vi "UHR-Fleezers Control (host) - 9.2.vi"() -> ()   [LabVIEW 2009]
uses:
  <vilib>/Utility/miscctls.llb/LVPoint32TypeDef.ctl
  <vilib>/Utility/miscctls.llb/LVMinMaxIncTypeDef.ctl
  <vilib>/userDefined/High Color/nirio_resource_hc.ctl
  <vilib>/Instr/_visa.llb/VISA Configure Serial Port (Instr).vi
  <vilib>/Platform/TimedLoop/XDataNode/XDataNode.xnode
  <vilib>/Platform/TimedLoop/XDataNode/loadlvalarms.vi
  <vilib>/Platform/TimedLoop/XDataNode/timing_clust.ctl
  <vilib>/Platform/TimedLoop/XDataNode/nitl_modes.ctl
  <vilib>/Platform/TimedLoop/XDataNode/wakeup.ctl
  <vilib>/rvi/interface/nirviOpenFPGA/nirviOpenFPGA.xnode
  FPGA Bitfiles/UHR-Fleezers Instr~3C_FPGA Target_UHR-Fleezers Contr~F0.lvbitx
  UHR-Fleezers Control (fpga) - 9.1.vi
  <vilib>/FPGAPlugInAG/PCIe-7852R/nirviIntfOpen_PCIe-7852R.vi
  <vilib>/rvi/interface/nirviMethod/nirviMethod.xnode
  <vilib>/Utility/error.llb/Merge Errors.vi
  <vilib>/LabVIEW Targets/FPGA/Rio/nirio_HostInterface/nirio_Reset.vi
  <vilib>/LabVIEW Targets/FPGA/Rio/nirio_HostInterface/nirio_DMAStopAll.vi
  <vilib>/rvi/interface/common/niFpgaNodeNameForErrorReporting.ctl
  <vilib>/rvi/errors/niLvFpgaWhatHappensToTopLevelVI.ctl
  <vilib>/LabVIEW Targets/FPGA/Rio/nirio_HostInterface/nirio_DisableInterrupts.vi
  <vilib>/Utility/error.llb/Error Cluster From Error Code.vi
  <vilib>/rvi/errors/niLvFpgaAdjustHostInterfaceError.vi
  <vilib>/rvi/interface/nirviReadWriteControl/nirviReadWriteControl.xnode
  <vilib>/LabVIEW Targets/FPGA/Rio/nirio_HostInterface/nirio_WriteBig.vi
  <vilib>/LabVIEW Targets/FPGA/Rio/nirio_HostInterface/nirio_DMAConfigure.vi
  <vilib>/LabVIEW Targets/FPGA/Rio/nirio_HostInterface/nirio_DMAStop.vi
  <vilib>/RVI Host/nirviSupport.llb/nirviErrorClusterFromErrorCode.vi
  <vilib>/LabVIEW Targets/FPGA/Rio/nirio_HostInterface/nirio_EnableInterrupts.vi
  <vilib>/rvi/errors/niLvFpgaReportInternalErrorWithAdditionalInfo.vi
  <vilib>/express/express analysis/Spectral/XNode/ExpressSpectralMeasurementsBlockNode.xnode
  <vilib>/express/express analysis/Spectral/Block/exnSpectralBlock spectral measurements PSD poly.vi
  <vilib>/express/express analysis/Spectral/Block/exnSpectralBlock spectral measurements PSD WFM.vi
  <vilib>/Waveform/WDTOps.llb/WDT Append Waveforms DBL.vi
  <vilib>/LabVIEW Targets/FPGA/Rio/nirio_HostInterface/nirio_ReadBig.vi
  <vilib>/vision/Avi1.llb/AviRefnum.ctl
  <vilib>/rvi/interface/nirviCloseFPGA/nirviCloseFPGA.xnode
  <vilib>/FPGAPlugInAG/PCIe-7852R/nirviIntfClose_PCIe-7852R.vi
  <vilib>/Analysis/NI_AALBase.lvlib
  <vilib>/Platform/TimedLoop/XDataNode/XDNodeRunTimeDep.lvlib
  openfpgaref.8.6.ctl
  NiRioSrv.dll
  <vilib>/vision/NI_Vision_Development_Module.lvlib
panel:
  out "Waveform Graph":dbl[](graph) caption="APD Line Scan"
  in  "Total Volume\nFlushed (uL)":dbl
  in  "Flush Center Channel":bool
  in  "Inject Bottom Channel":bool
  in  "Inject Top Channel":bool
  out "Messages":string
  in  "APD Ave N":dbl=10.0
  out "Int. Time (s)":dbl
  in  "Stop All":bool
  out "sigma/mean":dbl
  out "Rate sigma (Hz)":dbl format="%0.2f"
  out "Current Stage  Position":cluster{dbl, dbl, dbl}
  in  "Index":dbl=1.0 caption="Save File Index" min=1.0 step=1.0
  in  "Tab Control 6":T1(tab)=enum."Dual Display (APD)"
  out "All Signals":waveform(dbl)[](graph)
  in  "Signals to Plot":i32(listbox)
  out "Trap Disp. Freq. (Hz)":dbl caption="Freq. (Hz)" format="%#_6p"
  out "Display Period (s)":dbl caption="Period (s)" format="%#_6p"
  in  "Trap Disp. Downsample":dbl=20000.0 caption="Downsample"
  in  "APD Disp. Scale":dbl=0.1 caption="Scale (Divide,\nfor above plot only)"
  in  "APD Disp. Downsample":dbl=30.0 caption="Integrate" min=1.0 step=1.0
  out "APD Display Freq. (Hz)":dbl caption="Freq. (Hz)"
  out "APD Display Period (s)":dbl caption="Period (s)"
  out "RMS (Ang)":dbl format="%_2g"
  in  "Bead Sep. Int. Time (s)":dbl=5.0 caption="Int. Time (s)"
  in  "Below (kHz)":dbl=0.5
  in  "Above (kHz)":dbl=2.0
  in  "Adjust Scale\nto Mean":bool
  in  "Rescale on Mean":bool
  in  "Offset (nm)":dbl
  out "Mean":dbl caption="Mean (pN)" format="%#_3g"
  out "Force":waveform(dbl)[](graph)
  out "APD 1 Chart":waveform(dbl)(graph)
  in  "Calibration":u16(ring)=2 items=["None", "Position", "Force"]
  out "T1 X":dbl caption="T1 X (pN)" format="%0.2f"
  out "T2 X":dbl caption="T2 X (pN)" format="%0.2f"
  out "Bead Separation":waveform(dbl)(graph)
  in  "Amplitude (nm)":dbl=1.0
  out "Bead Mean (nm)":dbl caption="Mean (nm)" format="%0.2f"
  out "Difference":dbl caption="Difference (pN)" format="%.2g"
  in  "Set X Only":bool
  in  "Set Y Only":bool
  out "Detection Laser X":T2(plugin-control)
  out "APD 1":T2(plugin-control)
  out "Detection Laser Y":T2(plugin-control)
  out "Pointer Y (V)":dbl format="%_3g"
  out "Pointer X (V)":dbl format="%_3g"
  in  "Set Confocal Spot (X-Y)":bool
  out "FFT 1":cluster{"f0":dbl, "df":dbl, "magnitude":dbl[]}[](graph)
  out "FFT 2":cluster{"f0":dbl, "df":dbl, "magnitude":dbl[]}[](graph)
  in  "FFT 1 Choice 1":u16(ring) items=["T1 Y", "T1 X", "T1 Sum", "T2 Y", "T2 X", "T2 Sum", "T1 FB X", "T1 FB Sum", "T2 FB X", "T2 FB Sum", "PSD Y", "PSD X", "PSD Y Sum", "none"]
  in  "FFT 2 Choice 1":u16(ring)=13 items=["T1 Y", "T1 X", "T1 Sum", "T2 Y", "T2 X", "T2 Sum", "T1 FB X", "T1 FB Sum", "T2 FB X", "T2 FB Sum", "PSD Y", "PSD X", "PSD Y Sum", "none"]
  in  "FFT 1 Choice 2":u16(ring)=1 items=["T1 Y", "T1 X", "T1 Sum", "T2 Y", "T2 X", "T2 Sum", "T1 FB X", "T1 FB Sum", "T2 FB X", "T2 FB Sum", "PSD Y", "PSD X", "PSD Y Sum", "none"]
  in  "FFT 2 Choice 2":u16(ring)=13 items=["T1 Y", "T1 X", "T1 Sum", "T2 Y", "T2 X", "T2 Sum", "T1 FB X", "T1 FB Sum", "T2 FB X", "T2 FB Sum", "PSD Y", "PSD X", "PSD Y Sum", "none"]
  in  "Compute FFT":bool
  in  "Reset FFT":bool
  in  "# Spectra to Ave.":dbl=100.0
  out "Ave. Time (s)":dbl
  out "1 Channel":waveform(dbl)(graph)
  out "Slow mean":dbl format="%0.2f"
  in  "Slow mean N ave.":dbl=1.0 min=1.0 step=1.0
  out "Mean Intensity":dbl
  out "Sigma":dbl
  out "Sigma/Mean":dbl
  in  "Subtract mean":bool
  in  "High Res. Display":u16(ring) items=["T1 Y", "T1 X", "T1 Sum", "T2 Y", "T2 X", "T2 Sum", "T1 FB X", "T1 FB Sum", "T2 FB X", "T2 FB Sum", "PSD Y", "PSD X", "PSD Y Sum"]
  out "APD 1 Graph":dbl[](graph) caption="Most Recent Time Trace"
  out "Trap Delta Graph":dbl[](graph) caption="Most Recent Time Trace"
  out "APD 1 Rate (Hz)":dbl format="%#_3p"
  out "Image":u32[][](graph)
  in  "Tab Control":T3(tab)=enum."APD Counting"
  in  "Read Cal":bool
  out "Tether":bool
  in  "Tether Alarm?":bool=TRUE
  in  "Move to Delta (MHz)":dbl=14.5
  in  "Then...":string(combo)="2"
  in  "Data Acq. Spot":bool
  out "Fl. High":bool
  out "Waiting":bool
  in  "Yank to Freq. (MHz)":dbl
  in  "Fl. Threshold (kHz)":dbl
  in  "Fl. Triggered...":bool
  in  "Confocal Linescan":bool
  in  "Speed (nm/s)":dbl=100.0
  in  "Stop F (pN)":dbl=2.0
  in  "Furthest Withdraw (MHz)":dbl=15.0
  in  "Closest Delta (MHz)":dbl=10.25 step=0.25
  in  "Fish for Tether":bool
  in  "Confocal Image":bool
  in  "Round T1 X":bool caption="Round"
  in  "T1 offset_x (mV)":dbl=-26.302542012392074 format="%#_2g"
  in  "T1 kappa_x (pN/nm)":dbl=0.22546432407642192 min=0.0 step=0.001 format="%#_2g"
  out "Time (s)":dbl
  out "Total Time (s)":dbl
  in  "Start Saving":bool
  in  "Limits Enable":bool=TRUE caption="Enable"
  in  "Limit Max (MHz)":dbl=16.0 caption="Max (MHz)"
  in  "Limit Min (MHz)":dbl=10.0 caption="Min (MHz)"
  in  "Cal sets to save":u32=50 min=1 step=1
  in  "Comment (data description)":string="testing confocal setup"
  out "Calibrating Trap...":bool
  in  "Trap 2 (ON/OFF)":bool
  in  "Trap 1 (ON/OFF)":bool
  in  "Save Calibration":bool
  in  "N sets to save":u32=200 caption="N Sets"
  in  "Save N Sets":bool
  out "Save file name":path
  in  "Save ave N":dbl=500.0 caption="Averaging Factor"
  out "Saving...":bool
  in  "Stop Saving":bool
  out "Progress":u16(slide) scale=0.0..100.0
  out "Manipulating Trap":bool
  out "Buffer Status":dbl(slide) scale=0.0..1.0
  out "Overflow (data lost)":bool
  in  "Reset":bool
  out "Data Rate (Hz)":dbl caption="Trap Data Rate (Hz)" format="%#_3p"
  out "Data Period (s)":dbl caption="Trap Data Period (s)" format="%#_6p"
  out "Save Data Rate (Hz)":dbl caption="Rate (Hz)" format="%#_6p"
  out "Save Data Period (s)":dbl caption="Period (s)" format="%#_6p"
  in  "T1 alpha_x (nm/V)":dbl=630.439304367558 step=10.0 format="%#_3g"
  in  "T2 alpha_x (nm/V)":dbl=704.7738222964198 step=10.0 format="%#_3g"
  in  "T2 kappa_x (pN/nm)":dbl=0.2030110880477556 min=0.0 step=0.001 format="%#_2g"
  in  "T2 offset_x (mV)":dbl=-26.67973517613748 format="%#_2g"
  in  "BD 1 Frequency 1 (MHz)":dbl=70.5 caption="T1 X (MHz)" min=60.0 max=90.0 step=1.0 format="%#_6p"
  in  "BD 1 Frequency 2 (MHz)":dbl=85.0 caption="T2 X (MHz)" min=60.0 max=90.0 step=1.0 format="%#_6p"
  in  "Green Laser ON/Interlacing":bool
  in  "Round T2 X":bool caption="Round"
  in  "AO1":dbl(slide)=5.47 caption="Confocal Y (V)" min=0.0 max=10.0 step=0.01 scale=0.0..10.0 scale format="%_1f"
  in  "AO2":dbl(slide)=4.15 caption="Confocal X (V)" min=0.0 max=10.0 step=0.01 scale=0.0..10.0 scale format="%_1f"
  in  "Upper Cap.":bool
  in  "Lower Cap.":bool
  in  "Trap Raster Scan":bool
  out "Raster Scanning...":bool
  in  "Trap Delta (MHz)":dbl=14.5
  in  "Action":string(combo)="Alarm"
  in  "Dump Beads":bool
  out "Duration (s)":dbl
  out "Stage Moving":bool
  in  "Wait Before Save (s)":u32=1
  out "Attempts":dbl
  in  "Attempt Limit":dbl=20.0 caption="Limit"
  in  "z nudge increment (um)":dbl=0.5
  in  "+z":bool
  in  "Saved Stage Positions":T4={"Position 1"={1.35171, -1.39824, -0.01733}, "Position 2"={0.0, 0.0, 0.0}, "Position 3"={2.99911, -0.2477, 0.0}, "Position 4"={2.1058, 0.57485, 0.0}} {"Position 1"."?" min=-0.1 max=0.1 step=0.1; "Position 2"."?" min=-0.1 max=0.1 step=0.1; "Position 3"."?" min=-0.1 max=0.1 step=0.1; "Position 4"."?" min=-0.1 max=0.1 step=0.1}
  in  "Position 1 Label":string="Upper capillary"
  in  "Set Position 1":bool
  in  "Set Position 2":bool
  in  "Set Position 3":bool
  in  "Set Position 4":bool
  in  "Move to Position 3":bool
  in  "Move to Position 4":bool
  in  "Move to Position 2":bool
  in  "Move to Position 1":bool
  in  "Position 2 Label":string="Lower capillary"
  in  "Position 3 Label":string="Measurement Spot"
  in  "Position 4 Label":string="Dump beads"
  in  "-z":bool
  in  "Top Ch Inject Rate (ul/h)":dbl=10.0
  in  "Pump write delay (ms)":dbl=300.0
  in  "All Pump Parameters":T5={"Pump 1"={"Diameter (mm)"=4.61, "Units"=3.0, "Volume"=0.0, "Rate"=0.0}, "Pump 2"={"Diameter (mm)"=4.61, "Units"=3.0, "Volume"=0.0, "Rate"=0.0}, "Pump 3"={"Diameter (mm)"=4.61, "Units"=3.0, "Volume"=0.0, "Rate"=0.0}}
  in  "Top Ch Inject Volume (uL)":dbl=100.0
  in  "Pump pause delay (ms)":u32
  in  "Bottom Ch Inject Volume (uL)":dbl=100.0
  in  "Bottom Ch Inject Rate (ul/h)":dbl=10.0
  in  "Flush Center Ch Volume (uL)":dbl=15.0
  in  "Flush Center Ch Rate (ul/m)":dbl=100.0
  in  "Tab Control 2":T6(tab)=enum."AOD Raster Scan"
  out "Total Counts (ticks)":u32
  in  "Trap ON/OFF X or Y Amp?":bool=TRUE
  in  "Oscillate Set 1":bool
  in  "Trap 1 ON":bool
  in  "Number Interlace Sets":u8=3 min=1 max=3
  in  "DIO count 3 (ticks)":u32=200
  in  "DIO count 2 (ticks)":u32=200
  in  "DIO count 1 (ticks)":u32=200
  in  "BD 2 Amplitude 3 (%)":dbl min=0.0 max=50.0 step=1.0
  in  "BD 2 Amplitude 2 (%)":dbl min=0.0 max=50.0 step=1.0
  in  "BD 2 Amplitude 1 (%)":dbl min=0.0 max=50.0 step=1.0
  in  "BD 1 Amplitude 3 (%)":dbl min=0.0 max=50.0 step=1.0
  in  "BD 1 Amplitude 2 (%)":dbl=35.0 min=0.0 max=50.0 step=1.0
  in  "BD 1 Amplitude 1 (%)":dbl=10.0 min=0.0 max=50.0 step=1.0
  in  "BD 2 Frequency 3 (MHz)":dbl=26.0 min=0.0 max=40.0 step=1.0 format="%#_6p"
  in  "BD 1 Frequency 3 (MHz)":dbl=70.0 min=60.0 max=90.0 step=1.0 format="%#_6p"
  in  "BD 2 Frequency 2 (MHz)":dbl=26.0 min=0.0 max=40.0 step=1.0 format="%#_6p"
  in  "BD 2 Frequency 1 (MHz)":dbl=26.0 min=0.0 max=40.0 step=1.0 format="%#_6p"
  in  "Not-Interlacing Set":enum32{"Set 1", "Set 2", "Set 3"}(radio)
  in  "Interlace":bool=TRUE
  in  "Trap 2 ON":bool
  in  "Trap 3 ON":bool
  in  "Scan axis 2":bool=TRUE
  in  "Osc. freq. (Hz)":dbl=0.25
  in  "Osc. amp. (MHz)":dbl=2.0
  out "Coords":T7
  in  "Manipulation Scaling":cluster{"Horizontal":dbl, "Vertical":dbl}={"Horizontal"=0.075, "Vertical"=0.01}
  in  "Freq or Amp switch first":bool=TRUE
  in  "Swap F1 and F2":bool
  in  "Freq switch delay":u16
  in  "Amp switch delay":u16=5
  in  "MCL Step Increment (V_int)":dbl=3.0
  out "Time to Finish All (min)":dbl format="%#_2p"
  in  "Scan Speed (nm/s)":dbl=100.0
  in  "Scan Range (nm)":dbl=600.0
  in  "Step Size (nm)":dbl=1.0
  in  "MCL/AOM Scale Tweak":dbl=1.0
  in  "MCL Step Position Ratio":dbl=0.5
  in  "Move MCL Also?":bool=TRUE
  out "Final sep (nm)":dbl
  out "Initial sep (nm)":dbl
  out "Save index":dbl
  out "Final delta (MHz)":dbl
  out "Initial delta (MHz)":dbl
  out "Final freq. (MHz)":dbl
  out "Initial freq. (MHz)":dbl
  in  "Saved AOD Raster Scan Parameter Sets":T8(array[cluster])=[{"Scan Range AOD (nm) 2"=500.0, "Step Size AOD (nm) 2"=1.0, "Scan Speed AOD (nm/s) 2"=200.0, "Number of scans (AOD) 2"=1, "Label"=""}, {"Scan Range AOD (nm) 2"=1000.0, "Step Size AOD (nm) 2"=1.0, "Scan Speed AOD (nm/s) 2"=200.0, "Number of scans (AOD) 2"=5, "Label"="wide offset scan"}, {"Scan Range AOD (nm) 2"=20.0, "Step Size AOD (nm) 2"=0.68, "Scan Speed AOD (nm/s) 2"=0.68, "Number of scans (AOD) 2"=1, "Label"="2 bp steps"}]
  in  "Load parameters":bool
  out "Scan Range (MHz)":dbl=10.0
  in  "Restart DMA? (AOD)":bool=TRUE caption="Restart DMA?"
  out "Incr. int (AOD)":i64
  out "Time/Scan (s) (AOD)":dbl format="%#_2p"
  out "Data points/scans":dbl
  out "Data points/scan (f/b)":dbl
  in  "Save scans":bool=TRUE
  out "AOD Scan I":u64 caption="Scan I"
  in  "Continuous AOD Scanning":bool caption="Continuous Scanning"
  in  "Abort AOD Scan":bool caption="Abort Scan"
  in  "Scan BD":bool=TRUE
  out "Cycles/step (AOD)":u64=400 format="%.0p"
  in  "Number of F/B Scans (AOD)":u16=3 min=1
  out "Scan steps (AOD)":u64=1000
  out "Scan Increment (MHz)":dbl=0.2
  out "AOD Scanning":bool caption="Scanning"
  in  "Start AOD Scan":bool caption="Start Scan"
  out "N sets should be saved":dbl
  out "Progress 2":u16(slide) caption="Progress" scale=0.0..100.0
  in  "Abort save 2":bool caption="Abort save"
  in  "Trap 1 Bead Size (nm)":dbl=860.0
  in  "Trap 2 Bead Size (nm)":dbl=790.0
  out "MCL Count":dbl
  in  "All FB On/Off":bool=TRUE
  in  "AI2 to Setpoint":cluster{"Set 1":bool, "Set 2":bool}
  out "AI2 (V)":cluster{"Set 1":dbl, "Set 2":dbl}
  in  "Reset Feedback":cluster{"Set 1":bool, "Set 2":bool}
  in  "PID Gains":T9={"Set 1"={"proportional gain (Kc)"=0, "integral gain (Kc*Ts/Ti)"=5, "derivative gain (Kc*Td/Ts)"=0}, "Set 2"={"proportional gain (Kc)"=0, "integral gain (Kc*Ts/Ti)"=5, "derivative gain (Kc*Td/Ts)"=0}}
  in  "Setpoints (V)":cluster{"Set 1":dbl, "Set 2":dbl}={"Set 1"=7.0, "Set 2"=7.0}
  in  "Feedback On/Off":cluster{"Set 1":bool, "Set 2":bool}={"Set 1"=TRUE, "Set 2"=TRUE}
  in  "Tab Control 3":enum32{"Timing", "MCL Scan", "Analog Out"}(tab)
  out "APD Gate Late Counter":u32
  in  "- phase (APD Gate)":bool
  in  "+ phase (APD Gate)":bool
  out "APD Gate Relative Phase":i16
  in  "Phase Adj. (APD Gate)":i16=20
  in  "Initial Phase Adjustment (APD Gate)":i16=50
  in  "Save APD Data\nwith Trap Data":bool=TRUE
  out "APD FIFO Elements Remaining":u32
  in  "- phase (APD Acq)":bool
  in  "+ phase (APD Acq)":bool
  out "APD Acq Late Counter":u32
  out "APD Acq Relative Phase":i16
  in  "Phase Adj. (APD Acq)":i16=20
  in  "Initial Phase Adjustment (APD Acq)":i16
  in  "Invert APD Gate":bool caption="Invert Gate"
  in  "APD Gate OFF Count":u32=450 caption="Gate OFF Count"
  in  "APD Gate ON Count":u32=150 caption="Gate ON Count"
  in  "APD Gate":enum32{"ON", "OFF", "Interlace"}(radio)=enum."Interlace"
  in  "APD Integration Time (s)":dbl=0.01 caption="Integration Time (s)"
  out "APD Acq Rate (Hz)":dbl=20000000.0 caption="Rate (Hz)"
  out "APD Samples/FIFO Acq.":dbl
  out "APD Elements/DMA read":u32
  out "APD Int. Count":u32 format="%.0p"
  in  "Tab Control 5":enum32{"PSD X", "PSD Y", "Other Data Channel"}(tab)
  out "Data map":dbl[][](graph)
  in  "Channel":i32=4
  in  "Abort MCL Scan":bool
  out "MCL Scan I":u64
  out "MCL Scanning":bool
  in  "Start MCL Scan":bool
  out "wait to reset values":bool
  in  "Tab Control 4":enum32{"Scan Settings", "MCL FPGA Loop Timing"}(tab)=enum."MCL FPGA Loop Timing"
  out "Total Time (s)":dbl
  in  "Scan lines (y)":u64=10
  in  "Fast Scan Dir":bool=TRUE
  in  "2D or 1D Scan":bool=TRUE
  out "Initial X":dbl
  out "Initial Y":dbl
  out "Time/f+b scan (s) (MCL)":dbl caption="Time/scan (s)"
  in  "Number of scans (MCL)":u64=1 caption="Scans"
  in  "Scan steps (MCL)":u64=20 caption="Scan steps (x)"
  in  "N APD Samp/step":dbl=6.0
  in  "Scan Range (V)\n(of steps)":dbl=3.5
  in  "Restart DMA? (MCL)":bool=TRUE caption="Restart DMA?"
  in  "Continuous MCL Scanning":bool caption="Cont. Scanning"
  in  "Center Scan":bool=TRUE
  in  "Save Data (MCL)":bool=TRUE caption="Save Data"
  out "Actual Incr. int (MCL)":i16 caption="Incr. int"
  out "Desired incr (int)":dbl
  out "Desired Scan Incr (V)":dbl
  out "N sets should be saved (MCL)":dbl caption="N sets should be saved"
  out "Data points/scans (MCL)":dbl caption="Data points/scans"
  out "Data points/scan (f+b)":dbl caption="points/scan (f+b)"
  out "Cycles/step (MCL)":u64 caption="Cycles/step" format="%.0p"
  out "Actual MCL Inc (V)":dbl
  in  "Phase adjust (MCL)":i16 caption="Phase adjust"
  out "Relative Phase (MCL)":i16 caption="Relative Phase"
  in  "Initial Phase Adj. (MCL)":i16 caption="Initial Phase Adj."
  in  "Update Count (MCL)":u32=600
  in  "+ phase (MCL)":bool
  in  "- phase (MCL)":bool
  out "MCL Late Counter":u32
  in  "APD 1 AO Mult.":i16=1 min=1
  in  "APD 2 AO Mult.":i16=1 min=1
  in  "APD 1 AO offset":i16
  in  "APD 2 AO offset":i16
  in  "Tab Control 7":enum32{"Green FB Signals", "Slow MCL Scan"}(tab)
  out "Green FB Plot":dbl(graph)
  out "MCL Scan 2":cluster{"Begin (V)":dbl, dbl, dbl[]}(graph)
  out "MCL Scan":cluster{"Begin (V)":dbl, dbl, dbl[]}(graph)
  in  "Green laser mode":enum32{"Laser ON", "Laser OFF", "Interlace"}(radio)=enum."Interlace"
  in  "GI Frequency, ON count":u32=150 min=1 step=1
  in  "Invert GI":bool
  out "GI Late Counter":u32
  in  "Phase adj. (GI)":i16=5
  out "GI relative phase":i16
  in  "+ phase (GI)":bool
  in  "Initial Phase Adjustment (GI)":i16=15
  in  "GI Frequency, OFF count":u32=450 min=1 step=1
  in  "- phase (GI)":bool
  out "Green FB Signals (V)":cluster{"Y":dbl, "X":dbl, "Sum":dbl}
  out "Relative phase (Green FB)":i16
  in  "+ phase (Green FB)":bool
  in  "- phase (Green FB)":bool
  in  "Green FB Count":u32=600
  in  "Phase adj. (Green FB)":i16=10
  in  "Initial Phase Adjustment (Green FB)":i16=50
  in  "Green FB On/Off":bool=TRUE
  in  "Current When FB OFF (%)":dbl=65.0 min=0.0 max=100.0 step=1.0
  in  "Green int current ON count adj":u32=150
  in  "Green FB Gains":T10={"proportional gain (Kc)"=10, "integral gain (Kc*Ts/Ti)"=5, "derivative gain (Kc*Td/Ts)"=0}
  in  "Green FB Setpoint (mV)":dbl=100.0
  in  "- phase (GI) 2":bool
  in  "Initial Phase Adjustment (GI) 2":i16=-100
  in  "+ phase (GI) 2":bool
  out "GI relative phase 2":i16
  in  "Phase adj. (GI) 2":i16=20
  out "GI Late Counter 2":u32
  in  "# Samples/trap":dbl=20000.0 format="%#_6p"
  out "Elements/DMA read":u32 format="%.0p"
  out "Ave. Rate (Hz)":dbl format="%#_6p"
  out "FIFO El. Rem.":u32 format="%.0p"
  in  "Phase adj. (AI1)":i16=15
  out "Relative phase (AI1)":i16
  in  "+ phase (AI1)":bool
  in  "- phase (AI1)":bool
  out "Late Counter (AI1)":u32
  in  "Initial Phase Adjustment (AI1)":i16=220
  out "AI rate (Hz)":dbl=50000.0 format="%#_6p"
  in  "AI Count (ticks)":u32=200
  out "# Samples/channel":u32=20000 format="%.0p"
  in  "FIFO Depth":u32=600000 format="%.0p"
  in  "Detector Type":string(combo)="IR-QPD + PSD + FB-QPD X position"
  in  "N Acq Sets (Traps + Fl.)":i16=3
  in  "Sets to FIFO (Traps)":T11={"Set 1"=TRUE, "Set 2"=TRUE, "Set 3"=FALSE}
  in  "FPGA Ave.":dbl=1.0 min=1.0 step=1.0
  out "Ave. Period (s)":dbl format="%#_6p"
  out "DMA Update Period (s)":dbl
  out "FPGA Averaging":bool
  out "Trap Sets":i16
  out "Counts/DMA":dbl format="%#_6p"
  in  "Video Capture Rate (Hz)":dbl=30.0
  in  "Video Index":dbl=1.0 min=1.0 step=1.0
  in  "New Video File":bool
  in  "Capture Video":bool
  in  "Reset Averaging":bool
  in  "Averaging":bool
  in  "Capture and Save Image":bool
  in  "Image Index":dbl=1.0 min=1.0
  out "Path Out":path
  in  "Center Point":cluster{"X":i32, "Y":i32}={"X"=341, "Y"=253}
  in  "Zoom Factor":sgl=4.0
  out "Window Size":cluster{"Width":i32, "Height":i32}
  out "Window Position":cluster{"X Position":i32, "Y Position":i32}={"X Position"=40, "Y Position"=40}
  in  "Initial Window Size":cluster{"Width":i32, "Height":i32}={"Width"=884, "Height"=619}
  in  "Initial Window Position":cluster{"X Position":i32, "Y Position":i32}={"X Position"=796, "Y Position"=4}
  in  "Intensity Upper":u8=88
  in  "Intensity Lower":u8=66
  out "error out":errorcluster
  out "error out 2":errorcluster
  in  "Lost Tether Alarm Threshold (pN)":dbl=0.5
  in  "AOM X Cal (nm/MHz)":dbl=123.0
  in  "MCL X Cal (nm/V)":dbl=1070.0
  out "X RF Amplitude Limits (%)":T12={"Minimum"=0.0, "Maximum"=50.0, "Increment"=1.0}
  out "X RF Frequency Limits (MHz)":T12={"Minimum"=60.0, "Maximum"=90.0, "Increment"=1.0}
  out "Y RF Frequency Limits (MHz)":T12={"Minimum"=60.0, "Maximum"=90.0, "Increment"=1.0}
  out "Y RF Amplitude Limits (%)":T12={"Minimum"=0.0, "Maximum"=50.0, "Increment"=1.0}
  in  "Manip. X?":bool=TRUE
  in  "Manip. Y?":bool
  in  "Force Manip Abort":bool
  out "Read cal error":errorcluster
  in  "DAQ Delay (ms)":u32=1000
  in  "Start Scan":bool
  in  "Scan axis":bool=TRUE
  in  "Osc. amp. (V)":dbl=5.0
  in  "Osc. center (V)":dbl=5.0
  in  "Osc. freq. (Hz) 2":dbl=1.0
  in  "MCL Mode":u16(ring) items=["Manual Positioning", "Sinusoidal Wave", "Linear Scan"]
  in  "Begin (V)":dbl
  in  "End (V)":dbl=10.0
  in  "N Points":dbl=20.0
  in  "Delay to Interlace (s)":dbl
  in  "Delayed Interlace Start":bool
  in  "Read Lateness and Rel Phase":bool
  out "Vec Mean of T1 T2":dbl[](array[numeric])
  in  "Cal read wait (s)":u32=5
  out "Time tether formed":timestamp
  in  "Sample Chamber Stage Serial Port":refnum<visa-resource-name>="COM5"
  in  "Syringe Pump Serial Port":refnum<visa-resource-name>="COM4"
  # "Trap Display:"
  # "APD Display:"
  # "DAQ"
  # "Move Stage and Take Action"
  # "Trap Manipulation"
  # "Data Saving"
  # "Bead Calibration"
  # "Trap Position Difference Limits"
  # "Center channel"
  # "Units: \n1 = ml/m\n2 = ml/h\n3 = ul/m\n4 = ul/h"
  # "Rate param is ul/h\nVolume param is ul"
  # "X"
  # "Y"
  # "Oscillate Set 1 freq. (debugging)"
  # "BD 1"
  # "BD 2"
  # "AOD Raster Scan"
  # "Approx. trap separations"
  # "X"
  # "Y"
  # "Gate"
  # "X"
  # "2D"
  # "Y"
  # "1D"
  # "Green Laser Interlacing"
  # "Green FB Measurement"
  # "Digital Gate"
  # "Current Analog Control"
  # "Total AI Rates (NOT rates/trap)"
  # "(Samples/trap x Trap Sets)"
  # "(Samples/channel x\n8 if averaging (8 channels)\n4 if no averaging)"
  # "Trap 1"
  # "Trap 2"
  # "Flour./Trap 3"
  # "External Video Window"
  # "MCL Position Debugging"
  # "Temporary Control Storage\n(these used to be somewhere else, still want to keep them)"
  # "Y"
  # "X"
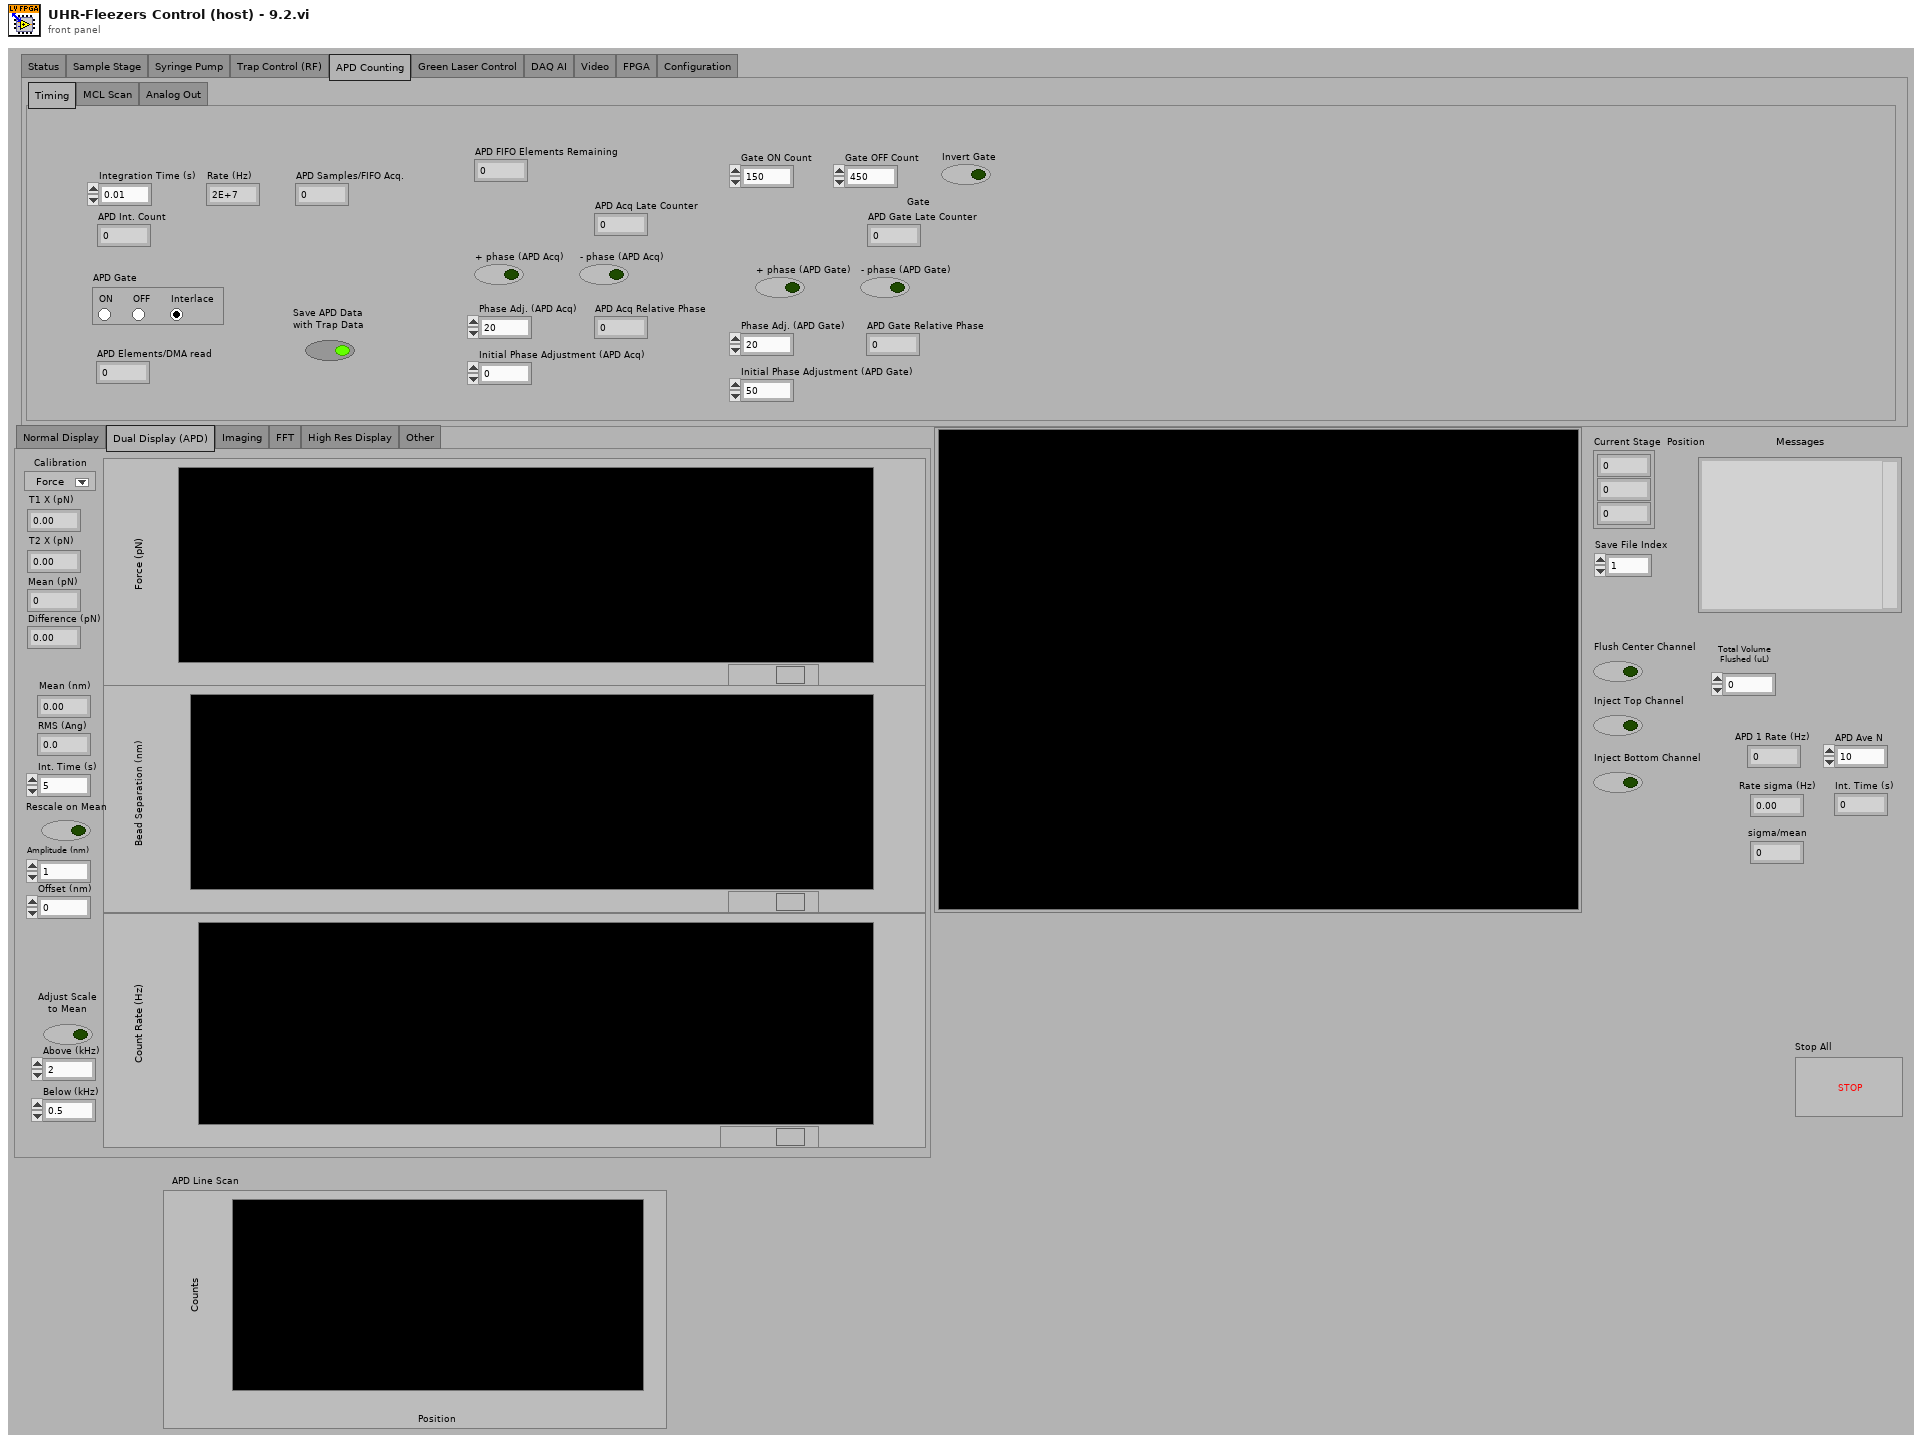
[diagram p1: front panel]
types:
  T1 = enum32{"Normal Display", "Dual Display (APD)", "Imaging", "FFT", "High Res Display", "Other"}
  T2 = typedef "IMAQ Image.ctl" = refnum<image>
  T3 = enum32{"Status", "Sample Stage", "Syringe Pump", "Trap Control (RF)", "APD Counting", "Green Laser Control", "DAQ AI", "Video", "FPGA", "Configuration"}
  T4 = cluster{"Position 1":cluster{dbl, dbl, dbl}, "Position 2":cluster{dbl, dbl, dbl}, "Position 3":cluster{dbl, dbl, dbl}, "Position 4":cluster{dbl, dbl, dbl}}
  T5 = cluster{"Pump 1":cluster{"Diameter (mm)":dbl, "Units":dbl, "Volume":dbl, "Rate":dbl}, "Pump 2":cluster{"Diameter (mm)":dbl, "Units":dbl, "Volume":dbl, "Rate":dbl}, "Pump 3":cluster{"Diameter (mm)":dbl, "Units":dbl, "Volume":dbl, "Rate":dbl}}
  T6 = enum32{"IR Laser Interlacing (Direct RF Board Control Method)", "AOD Raster Scan", "Feedback on BD 1 Amp to Control AI2"}
  T7 = typedef "LVPoint32TypeDef.ctl" = cluster{"Horizontal":i32, "Vertical":i32}
  T8 = cluster{"Scan Range AOD (nm) 2":dbl, "Step Size AOD (nm) 2":dbl, "Scan Speed AOD (nm/s) 2":dbl, "Number of scans (AOD) 2":u16, "Label":string}[]
  T9 = cluster{"Set 1":cluster{"proportional gain (Kc)":i16, "integral gain (Kc*Ts/Ti)":i16, "derivative gain (Kc*Td/Ts)":i16}, "Set 2":cluster{"proportional gain (Kc)":i16, "integral gain (Kc*Ts/Ti)":i16, "derivative gain (Kc*Td/Ts)":i16}}
  T10 = cluster{"proportional gain (Kc)":i16, "integral gain (Kc*Ts/Ti)":i16, "derivative gain (Kc*Td/Ts)":i16}
  T11 = cluster{"Set 1":bool, "Set 2":bool, "Set 3":bool}
  T12 = typedef "LVMinMaxIncTypeDef.ctl" = cluster{"Minimum":dbl, "Maximum":dbl, "Increment":dbl}
  T13 = typedef "Image Type" = u32
  T14 = typedef "nirio_resource_hc.ctl" = tag
  T15 = typedef "openfpgaref.8.6.ctl" = refnum<k20>
  T16 = typedef "niFpgaNodeNameForErrorReporting.ctl" = enum16{"Open FPGA VI Reference", "Read/Write Control", "Invoke Method: Abort", "Invoke Method: Acknowledge IRQ", "Invoke Method: Download", "Invoke Method: FIFO.Configure", "Invoke Method: FIFO.Read", "Invoke Method: FIFO.Start", "Invoke Method: FIFO.Stop", "Invoke Method: FIFO.Write", "Invoke Method: Reset", "Invoke Method: Run", "Invoke Method: Wait on IRQ", "Close FPGA VI Reference"}
  T17 = typedef "niLvFpgaWhatHappensToTopLevelVI.ctl" = enum16{"top level VI scripted behind XNode", "top level VI inlined behind XNode"}
  T18 = typedef "XDNodeRunTimeDep.lvlib/timing_clust.ctl" = cluster{"Expected End [f-1]":u64, "Actual End [f-1]":u64, "Finished Late? [f-1]":bool, "Expected End [i-1]":u64, "Actual End [i-1]":u64, "Finished Late? [i-1]":bool, "Expected Start [i]":u64, "Actual Start [i]":u64, "Expected Start [f]":u64, "Actual Start [f]":u64, "Source Name":string, "Structure Name":string, "Period":i64, "Deadline":i64, "Offset":i64, "Start":i64, "Priority":i32, "Timeout":i32, "Mode":T19, "Wakeup Reason":T20, "Error":errorcluster, "Source Type":string, "Secondary Source Type":string, "Global End Time":u64, "Global Start Time":u64, "Frame Duration":u64, "Iteration Duration":u64, "Assigned CPU":i32, "I/O Scan Engine Mode":u32}
  T19 = typedef "XDNodeRunTimeDep.lvlib/nitl_modes.ctl" = enum32{"No Change", "Process missed periods, maintain original phase", "Discard missed periods, maintain original phase", "Process missed periods, ignore original phase", "Discard missed periods, ignore original phase"}
  T20 = typedef "XDNodeRunTimeDep.lvlib/wakeup.ctl" = enum32{"Normal", "Aborted", "Asynchronous wakeup", "Timing source error", "Timed loop error", "Timeout"}
  T21 = enum32{"setting", "request", "request control", "info", "statistics", "system settings", "I/O sub system", "HRT control", "camera descriptions", "device specific data", "event sub system settings", "event sub system results", "image memory manager"}
  T22 = typedef "AviRefnum.ctl" = refnum<k1>
  T23 = typedef "imagedata.ctl" = cluster{"image type":i32, "image depth":i32, "image":u8[], "mask":u8[], "colors":u32[], "Rectangle":cluster{"left":i16, "top":i16, "right":i16, "bottom":i16}}
  T24 = enum16{"big-endian, network order", "native, host order", "little-endian"}
  T25 = enum16{"open", "replace", "create", "open or create", "replace or create", "replace or create with confirmation"}
  T26 = cluster{"Scan Range AOD (nm) 2":dbl, "Step Size AOD (nm) 2":dbl, "Scan Speed AOD (nm/s) 2":dbl, "Number of scans (AOD) 2":u16, "Label":string}
  T27 = cluster{"[0]":dbl, "[1]":dbl, "[2]":dbl, "[3]":dbl, "[4]":dbl, "[5]":dbl}
  T28 = cluster{"Diameter (mm)":dbl, "Units":dbl, "Volume":dbl, "Rate":dbl}
  T29 = enum32{"Normal Display", "Dual Display (APD)", "FFT", "High Res Display"}
  T30 = cluster{"Origin Pixel":cluster{"X":sgl, "Y":sgl}, "Angle Relative to Horizontal (deg)":sgl, "Axis Reference":u32}
  T31 = typedef "Simple Grid Descriptor" = cluster{"X Step":sgl, "Y Step":sgl, "Unit":T32}
  T32 = typedef "Image Unit" = enum32{"Undefined", "Angström", "Micrometer", "Millimeter", "Centimeter", "Meter", "Kilometer", "Microinch", "Inch", "Feet", "Nautical miles", "Standard miles", "Steps"}
  T33 = cluster{"averaging mode":u16, "weighting mode":u16, "number of averages":u32}
  T34 = cluster{"dB On (F)":bool, "unwrap phase (F)":bool, "convert to degree (F)":bool}
  T35 = cluster{"Green FB Ch 0":i16, "Green FB Ch 1":i16, "Green FB Ch 2":i16}
  T36 = cluster{string, string, string, string, string, string, string, string}
  T37 = cluster{string, string, string, string, string, string, string, string, string, string, string, string}
  T38 = cluster{string, string, string, string, string, string, string, string, string, string, string, string, string}
  T39 = cluster{string, string, string, string, string, string, string, string, string, string, string, string, string, string}
  T40 = cluster{"f0":dbl, "df":dbl, "magnitude":dbl[]}[][]
  T41 = cluster{"Green FB Ch 0":dbl, "Green FB Ch 1":dbl, "Green FB Ch 2":dbl}
  T42 = cluster{"Left":i32, "Top":i32, "Width":u32, "Height":u32}
  T43 = cluster{cluster{"Left":i32, "Top":i32, "Width":u32, "Height":u32}}[]
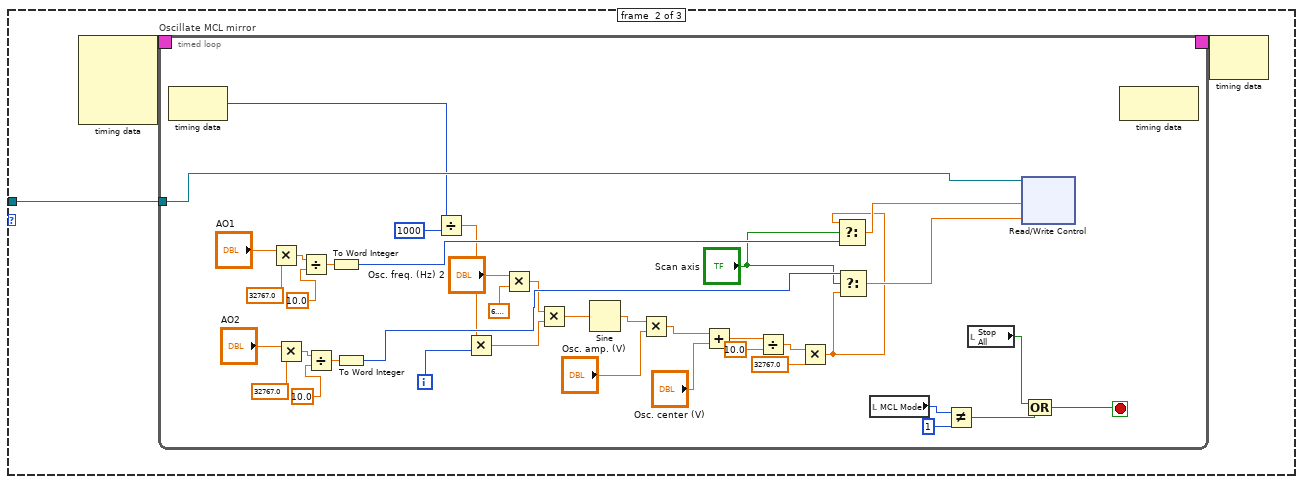
[diagram p2: hidden frame]
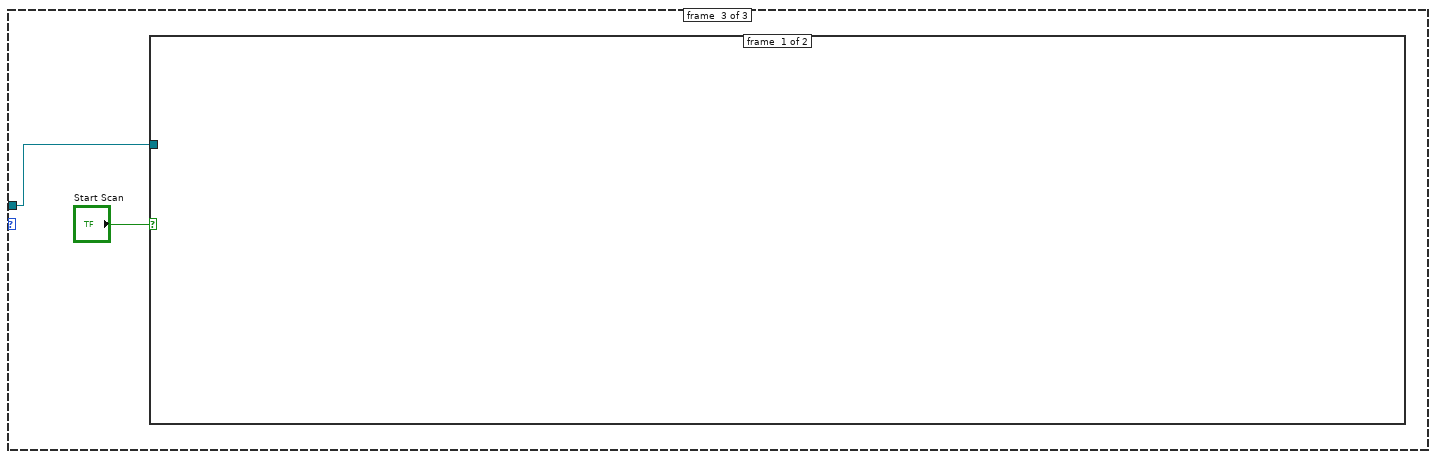
[diagram p3: hidden frame]
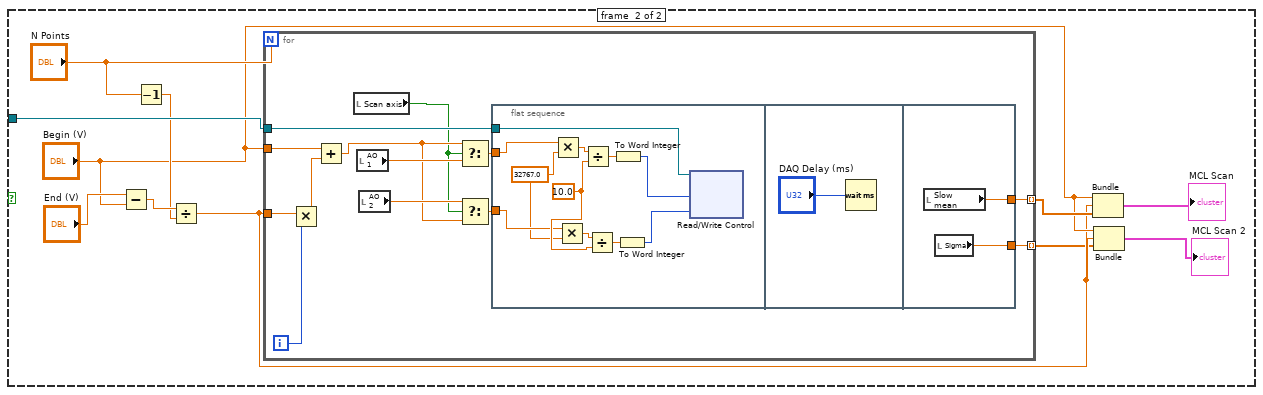
[diagram p4: hidden frame]
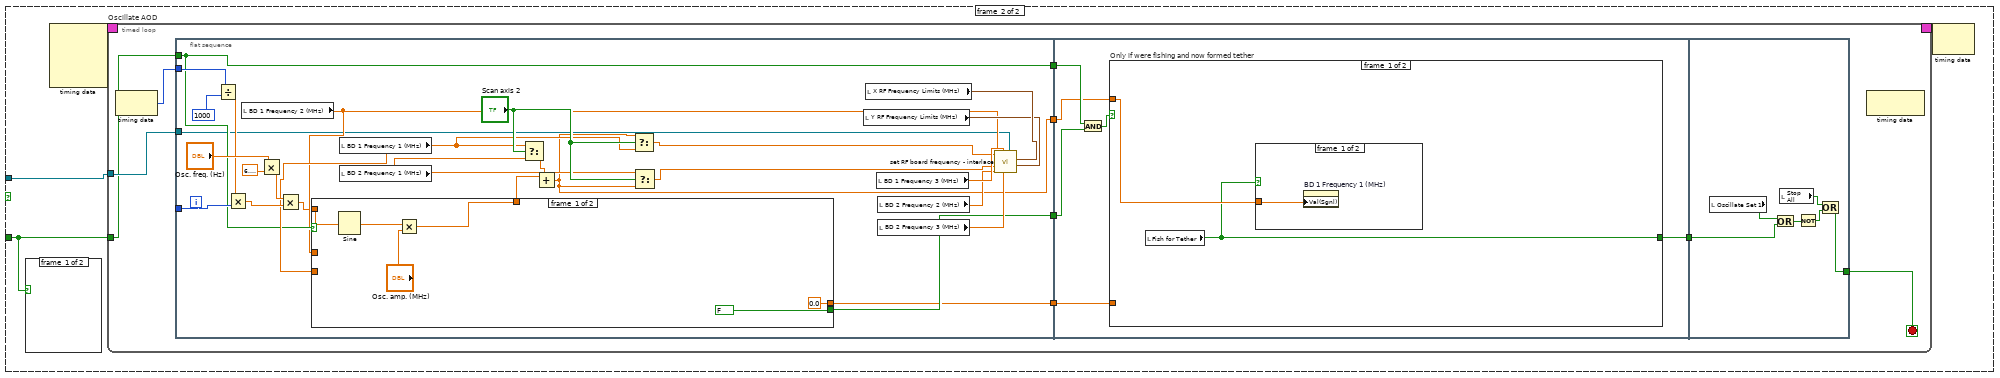
[diagram p5: hidden frame]
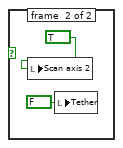
[diagram p6: hidden frame]
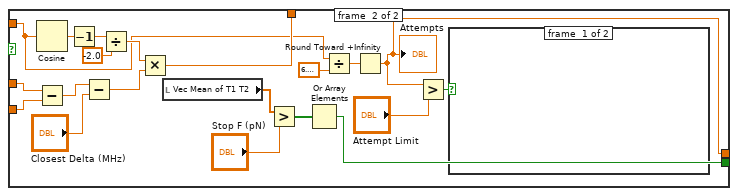
[diagram p7: hidden frame]
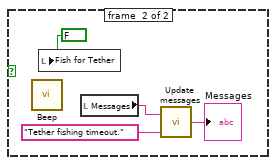
[diagram p8: hidden frame]
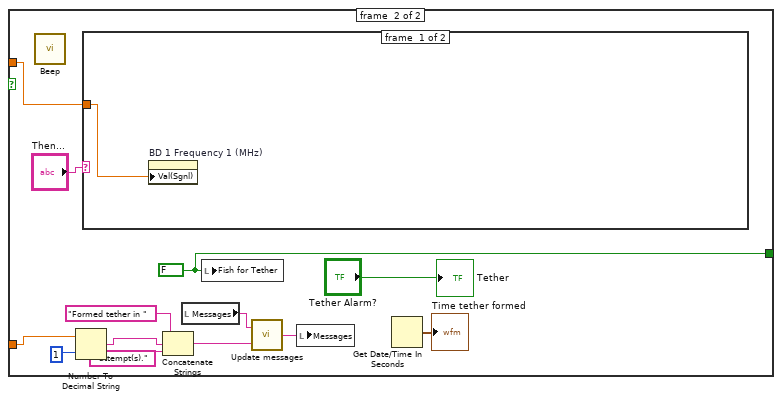
[diagram p10: hidden frame]
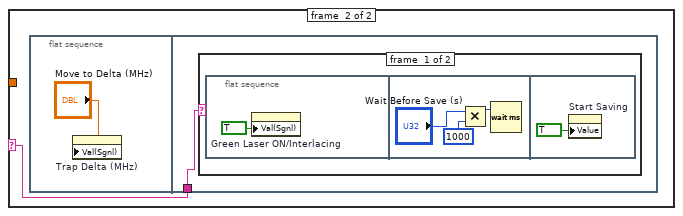
[diagram p11: hidden frame]
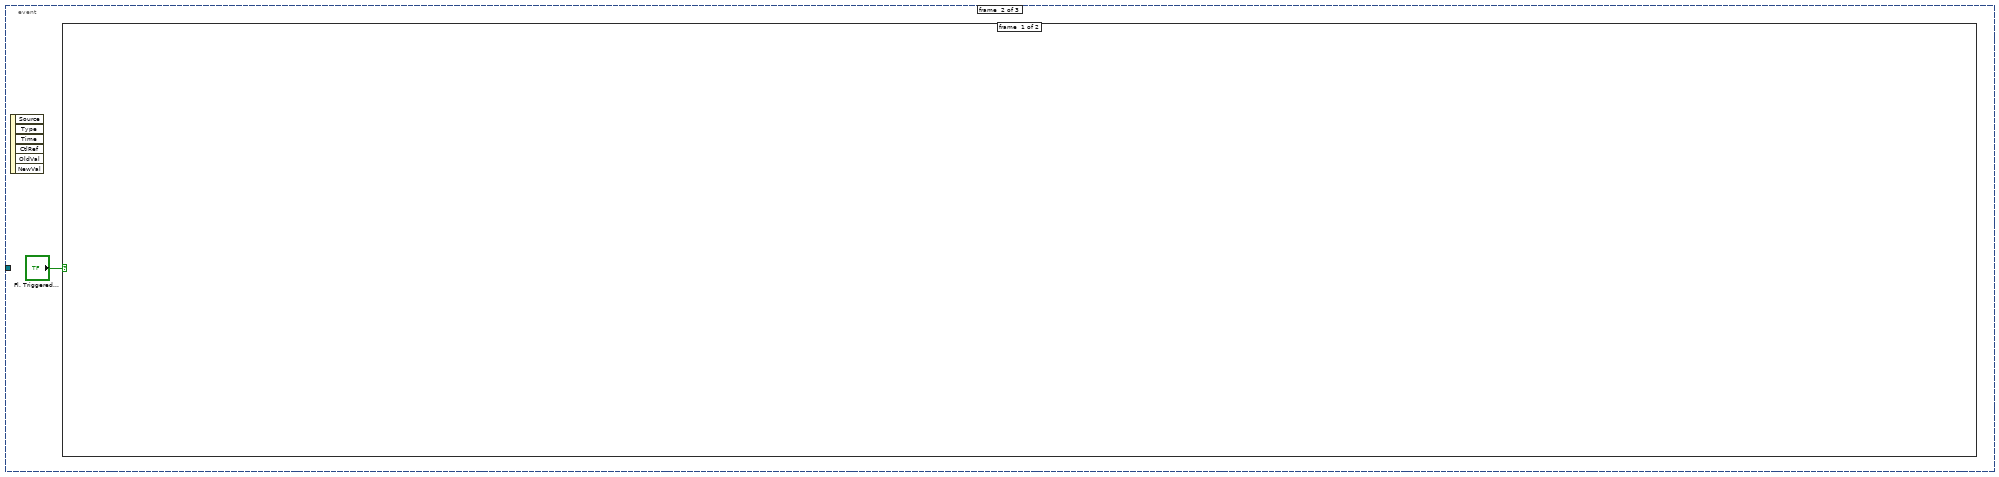
[diagram p13: hidden frame]
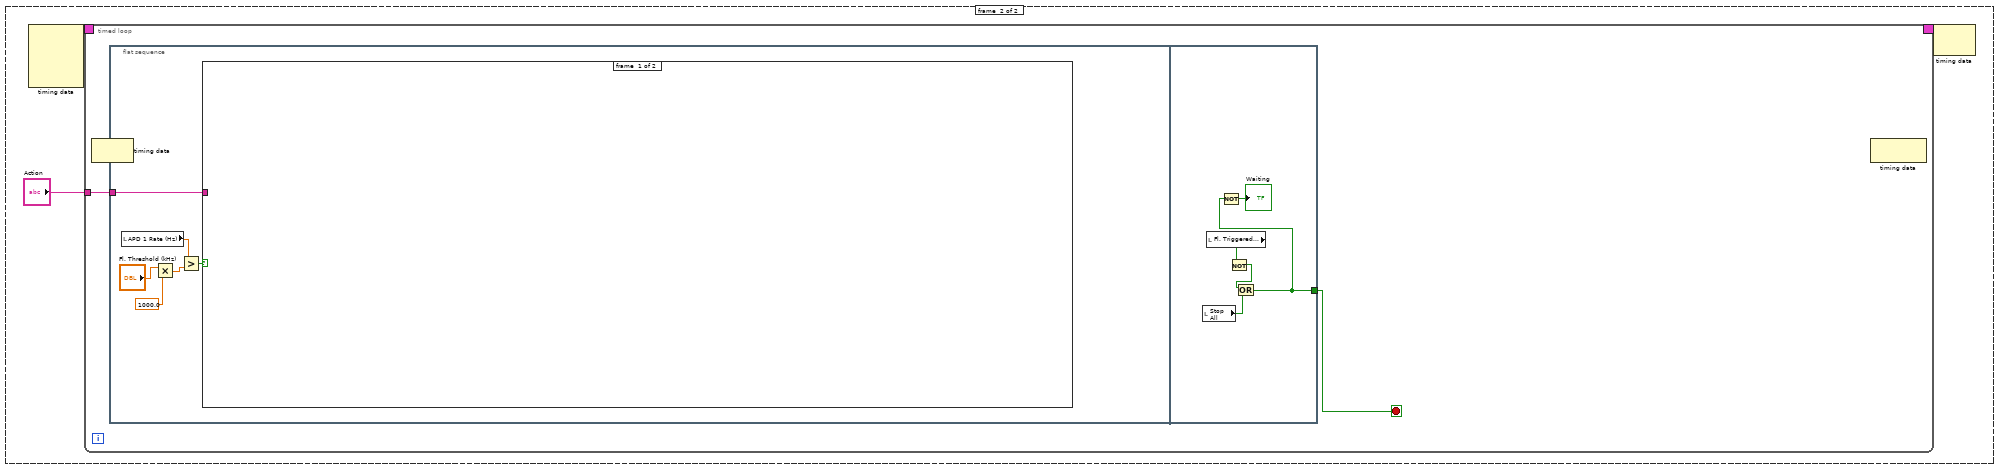
[diagram p14: hidden frame]
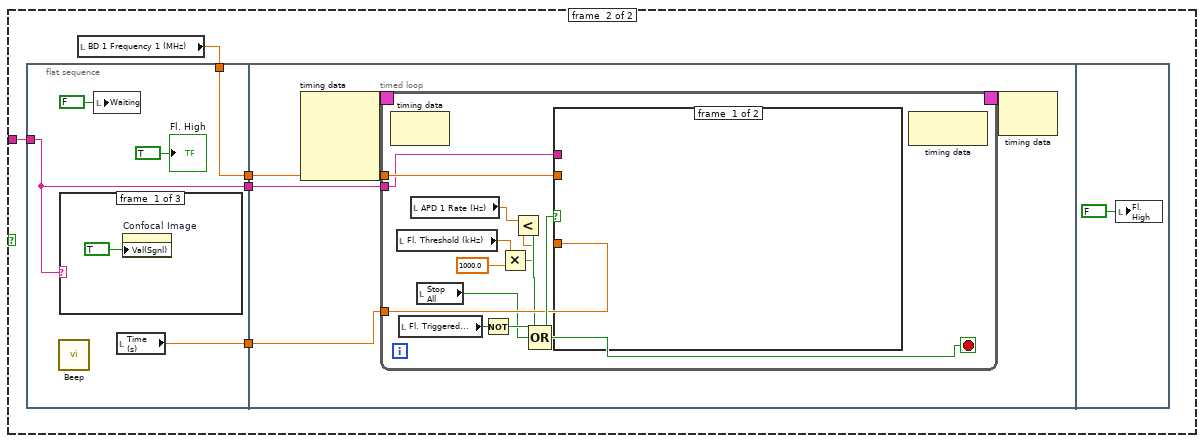
[diagram p15: hidden frame]
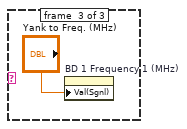
[diagram p17: hidden frame]
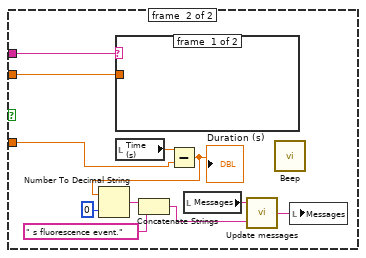
[diagram p18: hidden frame]
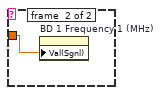
[diagram p19: hidden frame]
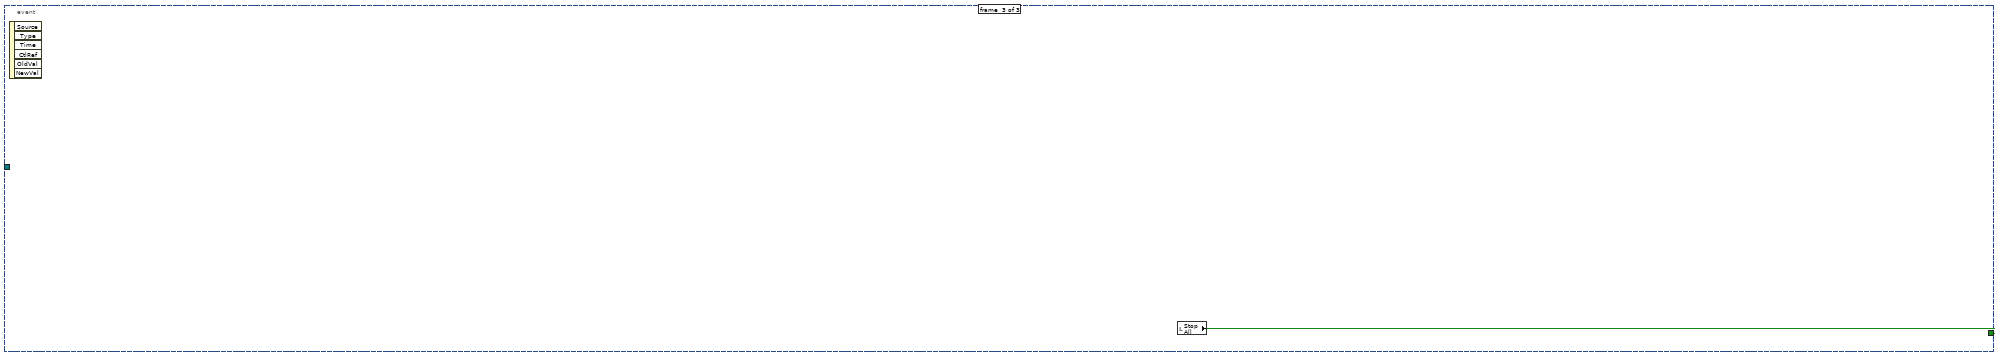
[diagram p20: hidden frame]
diagram:
  w3 = T13 2 items=["Grayscale (U8)", "Grayscale (I16)", "Grayscale (SGL)", "Complex (CSG)", "RGB (U32)", "HSL (U32)", "RGB (U64)", "Grayscale (U16)"] ("Image Type")
  w59 = T12 {"Minimum"=-0.1, "Maximum"=0.1, "Increment"=0.1}  # Z Limits
  w72 = cluster{"output high":i16, "output low":i16} {"output high"=3000, "output low"=0} ("FB output range 1")
  w78 = TRUE ("AI to FIFO")
  w163 = 10.0 ("y")
  w162 = 32767.0 ("y")
  w178 = 6.0  # clock mult.
  w179 = 49152000.0  # TCXO frequ.
  n1 = Build Array("DIO count 1 (ticks)", "DIO count 2 (ticks)", "DIO count 3 (ticks)") -> (w54:u32[])
  n2 = Multiply(x="APD Integration Time (s)", y=40000000.0) -> (x*y=w86:dbl)
  n3 = Reciprocal(x="APD Integration Time (s)") -> (1/x=w83:dbl)
  n4 = local write "APD Acq Rate (Hz)"(w83) -> ()
  n5 = local read "AO1"() -> (w157:dbl)
  n6 = local read "AO2"() -> (w156:dbl)
  n7 = To Unsigned Long Integer(number=w86) -> (unsigned 32bit integer=w85:u32)
  "APD Int. Count" <- w85
  n8 = local read "Scan Increment (MHz)"() -> (w174:dbl)
  n9 = local read "Fast Scan Dir"() -> (w143:bool)
  n10 = local read "Continuous MCL Scanning"() -> (w144:bool)
  n11 = Multiply(x=w157, y=w162) -> (x*y=w159:dbl)
  n12 = Multiply(x=w156, y=w162) -> (x*y=w161:dbl)
  n13 = local read "Number of scans (MCL)"() -> (w145:u64)
  n14 = Divide(x=w159, y=w163) -> (x/y=w158:dbl)
  n15 = Divide(x=w161, y=w163) -> (x/y=w160:dbl)
  n16 = To Word Integer(number=w158) -> (16bit integer=w155:i16)
  n17 = To Word Integer(number=w160) -> (16bit integer=w154:i16)
  n18 = Not(x=w143) -> (.not. x?=w138:bool)
  n19 = local read "Cycles/step (MCL)"() -> (w146:u64)
  n20 = Multiply(x=w174, y=1000.0) -> (x*y=w181:dbl)
  n21 = local read "Scan steps (MCL)"() -> (w147:u64)
  n22 = local read "Desired Scan Incr (V)"() -> (w149:dbl)
  n23 = Scale By Power Of 2(n=48, x=w181) -> (x*2^n=w182:dbl)
  n24 = Multiply(x=w179, y=w178) -> (x*y=w177:dbl)
  n25 = Divide(x=w182, y=w177) -> (x/y=w176:dbl)
  n26 = local read "Setpoints (V)"() -> (w202:cluster{"Set 1":dbl, "Set 2":dbl})
  n27 = property on="AI Count (ticks)" class="DigNum (strict)"("Val(Sgnl)"="AI Count (ticks)") -> ()  [unwired: 2 in, 2 out]
  n28 = local read "Number Interlace Sets"() -> (w47:u8)
  n29 = Split 1D Array(array=w54, index=w47) -> (first subarray=w56:u32[])  [unwired: 1 out]
  n30 = Add Array Elements(numeric array=w56) -> (sum=w55:u32)
  n31 = To Quad Integer(1:w176) -> (0:w173:i64)
  n32 = local read "Sets to FIFO (Traps)"() -> (w209:T11)
  n33 = local read "# Samples/channel"() -> (w166:u32)
  n34 = local read "Number of F/B Scans (AOD)"() -> (w167:u16)
  n35 = local read "Not-Interlacing Set"() -> (w46:enum32{"Set 1", "Set 2", "Set 3"})
  n36 = To Unsigned Byte Integer(number=w46) -> (unsigned 8bit integer=w52:u8)
  n37 = Index Array(array=w54, index=w52) -> (element=w53:u32)
  n38 = Divide(x=40000000.0, y="AI Count (ticks)") -> (x/y=w134:dbl)
  n39 = Multiply(x=w149, y=32767.0) -> (x*y=w151:dbl)
  n40 = local read "Feedback On/Off"() -> (w205:cluster{"Set 1":bool, "Set 2":bool})
  n41 = local read "PID Gains"() -> (w197:T9)
  n42 = local read "Scan steps (AOD)"() -> (w172:u64)
  n43 = local read "All FB On/Off"() -> (w206:bool)
  n44 = local write "AI rate (Hz)"(w134) -> ()
  n45 = local read "Cycles/step (AOD)"() -> (w171:u64)
  n46 = Divide(x=w151, y=10.0) -> (x/y=w150:dbl)
  n47 = Multiply(x=w172, y=w171) -> (x*y=w170:u64)
  n48 = Multiply(x=3276.7, y=w202) -> (x*y=w201:cluster{"Set 1":dbl, "Set 2":dbl})
  n49 = To Word Integer(number=w150) -> (16bit integer=w148:i16)
  n50 = Multiply(x=w170, y=u64 2) -> (x*y=w168:u64)
  n51 = Divide(x=w134, y="FPGA Ave.") -> (x/y=w135:dbl)
  n52 = To Word Integer(number=w201) -> (16bit integer=w200:cluster{"Set 1":i16, "Set 2":i16})
  n53 = xnode "Open FPGA VI Reference"("resource name"=T14 "750kHzDAQ") -> ("FPGA VI Reference Out"=w189:T15, "error out"=w188:errorcluster)  [unwired: 1 in]
  n54 = Unbundle By Name(w197) -> ("Set 1"=w196:T10, "Set 2"=w195:T10)
  n55 = Multiply(x=w168, y=w167) -> (x*y=w165:u64)
  n56 = Divide(x=w165, y=w166) -> (x/y=w164:dbl)
  n57 = Unbundle By Name(w200) -> ("Set 1"=w199:i16, "Set 2"=w198:i16)
  n58 = local write "Ave. Rate (Hz)"(w135) -> ()
  n59 = And(x=w205, y=w206) -> (x .and. y?=w204:cluster{"Set 1":bool, "Set 2":bool})
  n60 = local read "2D or 1D Scan"() -> (w75:bool)
  n61 = local write "Data points/scans"(w165) -> ()
  n62 = local read "Scan BD"() -> (w183:bool)
  n63 = Reciprocal(x=w135) -> (1/x=w136:dbl)
  n64 = local write "Data points/scan (f/b)"(w168) -> ()
  n65 = local read "N Acq Sets (Traps + Fl.)"() -> (w127:i16)
  n66 = local write "N sets should be saved"(w164) -> ()
  n67 = Unbundle By Name(w204) -> ("Set 1"=w208:bool, "Set 2"=w207:bool)
  n68 = xnode "Invoke Method"("FPGA VI Reference In"=w189, "error in"=w188) -> ("FPGA VI Reference Out"=w71:T15, "error out"=w101:errorcluster)
  n69 = local read "Interlace"() -> (w48:bool)
  n70 = Select(t=w55, s=w48, f=w53) -> (s? t:f=w45:u32)
  n71 = local write "Update Count (MCL)"(w45) -> ()
  n72 = local write "Total Counts (ticks)"(w45) -> ()
  n73 = local write "Ave. Period (s)"(w136) -> ()
  n74 = property on="2D or 1D Scan" class="Bool (strict)"("Val(Sgnl)"=w75) -> ()  [unwired: 2 in, 2 out]
  n75 = xnode "Read/Write Control"("FPGA VI Reference In"=w70, "error in"=w101, "ai count"="AI Count (ticks)", "AI Averages"="FPGA Ave.", "DMA buffer timeout"=0, "AI to FIFO"=FALSE, "Interlace ON/OFF"=w48, "Number Interlace Cycles"=w47, "AI1 Sets to FIFO"=w209, "FB On/Off Set 1"=w208, "FB On/Off Set 2"=w207, "Interlace Off Parameters"=w46, "FB Setpoint Set 1"=w199, "FB Setpoint Set 2"=w198, "FB Gains Set 1"=w196, "FB Gains Set 2"=w195, "FB output range 1"=w72, "FB output range 2"=w72, "Cycles per step"=w171, "Scan BD"=w183, "Number of scans"=w167, "Scan steps"=w172, "Scan freq.  increment"=w173, "AO1"=w155, "AO2"=w154, "Scan freq.  increment (MCL)"=w148, "Scan steps (MCL)"=w147, "Cycles per step (MCL)"=w146, "Number of scans (MCL)"=w145, "MCL count"=w45, "Cont. Scan (MCL)"=w144, "MCL Scan Axis"=w138, "1D or 2D Scan?"=w75, "N of AI1 Int Acq Sets"=w127, "Freq or Amp switch first"="Freq or Amp switch first", "Freq switch delay"="Freq switch delay", "Amp switch delay"="Amp switch delay", "Swap F1 and F2"="Swap F1 and F2", "APD Acq Rate Count"=w85, "APD to FIFO"=FALSE, "APD Gate Operating Mode"="APD Gate", "APD Gate ON Count"="APD Gate ON Count", "APD Gate OFF Count"="APD Gate OFF Count", "Invert APD Gate"="Invert APD Gate", "DIO count 1 (ticks)"="DIO count 1 (ticks)", "DIO count 2 (ticks)"="DIO count 2 (ticks)", "DIO count 3 (ticks)"="DIO count 3 (ticks)", "APD 1 AO scale factor"="APD 1 AO Mult.", "APD 2 AO scale factor"="APD 2 AO Mult.", "APD 1 AO offset"="APD 1 AO offset", "APD 2 AO offset"="APD 2 AO offset") -> ("FPGA VI Reference Out"=w40:T15, "error out"=w42:errorcluster)
  n76 = local read "Green Laser ON/Interlacing"() -> (w43:bool)
  n77 = local read "GI Frequency, OFF count"() -> (w36:u32)
  n78 = Multiply(x="Current When FB OFF (%)", y=655.35) -> (x*y=w26:dbl)
  n79 = local read "GI Frequency, ON count"() -> (w35:u32)
  n80 = local read "Green laser mode"() -> (w44:enum32{"Laser ON", "Laser OFF", "Interlace"})
  n81 = local read "Green FB Count"() -> (w34:u32)
  n82 = To Unsigned Word Integer(number=w26) -> (unsigned 16bit integer=w24:u16)
  n83 = local read "Invert GI"() -> (w38:bool)
  n84 = Multiply(x="Green FB Setpoint (mV)", y=3.2767) -> (x*y=w23:dbl)
  n85 = case shown="False" w43 {
    tunnel: w44 -> [_ w236]
    tunnel: [enum32{"Laser ON", "Laser OFF", "Interlace"}."Laser OFF" ("Green laser mode") w236] -> w37
    frame #0 {
    }
    frame #1 {
    }
  }
  n86 = To Word Integer(number=w23) -> (16bit integer=w21:i16)
  n87 = xnode "Read/Write Control"("FPGA VI Reference In"=w40, "error in"=w42, "Green interlace ON count 2"=w35, "Green interlace OFF count 2"=w36, "Invert GI 2"=w38, "Operating Mode 2"=w37, "Green FB Gains"="Green FB Gains", "Green FB Setpoint"=w21, "Green FB On/Off"="Green FB On/Off", "Current Out"=w24, "Green int current ON count adj"="Green int current ON count adj", "Green FB Count"=w34, "Operating Mode"=w37, "Green interlace OFF count"=w36, "Green interlace ON count"=w35, "Invert GI"=w38) -> ("FPGA VI Reference Out"=w39:T15, "error out"=w41:errorcluster)
  n88 = flat-sequence {
    tunnel: w71 -> [w241]
    tunnel: [w241] -> w70
    tunnel: [w240] -> w69
    tunnel: [w239] -> w68
    tunnel: [w237] -> w66
    tunnel: [w238] -> w67
    frame #0 {
      w238 = T12 {"Minimum"=0.0, "Maximum"=40.0, "Increment"=1.0} ("Min Max Inc")
      w237 = T12 {"Minimum"=0.0, "Maximum"=50.0, "Increment"=1.0} ("Data Entry Limits")
      w240 = T12 {"Minimum"=60.0, "Maximum"=90.0, "Increment"=1.0} ("Min Max Inc")
      w239 = T12 {"Minimum"=0.0, "Maximum"=50.0, "Increment"=1.0} ("Data Entry Limits")
      n89 = property on="BD 2 Frequency 1 (MHz)" class="DigNum (strict)"("Data Range"=w238) -> ()  [unwired: 2 in, 2 out]
      n90 = property on="BD 2 Frequency 3 (MHz)" class="DigNum (strict)"("Data Range"=w238) -> ()  [unwired: 2 in, 2 out]
      n91 = property on="BD 2 Frequency 2 (MHz)" class="DigNum (strict)"("Data Range"=w238) -> ()  [unwired: 2 in, 2 out]
      n92 = property on="BD 1 Frequency 1 (MHz)" class="DigNum (strict)"("Data Range"=w240) -> ()  [unwired: 2 in, 2 out]
      n93 = property on="BD 1 Frequency 2 (MHz)" class="DigNum (strict)"("Data Range"=w240) -> ()  [unwired: 2 in, 2 out]
      n94 = property on="BD 1 Frequency 3 (MHz)" class="DigNum (strict)"("Data Range"=w240) -> ()  [unwired: 2 in, 2 out]
      n95 = property on="BD 2 Amplitude 1 (%)" class="DigNum (strict)"("Data Range"=w237) -> ()  [unwired: 2 in, 2 out]
      n96 = property on="BD 2 Amplitude 2 (%)" class="DigNum (strict)"("Data Range"=w237) -> ()  [unwired: 2 in, 2 out]
      n97 = property on="BD 2 Amplitude 3 (%)" class="DigNum (strict)"("Data Range"=w237) -> ()  [unwired: 2 in, 2 out]
      n98 = property on="BD 1 Amplitude 3 (%)" class="DigNum (strict)"("Data Range"=w239) -> ()  [unwired: 2 in, 2 out]
      n99 = property on="BD 1 Amplitude 2 (%)" class="DigNum (strict)"("Data Range"=w239) -> ()  [unwired: 2 in, 2 out]
      n100 = property on="BD 1 Amplitude 1 (%)" class="DigNum (strict)"("Data Range"=w239) -> ()  [unwired: 2 in, 2 out]
      "X RF Frequency Limits (MHz)" <- w240
      "X RF Amplitude Limits (%)" <- w239
      "Y RF Amplitude Limits (%)" <- w237
      "Y RF Frequency Limits (MHz)" <- w238
    }
  }
  n101 = xnode "Invoke Method"("FPGA VI Reference In"=w39, "error in"=w41, "Depth"="FIFO Depth") -> ("FPGA VI Reference Out"=w194:T15, "error out"=w193:errorcluster)
  n102 = xnode "Invoke Method"("FPGA VI Reference In"=w194, "error in"=w193) -> ("FPGA VI Reference Out"=w100:T15, "error out"=w99:errorcluster)
  n103 = xnode "Invoke Method"("FPGA VI Reference In"=w100, "error in"=w99) -> ("FPGA VI Reference Out"=w98:T15, "error out"=w97:errorcluster)  [unwired: 1 out]
  n104 = flat-sequence "Initial FPGA Loop Relative Phase Adjustment" {
    tunnel: "Initial Phase Adjustment (AI1)" -> [w251]
    tunnel: "Initial Phase Adjustment (GI)" -> [w250]
    tunnel: w98 -> [w249]
    tunnel: w97 -> [w248]
    tunnel: "Initial Phase Adj. (MCL)" -> [w247]
    tunnel: [w252] -> w109
    tunnel: [w246] -> w105
    tunnel: "Initial Phase Adjustment (APD Acq)" -> [w245]
    tunnel: "Initial Phase Adjustment (APD Gate)" -> [w244]
    tunnel: "Initial Phase Adjustment (Green FB)" -> [w243]
    tunnel: "Initial Phase Adjustment (GI) 2" -> [w242]
    tunnel: w109 -> [w404]
    tunnel: [w405] -> w106
    tunnel: w105 -> [w405]
    tunnel: [w404] -> w104
    tunnel: w106 -> [w408]
    tunnel: w104 -> [w407]
    tunnel: [w410] -> w103
    tunnel: [w409] -> w102
    tunnel: [w569] -> w107
    tunnel: [w570] -> w108
    tunnel: w103 -> [w570]
    tunnel: w102 -> [w569]
    frame #0 {
      n105 = xnode "Read/Write Control"("FPGA VI Reference In"=w249, "error in"=w248, "Phase count adjustment"=w251, "Phase count adjustment (GI)"=w250, "Phase count adjustment (MCL)"=w247, "Phase Count Adjustment (APD Acq)"=w245, "Phase count adjustment (APD Gate)"=w244, "Phase count adjustment (Green FB)"=w243, "Phase count adjustment (GI) 2"=w242) -> ("FPGA VI Reference Out"=w246:T15, "error out"=w252:errorcluster)
    }
    frame #1 {
      n106 = Wait (ms)(milliseconds to wait=u32 1000) -> ()  [unwired: 1 out]
    }
    frame #2 {
      w406 = TRUE
      n107 = xnode "Read/Write Control"("FPGA VI Reference In"=w408, "error in"=w407, "+ phase"=w406, "+ phase (GI)"=w406, "+ phase (MCL)"=w406, "+ phase (APD Acq)"=w406, "+ phase (APD Gate)"=w406, "+ phase (Green FB)"=w406, "+ phase (GI) 2"=w406) -> ("FPGA VI Reference Out"=w409:T15, "error out"=w410:errorcluster)
    }
    frame #3 {
      n108 = Wait (ms)(milliseconds to wait=u32 1000) -> ()  [unwired: 1 out]
    }
  }
  n109 = local read "Phase adj. (Green FB)"() -> (w57:i16)
  n110 = local read "Phase adj. (GI) 2"() -> (w27:i16)
  n111 = local read "Phase adj. (AI1)"() -> (w141:i16)
  n112 = local read "Phase adj. (GI)"() -> (w140:i16)
  n113 = local read "Phase adjust (MCL)"() -> (w139:i16)
  n114 = xnode "Read/Write Control"("FPGA VI Reference In"=w107, "error in"=w108, "Phase count adjustment"=w141, "Phase count adjustment (GI)"=w140, "Phase count adjustment (MCL)"=w139, "Phase Count Adjustment (APD Acq)"="Phase Adj. (APD Acq)", "Phase count adjustment (APD Gate)"="Phase Adj. (APD Gate)", "Phase count adjustment (Green FB)"=w57, "Phase count adjustment (GI) 2"=w27) -> ("FPGA VI Reference Out"=w8:T15, "error out"=w116:errorcluster)
  n115 = call "Initialize RF boards - interlace 3.vi"("error in"=w116, "FPGA VI Reference In"=w8) -> ("error out"=w114:errorcluster, "FPGA VI Reference Out"=w115:T15)
  n116 = call "set RF board frequency - interlace.vi"("Board 2 Frequency Limits"=w67, "Board 1 Frequency Limits"=w69, "error in"=w114, "FPGA VI Reference In"=w115, "Board 2 Frequency 3 (MHz)"="BD 2 Frequency 3 (MHz)", "Board 1 Frequency 3 (MHz)"="BD 1 Frequency 3 (MHz)", "Board 2 Frequency 2 (MHz)"="BD 2 Frequency 2 (MHz)", "Board 2 Frequency 1 (MHz)"="BD 2 Frequency 1 (MHz)", "Board 1 Frequency 2 (MHz)"="BD 1 Frequency 2 (MHz)", "Board 1 Frequency 1  (MHz)"="BD 1 Frequency 1 (MHz)") -> ("error out"=w225:errorcluster, "FPGA VI Reference Out"=w226:T15)
  n117 = call "set RF board amplitude - interlace.vi"("Board 2 Amplitude Limits"=w66, "Board 1 Amplitude Limits"=w68, "error in"=w225, "FPGA VI Reference In"=w226, "Board 2 Amplitude 3 (%)"="BD 2 Amplitude 3 (%)", "Board 1 Amplitude 3 (%)"="BD 1 Amplitude 3 (%)", "Board 2 Amplitude 2 (%)"="BD 2 Amplitude 2 (%)", "Board 2 Amplitude 1 (%)"="BD 2 Amplitude 1 (%)", "Board 1 Amplitude 2 (%)"="BD 1 Amplitude 2 (%)", "Board 1 Amplitude 1 (%)"="BD 1 Amplitude 1 (%)") -> ("error out"=w213:errorcluster, "FPGA VI Reference Out"=w214:T15)
  n118 = flat-sequence {
    tunnel: w214 -> [w579]
    tunnel: w213 -> [w578]
    tunnel: [w577] -> w218
    tunnel: [w576] -> w217
    tunnel: [w620] -> w216
    tunnel: w218 -> [w620]
    tunnel: [w619] -> w215
    tunnel: w217 -> [w619]
    tunnel: w216 -> [w628]
    tunnel: w215 -> [w627]
    tunnel: [w626] -> w80
    tunnel: [w625] -> w79
    frame #0 {
      n119 = local read "Trap 1 (ON/OFF)"() -> (w571:bool)
      n120 = xnode "Read/Write Control"("FPGA VI Reference In"=w579, "error in"=w578, "Direct RF Box  Communication"=FALSE) -> ("FPGA VI Reference Out"=w577:T15, "error out"=w576:errorcluster)
      n121 = local write "Saving..."(FALSE ("Saving Data")) -> ()
      n122 = local write "Stop All"(FALSE ("Stop All")) -> ()
      n123 = local write "Index"(1.0 ("Index")) -> ()
      n124 = property on="Trap 1 ON" class="Bool (strict)"("Value"=w571) -> ()  [unwired: 2 in, 2 out]
      "Manipulating Trap" <- FALSE ("Manipulating Trap")
    }
    frame #1 {
      n125 = local read "Trap 2 (ON/OFF)"() -> (w618:bool)
      n126 = Wait (ms)(milliseconds to wait=u32 10) -> ()  [unwired: 1 out]
      n127 = property on="Trap 2 ON" class="Bool (strict)"("Val(Sgnl)"=w618) -> ()  [unwired: 2 in, 2 out]
    }
    frame #2 {
      n128 = xnode "Read/Write Control"("FPGA VI Reference In"=w628, "error in"=w627, "FPGA Controls  RF Box"=TRUE ("Direct RF Box  Communication")) -> ("FPGA VI Reference Out"=w626:T15, "error out"=w625:errorcluster)
      n129 = call "Update messages.vi"("Message to add"="UHR-Fleezers ready.", "Old message string"="") -> ("New message string"=w624:string)
      n130 = local write "Messages"(w624) -> ()
    }
  }
  n131 = Subtract(x="BD 1 Frequency 1 (MHz)", y="BD 1 Frequency 2 (MHz)") -> (x-y=w126:dbl)
  n132 = Subtract(x="BD 2 Frequency 1 (MHz)", y="BD 2 Frequency 2 (MHz)") -> (x-y=w125:dbl)
  n133 = Square(x=w125) -> (x^2=w123:dbl)
  n134 = Square(x=w126) -> (x^2=w124:dbl)
  n135 = Add(x=w124, y=w123) -> (x+y=w122:dbl)
  n136 = Square Root(x=w122) -> (sqrt(x)=w121:dbl)
  n137 = local write "Trap Delta (MHz)"(w121) -> ()
  n138 = xnode "Read/Write Control"("FPGA VI Reference In"=w80, "error in"=w79, "AI to FIFO"=w78, "APD to FIFO"=w78) -> ("FPGA VI Reference Out"=w77:T15, "error out"=w76:errorcluster)
  n139 = property on="pos 1 z" class="DigNum (strict)"("Data Range"=w59) -> ()  [unwired: 2 in, 2 out]
  n140 = property on="pos 2 z" class="DigNum (strict)"("Data Range"=w59) -> ()  [unwired: 2 in, 2 out]
  n141 = property on="pos 3 z" class="DigNum (strict)"("Data Range"=w59) -> ()  [unwired: 2 in, 2 out]
  n142 = property on="pos 4 z" class="DigNum (strict)"("Data Range"=w59) -> ()  [unwired: 2 in, 2 out]
  n143 = node-c288() -> (w13:T18)  [unwired: 4 out]
  n144 = node-c288() -> (w15:T18)  [unwired: 4 out]
  n145 = node-c288(i64 1 ("Period")) -> (w130:T18)  [unwired: 3 out]
  n146 = node-c288() -> (w11:T18)  [unwired: 4 out]
  n147 = node-c288() -> (w19:T18)  [unwired: 4 out]
  n148 = node-c288() -> (w17:T18)  [unwired: 4 out]
  n149 = call "IMAQ Create"("Image Name"="Det. Y Image", "Image Type"=w3) -> ("New Image"=w1:T2)  [unwired: 3 in, 1 out]
  n150 = call-poly "VISA Configure Serial Port"("VISA resource name"="Sample Chamber Stage Serial Port") -> ("VISA resource name out"=w63:refnum<visa-resource-name>, "error out"=w62:errorcluster)  [unwired: 5 in, 8 out]
  n151 = call "IMAQ Create"("Image Name"="Det. X Image", "Image Type"=w3) -> ("New Image"=w2:T2)  [unwired: 3 in, 1 out]
  n152 = call "IMAQ Create"("Image Name"="APD1 Image", "Image Type"=w3) -> ("New Image"=w6:T2)  [unwired: 3 in, 1 out]
  n153 = flat-sequence "Video" {
    tunnel: [w675] -> w192
    tunnel: w192 -> [w711]
    tunnel: w190 -> [w709]
    frame #0 {
      n154 = while {
        stop <- w668 continue-if-true
        n155 = call "Close Video Capture.vi"() -> ("error code OUT"=w670:i32)
        n156 = Equal?(x=w670, y=0) -> (x = y?=w668:bool)
      }
      n157 = local write "Stop All"(FALSE ("Stop All")) -> ()
    }
    frame #1 {
      n158 = call "DMR_Init.vi"() -> ()  [unwired: 3 out]
    }
    frame #2 {
      # "Setting the destination format to Mono8 makes sure that the image can be displayed in the intensity plot."
      n159 = call "DMR_GetDevice.vi"("search string IN"="DE019116701") -> ("device handle OUT"=w693:i32)  [unwired: 4 in, 2 out]
      n160 = call "DMR_OpenDevice.vi"("device handle IN"=w693) -> ("driver handle OUT"=w676:i32)  [unwired: 4 out]
      n161 = call "DMR_FindList.vi"("flags IN"=u32 0 ("flags"), "list name IN"="" ("String"), "list type IN"=T21."camera descriptions", "driver handle IN"=w676) -> ("list handle OUT"=w679:i32)  [unwired: 2 out]
      n162 = call "DMR_FindList.vi"("flags IN"=u32 0 ("flags"), "list name IN"="Base", "list type IN"=T21."setting", "driver handle IN"=w676) -> ("list handle OUT"=w677:i32)  [unwired: 2 out]
      n163 = call "OBJ_GetHandle.vi"("object name IN"="VideoStandard", "list handle IN"=w679) -> ("object handle OUT"=w673:i32)  [unwired: 3 out]
      n164 = call "OBJ_GetHandle.vi"("object name IN"="PixelFormat", "list handle IN"=w677) -> ("object handle OUT"=w687:i32)  [unwired: 3 out]
      n165 = call "OBJ_SetS.vi"("value index IN"=0, "value IN"="NTSC M", "object handle IN"=w673) -> ()  [unwired: 2 out]
      n166 = call "OBJ_SetS.vi"("value index IN"=0, "value IN"="Mono8" ("value"), "object handle IN"=w687) -> ()  [unwired: 2 out]
      n167 = call "OBJ_GetHandle.vi"("object name IN"="VideoChannel", "list handle IN"=w677) -> ("object handle OUT"=w683:i32)  [unwired: 3 out]
      n168 = while {
        tunnel: [w698] -> w675
        tunnel: w676 -> [w695]
        stop <- w696 continue-if-true
        n169 = call "DMR_ImageRequestSingle.vi"("request control IN"=0, "driver handle IN"=w695) -> ("error code OUT"=w697:i32, "driver handle OUT"=w698:i32)  [unwired: 2 out]
        n170 = Equal To 0?(x=w697) -> (x = 0?=w696:bool)
      }
      n171 = call "OBJ_SetI.vi"("value index IN"=0, "value IN"=3 ("Video channel"), "object handle IN"=w683) -> ()  [unwired: 2 out]
    }
    frame #3 {
      w706 = T13 0 items=["Grayscale (U8)", "Grayscale (I16)", "Grayscale (SGL)", "Complex (CSG)", "RGB (U32)", "HSL (U32)", "RGB (U64)"] ("Image Type")
      n172 = call "IMAQ Create"("Image Name"="untitled", "Image Type"=w706) -> ("New Image"=w707:T2)  [unwired: 2 in, 2 out]
      n173 = node-c288() -> (w705:T18)  [unwired: 4 out]
      n174 = Initialize Array(u32 0 ("Window Number (0...15)"), 480 ("dimension size"), 640 ("dimension size")) -> (w700:u32[][])
      n175 = timed-loop {
        tunnel: w711 -> [w729]
        tunnel: [w728] -> w710
        tunnel: w709 -> [w727]
        tunnel: w707 -> [w726]
        timing: w705 -> [_]
        timing-out: [_] -> w704
        tunnel: w700 -> [w712]
        stop <- w715 stop-if-true
        # "This block performs the \nactual image capture."
        n176 = node-c288() -> ()  [unwired: 2 out]
        n177 = local read "Stop All"() -> (w716:bool)
        n178 = Reciprocal(x="Video Capture Rate (Hz)") -> (1/x=w718:dbl)
        n179 = Or(x=FALSE, y=w716) -> (x .or. y?=w715:bool)
        n180 = Multiply(x=w718, y=1000.0) -> (x*y=w713:dbl)
        n181 = call "DMR_ImageRequestWaitFor.vi"("queue number IN"=0, "timeout(ms) IN"=500, "driver handle IN"=w729) -> ("error code OUT"=w733:i32, "request number OUT"=w730:i32, "driver handle OUT"=w731:i32)
        n182 = feedback #1(T22 refnum ("Avi Refnum")) -> (w720:T22)
        n183 = case shown="True" "New Video File" {
          tunnel: [T22 refnum ("Avi Refnum") w750] -> w722
          tunnel: [FALSE TRUE] -> w723
          tunnel: w720 -> [_ w746]
          frame #0 {
          }
          frame #1 {
            n184 = call "Create new save file.vi"("Ext"=".avi" ("string"), "Index In"="Video Index") -> ("Path Out"=w742:path, "Index Out"=w743:dbl)  [unwired: 1 in]
            "Path Out" <- w742
            n185 = Not Equal?(x=w746, y=T22 refnum ("Avi Refnum")) -> (x != y?=w747:bool)
            n186 = Increment(x=w743) -> (x+1=w752:dbl)
            n187 = case shown="True" w747 {
              tunnel: w746 -> [_ w753]
              frame #0 {
              }
              frame #1 {
                n188 = call "IMAQ AVI Close"("Avi Refnum"=w753) -> ()  [unwired: 1 in, 10 out]
              }
            }
            n189 = call "IMAQ AVI Create"("Frames Per Second"=u32 30, "AVI Path"=w742) -> ("Avi Refnum"=w750:T22)  [unwired: 5 in, 4 out]
            n190 = local write "Video Index"(w752) -> ()
          }
        }
        n191 = Equal To 0?(x=w733) -> (x = 0?=w732:bool)
        n192 = Select(t=w722, s=w723, f=w720) -> (s? t:f=w721:T22)
        n193 = case shown="True" w732 {
          tunnel: w731 -> [w754 w794]
          tunnel: w730 -> [_ w793]
          tunnel: [w754 w790] -> w728
          tunnel: w727 -> [_ w780]
          tunnel: w726 -> [_ w773]
          tunnel: w712 -> [_ w777]
          tunnel: w721 -> [_ w775]
          frame #0 {
          }
          frame #1 {
            w784 = u32 0 ("X-offset IN")
            n194 = call "DMR_GetImageRequestBufferData.vi"("driver handle IN"=w794, "request number IN"=w793) -> ("width OUT"=w783:i32, "height OUT"=w782:i32, "driver handle OUT"=w789:i32, "request number OUT"=w788:i32, "bytes per pixel OUT"=w785:i32)  [unwired: 13 out]
            n195 = call "DMR_GetImageRequestBufferImageData.vi"("driver handle IN"=w789, "request number IN"=w788, "bytes per pixel IN"=w785, "X-offset IN"=w784, "Y-offset IN"=w784, "height IN"=w782, "width IN"=w783) -> ("driver handle OUT"=w787:u32, "request number OUT"=w786:u32, "image OUT"=w778:u32[][])  [unwired: 10 out]
            n196 = call "DMR_ImageRequestUnlock.vi"("request number IN"=w786, "driver handle IN"=w787) -> ("driver handle OUT"=w792:i32)  [unwired: 1 in, 2 out]
            n197 = case shown="True" "Averaging" {
              tunnel: w778 -> [w820 w825]
              tunnel: [w820 w824] -> w774
              tunnel: w777 -> [_ w822]
              frame #0 {
              }
              frame #1 {
                (unwired) 1
                w830 = 1
                n198 = feedback #2(w822) -> (w821:u32[][])
                n199 = Add(x=w825, y=w821) -> (x+y=w826:u32[][])
                n200 = Select(t=w822, s="Reset Averaging", f=w826) -> (s? t:f=w828:u32[][])
                n201 = feedback #3(w830) -> (w823:i32)
                n202 = Divide(x=w826, y=w823) -> (x/y=w827:dbl[][])
                n203 = Increment(x=w823) -> (x+1=w831:i32)
                n204 = To Unsigned Long Integer(number=w827) -> (unsigned 32bit integer=w824:u32[][])
                n205 = Select(t=w830, s="Reset Averaging", f=w831) -> (s? t:f=w829:i32)
              }
            }
            "Image" <- w774
            n206 = case shown="True" "Capture and Save Image" {
              tunnel: w774 -> [_ w842]
              tunnel: w780 -> [_ w841]
              frame #0 {
              }
              frame #1 {
                n207 = To Unsigned Byte Integer(number=w842) -> (unsigned 8bit integer=w838:u8[][])
                n208 = call <vilib>:"Flatten Pixmap.vi"("colors"=w841, "8-bit pixmap"=w838) -> ("image data"=w839:T23)  [unwired: 4 in, 5 out]
                n209 = call "Create new save file.vi"("Insert"="video_frame_" ("string"), "Ext"=".bmp" ("string"), "Index In"="Image Index") -> ("Path Out"=w834:path, "Index Out"=w840:dbl)
                n210 = call <vilib>:"Write BMP File.vi"("image data"=w839, "path to BMP file"=w834) -> ()  [unwired: 1 in, 9 out]
                n211 = Increment(x=w840) -> (x+1=w833:dbl)
                n212 = local write "Image Index"(w833) -> ()
              }
            }
            n213 = case shown="True" "Capture Video" {
              tunnel: w775 -> [_ w819]
              tunnel: w774 -> [_ w817]
              tunnel: w773 -> [_ w816]
              frame #0 {
              }
              frame #1 {
                n214 = To Unsigned Byte Integer(number=w817) -> (unsigned 8bit integer=w818:u8[][])
                n215 = call "IMAQ ArrayToImage"("Image Pixels (U8)"=w818, "Image"=w816) -> ("Image Out"=w815:T2)  [unwired: 4 in, 5 out]
                n216 = call "IMAQ AVI Write Frame"("Image"=w815, "Avi Refnum"=w819) -> ()  [unwired: 2 in, 8 out]
              }
            }
            n217 = call "DMR_ImageRequestSingle.vi"("request control IN"=0, "driver handle IN"=w792) -> ("driver handle OUT"=w790:i32)  [unwired: 3 out]
            n218 = To Double Precision Float(number=w774) -> (double precision float=w767:dbl[][])
            n219 = Initialize Array(u8 1, 480 ("dimension size"), 640 ("dimension size")) -> (w766:u8[][])
            n220 = Multiply(x=w766, y="Intensity Upper") -> (x*y=w765:u8[][])
            n221 = Multiply(x=w766, y="Intensity Lower") -> (x*y=w764:u8[][])
            n222 = In Range and Coerce(upper limit=w765, x=w767, lower limit=w764) -> (coerced(x)=w763:dbl[][])  [unwired: 1 out]
            n223 = Subtract(x=w763, y="Intensity Lower") -> (x-y=w759:dbl[][])
            n224 = Subtract(x="Intensity Upper", y="Intensity Lower") -> (x-y=w758:u8)
            n225 = Divide(x=w759, y=w758) -> (x/y=w760:dbl[][])
            n226 = Multiply(x=u8 255, y=w760) -> (x*y=w756:dbl[][])
            n227 = To Unsigned Byte Integer(number=w756) -> (unsigned 8bit integer=w755:u8[][])
            n228 = call "IMAQ ArrayToImage"("Image Pixels (U8)"=w755, "Image"=w773) -> ("Image Out"=w771:T2)  [unwired: 4 in, 5 out]
            n229 = First Call?() -> (First Call?: T/F=w772:bool)
            n230 = case shown="True" w772 {
              tunnel: w771 -> [w795 w806]
              frame #0 {
                n231 = flat-sequence {
                  tunnel: w795 -> [w801]
                  frame #0 {
                    w798 = FALSE ("Get/Set Status? (Set)")
                    w797 = 0 ("Window Number (0...15)")
                    n232 = call "IMAQ WindSize"("Get/Set Status? (Set)"=w798, "Window Number"=w797) -> ("Width & Height out"=→"Window Size":cluster{"Width":i32, "Height":i32})  [unwired: 4 in, 2 out]
                    n233 = call "IMAQ WindMove"("Window Number (0...15)"=w797, "Get/Set Status? (Set)"=w798) -> ("Coordinates (screen)"=→"Window Position":cluster{"X Position":i32, "Y Position":i32})  [unwired: 3 in, 1 out]
                    n234 = call "IMAQ WindDraw"("Resize to Image Size? (Y)"=FALSE, "Window Number (0...15)"=w797, "Image"=w801) -> ()  [unwired: 7 in, 2 out]
                  }
                  frame #1 {
                    n235 = call "IMAQ WindZoom 2"("Center Point"="Center Point", "Zoom to Fit? (False)"=FALSE, "Zoom Factor"="Zoom Factor") -> ()  [unwired: 5 in, 4 out]
                  }
                }
              }
              frame #1 {
                n236 = flat-sequence {
                  tunnel: w806 -> [w809]
                  tunnel: [w807] -> w805
                  tunnel: w805 -> [w811]
                  frame #0 {
                    w808 = TRUE ("Resize to Image Size? (Y)")
                    w807 = 0 ("Window Number (0...15)")
                    n237 = call "IMAQ WindNonTearing"("Window Number"=w807, "NonTearing? (True)"=w808) -> ()  [unwired: 8 in, 2 out]
                    n238 = call "IMAQ WindDraw"("Resize to Image Size? (Y)"=w808, "Window Number (0...15)"=w807, "Image"=w809) -> ()  [unwired: 7 in, 2 out]
                  }
                  frame #1 {
                    n239 = disable-structure shown="Disabled" {
                      frame #0 {
                        n240 = call "IMAQ WindToolsSetup"() -> ("error out"=w814:errorcluster)  [unwired: 6 in]
                        n241 = call "IMAQ WindToolsShow"("error in (no error)"=w814) -> ()  [unwired: 4 in, 2 out]
                      }
                      frame #1 {
                      }
                    }
                    n242 = call "IMAQ WindSize"("Scrollbars? (N)"=FALSE, "Width & Height"="Initial Window Size", "Window Number"=w811) -> ()  [unwired: 3 in, 3 out]
                    n243 = call "IMAQ WindMove"("Window Number (0...15)"=w811, "Coordinates (screen)"="Initial Window Position") -> ()  [unwired: 3 in, 2 out]
                  }
                }
              }
            }
          }
        }
        n244 = node-c288(w713) -> ()  [unwired: 1 out]
      }
      n245 = node-c288(w704) -> ()  [unwired: 1 out]
      n246 = call "DMR_CloseDevice.vi"("driver handle IN"=w710) -> ()  [unwired: 1 in, 4 out]
    }
    frame #4 {
      n247 = call "DMR_Close.vi"() -> ()  [unwired: 1 out]
    }
  }
  n248 = timed-loop "Oscillate AOD (debugging)" {
    tunnel: w80 -> [w846]
    tunnel: [w845] -> w20
    timing: w13 -> [_]
    timing-out: [_] -> w12
    stop <- w845 stop-if-true
    n249 = node-c288() -> ()  [unwired: 2 out]
    n250 = event shown="[0] \"Oscillate Set 1\", \"Fish for Tether\": Value Change" {
      selector: _ -> [_ _ _]
      dyn-events: _ -> [_ _ _]
      timeout: _ -> [_ _ _]
      tunnel: w846 -> [w853 _ _]
      tunnel: [FALSE ("Stop All") _ w1036] -> w845
      event #0 {
        n251 = event-data() -> ()  [unwired: 6 out]
        n252 = local read "Oscillate Set 1"() -> (w852:bool)
        n253 = Or(x=w852, y="Fish for Tether") -> (x .or. y?=w850:bool)
        n254 = case shown="True" w850 {
          tunnel: w853 -> [_ w855]
          tunnel: "Fish for Tether" -> [_ w854]
          frame #0 {
          }
          frame #1 {
            n255 = case shown="True" w854 {
              frame #0 {
              }
              frame #1 {
                n256 = local write "Scan axis 2"(TRUE) -> ()
                n257 = local write "Tether"(FALSE ("Tether")) -> ()
              }
            }
            n258 = node-c288() -> (w857:T18)  [unwired: 4 out]
            n259 = timed-loop "Oscillate AOD" {
              timing: w857 -> [_]
              timing-out: [_] -> w856
              tunnel: w855 -> [w867]
              tunnel: w854 -> [w866]
              i -> [w869]
              stop <- w865 stop-if-true
              n260 = node-c288() -> (w868:i64)  [unwired: 1 out]
              n261 = flat-sequence {
                tunnel: w869 -> [w896]
                tunnel: w868 -> [w895]
                tunnel: w867 -> [w874]
                tunnel: w866 -> [w877]
                tunnel: [w877] -> w864
                tunnel: [w876] -> w863
                tunnel: [w873] -> w862
                tunnel: [w870] -> w860
                tunnel: w864 -> [w932]
                tunnel: w863 -> [w930]
                tunnel: w862 -> [w929]
                tunnel: [w928] -> w861
                tunnel: w860 -> [w927]
                tunnel: [w959] -> w865
                tunnel: w861 -> [w958]
                frame #0 {
                  n262 = Divide(x=w895, y=i64 1000) -> (x/y=w890:dbl)
                  n263 = Multiply(x=w890, y=w896) -> (x*y=w892:dbl)
                  n264 = local read "BD 1 Frequency 2 (MHz)"() -> (w875:dbl)
                  n265 = Multiply(x="Osc. freq. (Hz)", y=6.283185307179586) -> (x*y=w893:dbl)
                  n266 = Multiply(x=w893, y=w892) -> (x*y=w872:dbl)
                  n267 = local read "BD 1 Frequency 1 (MHz)"() -> (w880:dbl)
                  n268 = case shown="True" w877 {
                    tunnel: w872 -> [w902 w907]
                    tunnel: w880 -> [_ w918]
                    tunnel: w875 -> [_ w919]
                    tunnel: [w899 w913] -> w878
                    tunnel: [FALSE w910] -> w873
                    tunnel: [0.0 w903] -> w870
                    frame #0 {
                      n269 = Sine(x=w902) -> (sin(x)=w900:dbl)
                      n270 = Multiply(x=w900, y="Osc. amp. (MHz)") -> (x*y=w899:dbl)
                    }
                    frame #1 {
                      n271 = Cosine(x=w907) -> (cos(x)=w922:dbl)
                      n272 = Subtract(x=w919, y=w918) -> (x-y=w917:dbl)
                      n273 = Decrement(x=w922) -> (x-1=w921:dbl)
                      n274 = Subtract(x=w917, y="Closest Delta (MHz)") -> (x-y=w914:dbl)
                      n275 = Divide(x=w921, y=-2.0) -> (x/y=w915:dbl)
                      n276 = Multiply(x=w915, y=w914) -> (x*y=w913:dbl)
                      n277 = local read "Vec Mean of T1 T2"() -> (w909:dbl[])
                      n278 = Greater?(x=w909, y="Stop F (pN)") -> (0:w911:bool[])
                      n279 = Or Array Elements(Boolean array=w911) -> (logical OR=w910:bool)
                      n280 = Divide(x=w907, y=6.283185307179586) -> (x/y=w906:dbl)
                      n281 = Round Toward +Infinity(x=w906) -> (ceil(x): smallest int >= x=w903:dbl)
                      "Attempts" <- w903
                      n282 = Greater?(x=w903, y="Attempt Limit") -> (0:w905:bool)
                      n283 = case shown="True" w905 {
                        frame #0 {
                        }
                        frame #1 {
                          n284 = call <vilib>:"Beep.vi"() -> ()  [unwired: 3 in, 9 out]
                          n285 = local write "Fish for Tether"(FALSE ("Fish for Tether")) -> ()
                          n286 = local read "Messages"() -> (w924:string)
                          n287 = call "Update messages.vi"("Message to add"="Tether fishing timeout." ("Messages"), "Old message string"=w924) -> ("New message string"=→"Messages":string)
                        }
                      }
                    }
                  }
                  n288 = local read "BD 2 Frequency 1 (MHz)"() -> (w879:dbl)
                  n289 = Select(t=w880, s="Scan axis 2", f=w879) -> (s? t:f=w883:dbl)
                  n290 = Add(x=w878, y=w883) -> (x+y=w876:dbl)
                  n291 = Select(t=w876, s="Scan axis 2", f=w880) -> (s? t:f=w886:dbl)
                  n292 = Select(t=w879, s="Scan axis 2", f=w876) -> (s? t:f=w885:dbl)
                  n293 = local read "Y RF Frequency Limits (MHz)"() -> (w881:T12)
                  n294 = local read "X RF Frequency Limits (MHz)"() -> (w882:T12)
                  n295 = local read "BD 1 Frequency 3 (MHz)"() -> (w889:dbl)
                  n296 = local read "BD 2 Frequency 2 (MHz)"() -> (w888:dbl)
                  n297 = local read "BD 2 Frequency 3 (MHz)"() -> (w887:dbl)
                  n298 = call "set RF board frequency - interlace.vi"("Board 2 Frequency Limits"=w881, "Board 1 Frequency Limits"=w882, "FPGA VI Reference In"=w874, "Board 2 Frequency 3 (MHz)"=w887, "Board 1 Frequency 3 (MHz)"=w889, "Board 2 Frequency 2 (MHz)"=w888, "Board 2 Frequency 1 (MHz)"=w885, "Board 1 Frequency 2 (MHz)"=w875, "Board 1 Frequency 1  (MHz)"=w886) -> ()  [unwired: 1 in, 2 out]
                }
                frame #1 {
                  n299 = And(x=w932, y=w929) -> (x .and. y?=w931:bool)
                  n300 = case "Only if were fishing and now formed tether" shown="True" w931 {
                    tunnel: w930 -> [w934 w947]
                    tunnel: [w933 w946] -> w928
                    tunnel: w927 -> [_ w942]
                    frame #0 {
                      n301 = local read "Fish for Tether"() -> (w933:bool)
                      n302 = case shown="False" w933 {
                        tunnel: w934 -> [w935 _]
                        frame #0 {
                          n303 = property on="BD 1 Frequency 1 (MHz)" class="DigNum (strict)"("Val(Sgnl)"=w935) -> ()  [unwired: 2 in, 2 out]
                        }
                        frame #1 {
                        }
                      }
                    }
                    frame #1 {
                      w946 = FALSE ("Fish for Tether")
                      n304 = call <vilib>:"Beep.vi"() -> ()  [unwired: 3 in, 9 out]
                      n305 = Number To Decimal String(number=w942, width (-)=i16 1) -> (decimal integer string=w940:string)
                      n306 = case shown="\"2\", \"3\"" "Then..." {
                        selector: "Then..." -> [_ w950]
                        tunnel: w947 -> [w949 _]
                        frame #0 {
                          n307 = property on="BD 1 Frequency 1 (MHz)" class="DigNum (strict)"("Val(Sgnl)"=w949) -> ()  [unwired: 2 in, 2 out]
                        }
                        frame #1 {
                          n308 = flat-sequence {
                            tunnel: w950 -> [w952]
                            frame #0 {
                              n309 = property on="Trap Delta (MHz)" class="DigNum (strict)"("Val(Sgnl)"="Move to Delta (MHz)") -> ()  [unwired: 2 in, 2 out]
                            }
                            frame #1 {
                              n310 = case shown="\"3\"" w952 {
                                frame #0 {
                                n311 = flat-sequence {
                                frame #0 {
                                n312 = property on="Green Laser ON/Interlacing" class="Bool (strict)"("Val(Sgnl)"=TRUE ("Value (Signaling)")) -> ()  [unwired: 2 in, 2 out]
                                }
                                frame #1 {
                                n313 = Multiply(x="Wait Before Save (s)", y=u32 1000 ("x")) -> (x*y=w955:u32)
                                n314 = Wait (ms)(milliseconds to wait=w955) -> ()  [unwired: 1 out]
                                }
                                frame #2 {
                                n315 = property on="Start Saving" class="Bool (strict)"("Value"=TRUE ("Start Saving")) -> ()  [unwired: 2 in, 2 out]
                                }
                                }
                                }
                                frame #1 {
                                }
                              }
                            }
                          }
                        }
                      }
                      n316 = Concatenate Strings("Formed tether in ", w940, " attempt(s)." ("string")) -> (w937:string)
                      n317 = local read "Messages"() -> (w944:string)
                      n318 = local write "Fish for Tether"(w946) -> ()
                      n319 = call "Update messages.vi"("Message to add"=w937, "Old message string"=w944) -> ("New message string"=w943:string)
                      n320 = local write "Messages"(w943) -> ()
                      n321 = Get Date/Time In Seconds() -> (seconds since 1Jan1904=→"Time tether formed":timestamp)
                      "Tether" <- "Tether Alarm?"
                    }
                  }
                }
                frame #2 {
                  n322 = local read "Oscillate Set 1"() -> (w963:bool)
                  n323 = Or(x=w963, y=w958) -> (x .or. y?=w960:bool)
                  n324 = local read "Stop All"() -> (w961:bool)
                  n325 = Not(x=w960) -> (.not. x?=w962:bool)
                  n326 = Compound Arithmetic op=OR(w961, w962) -> (w959:bool)
                }
              }
              n327 = node-c288() -> ()  [unwired: 2 out]
            }
            n328 = node-c288(w856) -> ()  [unwired: 1 out]
          }
        }
      }
      event #1 {
        n329 = event-data() -> ()  [unwired: 7 out]
        n330 = case shown="True" "Fl. Triggered..." {
          frame #0 {
          }
          frame #1 {
            n331 = node-c288() -> (w972:T18)  [unwired: 4 out]
            n332 = timed-loop {
              timing: w972 -> [_]
              timing-out: [_] -> w971
              tunnel: "Action" -> [w973]
              stop <- w974 stop-if-true
              n333 = node-c288() -> ()  [unwired: 2 out]
              n334 = flat-sequence {
                tunnel: w973 -> [w977]
                tunnel: [w1027] -> w974
                frame #0 {
                  n335 = local read "APD 1 Rate (Hz)"() -> (w980:dbl)
                  n336 = Multiply(x="Fl. Threshold (kHz)", y=1000.0) -> (x*y=w976:dbl)
                  n337 = Greater?(x=w980, y=w976) -> (0:w978:bool)
                  n338 = case shown="True" w978 {
                    tunnel: w977 -> [_ w983]
                    frame #0 {
                    }
                    frame #1 {
                      n339 = flat-sequence {
                        tunnel: w985 -> [w988]
                        tunnel: [w988] -> w984
                        tunnel: w983 -> [w987]
                        tunnel: [w987] -> w982
                        tunnel: [w986] -> w981
                        tunnel: w984 -> [w995]
                        tunnel: w982 -> [w994]
                        tunnel: w981 -> [w993]
                        frame #0 {
                          n340 = call <vilib>:"Beep.vi"() -> ()  [unwired: 3 in, 9 out]
                          n341 = case shown="\"Alarm\", Default" w987 {
                            frame #0 {
                              n342 = property on="Confocal Image" class="Bool (strict)"("Val(Sgnl)"=TRUE ("Value (Signaling)")) -> ()  [unwired: 2 in, 2 out]
                            }
                            frame #1 {
                            }
                            frame #2 {
                              n343 = property on="BD 1 Frequency 1 (MHz)" class="DigNum (strict)"("Val(Sgnl)"="Yank to Freq. (MHz)") -> ()  [unwired: 2 in, 2 out]
                            }
                          }
                          n344 = local write "Waiting"(FALSE ("Waiting")) -> ()
                          n345 = local read "Time (s)"() -> (w986:dbl)
                          "Fl. High" <- TRUE ("Yanking")
                        }
                        frame #1 {
                          n346 = node-c288() -> (w997:T18)  [unwired: 4 out]
                          n347 = timed-loop {
                            timing: w997 -> [_]
                            timing-out: [_] -> w996
                            tunnel: w995 -> [w1007]
                            tunnel: w994 -> [w1005]
                            tunnel: w993 -> [w1004]
                            stop <- w1006 stop-if-true
                            n348 = node-c288() -> ()  [unwired: 2 out]
                            n349 = local read "Fl. Threshold (kHz)"() -> (w999:dbl)
                            n350 = local read "Fl. Triggered..."() -> (w1008:bool)
                            n351 = local read "APD 1 Rate (Hz)"() -> (w1009:dbl)
                            n352 = local read "Stop All"() -> (w1002:bool)
                            n353 = Not(x=w1008) -> (.not. x?=w1003:bool)
                            n354 = Multiply(x=w999, y=1000.0) -> (x*y=w1000:dbl)
                            n355 = Less?(x=w1009, y=w1000) -> (x < y?=w1001:bool)
                            n356 = Compound Arithmetic op=OR(w1001, w1002, w1003) -> (w1006:bool)
                            n357 = case shown="True" w1006 {
                              tunnel: w1007 -> [_ w1020]
                              tunnel: w1005 -> [_ w1019]
                              tunnel: w1004 -> [_ w1017]
                              frame #0 {
                              }
                              frame #1 {
                                n358 = case shown="\"Yank\"" w1019 {
                                tunnel: w1020 -> [_ w1021]
                                frame #0 {
                                }
                                frame #1 {
                                n359 = property on="BD 1 Frequency 1 (MHz)" class="DigNum (strict)"("Val(Sgnl)"=w1021) -> ()  [unwired: 2 in, 2 out]
                                }
                                }
                                n360 = local read "Time (s)"() -> (w1018:dbl)
                                n361 = Subtract(x=w1018, y=w1017) -> (x-y=w1014:dbl)
                                "Duration (s)" <- w1014
                                n362 = Number To Decimal String(number=w1014, width (-)=i16 0) -> (decimal integer string=w1012:string)
                                n363 = Concatenate Strings(w1012, " s fluorescence event." ("string")) -> (w1010:string)
                                n364 = local read "Messages"() -> (w1016:string)
                                n365 = call "Update messages.vi"("Message to add"=w1010, "Old message string"=w1016) -> ("New message string"=w1015:string)
                                n366 = call <vilib>:"Beep.vi"() -> ()  [unwired: 3 in, 9 out]
                                n367 = local write "Messages"(w1015) -> ()
                              }
                            }
                            n368 = node-c288() -> ()  [unwired: 2 out]
                          }
                          n369 = node-c288(w996) -> ()  [unwired: 1 out]
                        }
                        frame #2 {
                          n370 = local write "Fl. High"(FALSE ("Yanking")) -> ()
                        }
                      }
                      n371 = local read "BD 1 Frequency 1 (MHz)"() -> (w985:dbl)
                    }
                  }
                }
                frame #1 {
                  n372 = local read "Stop All"() -> (w1030:bool)
                  n373 = local read "Fl. Triggered..."() -> (w1028:bool)
                  n374 = Not(x=w1028) -> (.not. x?=w1029:bool)
                  n375 = Or(x=w1029, y=w1030) -> (x .or. y?=w1027:bool)
                  n376 = Not(x=w1027) -> (.not. x?=→"Waiting":bool)
                }
              }
              n377 = node-c288() -> ()  [unwired: 2 out]
            }
            n378 = node-c288(w971) -> ()  [unwired: 1 out]
          }
        }
      }
      event #2 {
        n379 = event-data() -> ()  [unwired: 7 out]
        n380 = local read "Stop All"() -> (w1036:bool)
      }
    }
    n381 = node-c288() -> ()  [unwired: 2 out]
  }
  n382 = timed-loop "Control parameters (event loop)" {
    tunnel: w80 -> [w1040]
    shift-right: [w1039] -> _
    shift-left: errorcluster {"status"=FALSE, "code"=0, "source"=""} ("error out") -> [w1038]
    tunnel: [w1037] -> w184
    timing: w15 -> [_]
    timing-out: [_] -> w14
    stop <- w1037 stop-if-true
    n383 = node-c288() -> ()  [unwired: 2 out]
    n384 = event shown="[33] \"Scan steps (MCL)\", \"Number of scans (MCL)\", \"Scan Range (V)\n(of steps)\", \"2D or 1D Scan\", \"N APD Samp/step\", \"Fast Scan Dir\", \"Continuous MCL Scanning\", \"Scan lines (y)\": Value Change" {
      selector: _ -> [_ _ _ _ _ _ _ _ _ _ _ _ _ _ _ _ _ _ _ _ _ _ _ _ _ _ _ _ _ _ _ _ _ _ _ _ _ _ _ _ _ _ _ _ _]
      dyn-events: _ -> [_ _ _ _ _ _ _ _ _ _ _ _ _ _ _ _ _ _ _ _ _ _ _ _ _ _ _ _ _ _ _ _ _ _ _ _ _ _ _ _ _ _ _ _ _]
      timeout: _ -> [_ _ _ _ _ _ _ _ _ _ _ _ _ _ _ _ _ _ _ _ _ _ _ _ _ _ _ _ _ _ _ _ _ _ _ _ _ _ _ _ _ _ _ _ _]
      tunnel: w1040 -> [w1081 _ _ w1208 _ w1303 _ _ _ _ w1369 _ _ _ _ _ _ w1485 w1623 w1685 w1728 w1878 w1953 w2064 w2157 w2241 w2325 w2409 w2493 w2586 w2781 w2981 w3074 w3207 _ w3377 w3418 w3465 w3542 w3583 _ w3628 _ _ _]
      tunnel: [w1080 _ _ w1198 _ w1302 _ _ w1334 _ w1348 _ _ _ _ _ _ w1484 w1619 w1682 w1725 w1877 w1951 w2063 w2151 w2235 w2319 w2403 w2487 w2584 w2780 w2979 w3072 w3205 _ w3375 w3416 w3455 w3540 w3581 _ w3626 _ _ _] -> w1039
      tunnel: w1038 -> [w1079 _ _ w1207 _ w1301 _ _ w1334 _ w1368 _ _ _ _ _ _ w1483 w1618 w1681 w1724 w1876 w1952 w2062 w2156 w2240 w2324 w2408 w2492 w2585 w2779 w2980 w3073 w3206 _ w3376 w3417 w3464 w3541 w3582 _ w3627 _ _ _]
      tunnel: [_ _ _ _ _ _ _ _ w1333 _ _ _ _ _ _ _ _ _ _ _ _ _ _ _ _ _ _ _ _ _ _ _ _ _ _ _ _ _ _ _ _ _ _ _ _] -> w1037
      tunnel: [_ _ _ _ _ _ "Round T1 X" _ _ _ _ _ _ _ _ "Load parameters" _ _ _ _ _ _ _ _ _ _ _ _ _ _ _ _ _ _ _ _ _ _ _ _ _ _ _ _ _] -> _
      tunnel: [_ _ "Adjust Scale\nto Mean" _ _ _ _ _ _ _ _ "Set Position 1" "Set Position 2" "Set Position 3" "Set Position 4" _ _ _ _ _ _ _ _ _ _ _ _ _ _ _ _ _ _ _ _ _ _ _ _ _ _ _ _ _ _] -> _
      tunnel: [_ _ _ _ _ _ _ "Round T2 X" _ "Delayed Interlace Start" _ _ _ _ _ _ _ _ _ _ _ _ _ _ _ _ _ _ _ _ _ _ _ _ _ _ _ _ _ _ _ _ _ _ _] -> _
      tunnel: [_ "Rescale on Mean" _ _ _ _ _ _ _ _ _ _ _ _ _ _ _ _ _ _ _ _ _ _ _ _ _ _ _ _ _ _ _ _ _ _ _ _ _ _ _ _ _ _ _] -> _
      event #0 {
        # "So that if 'Save ave N' is updated, the AOD scanning code updates too."
        n385 = event-data() -> ()  [unwired: 6 out]
        n386 = local read "AI Count (ticks)"() -> (w1051:u32)
        n387 = local read "FPGA Ave."() -> (w1055:dbl)
        n388 = Boolean To (0,1)(Boolean="Sets to FIFO (Traps)") -> (0, 1=w1069:cluster{"Set 1":i16, "Set 2":i16, "Set 3":i16})
        n389 = xnode "Read/Write Control"("FPGA VI Reference In"=w1081, "error in"=w1079, "ai count"=w1051, "AI1 Sets to FIFO"="Sets to FIFO (Traps)", "AI Averages"=w1055, "N of AI1 Int Acq Sets"="N Acq Sets (Traps + Fl.)") -> ("error out"=w1080:errorcluster)  [unwired: 1 out]
        n390 = Cluster To Array(cluster=w1069) -> (array=w1068:i16[])
        n391 = local read "Scan steps (AOD)"() -> (w1070:u64)
        n392 = Multiply(x=w1051, y="N Acq Sets (Traps + Fl.)") -> (x*y=w1049:u32)
        n393 = Divide(x=40000000.0, y=w1051) -> (x/y=w1077:dbl)
        "AI rate (Hz)" <- w1077
        n394 = Add Array Elements(numeric array=w1068) -> (sum=w1053:i16)
        "Trap Sets" <- w1053
        n395 = Divide(x=w1077, y=w1055) -> (x/y=w1078:dbl)
        "Ave. Rate (Hz)" <- w1078
        n396 = Reciprocal(x=w1078) -> (1/x=→"Ave. Period (s)":dbl)
        n397 = property on="Scan steps (AOD)" class="DigNum (strict)"("Val(Sgnl)"=w1070) -> ()  [unwired: 2 in, 2 out]
        n398 = Divide(x=w1078, y="N Acq Sets (Traps + Fl.)") -> (x/y=w1074:dbl)
        "Data Rate (Hz)" <- w1074
        n399 = Reciprocal(x=w1074) -> (1/x=→"Data Period (s)":dbl)
        n400 = local read "Save ave N"() -> (w1073:dbl)
        n401 = Divide(x=w1074, y=w1073) -> (x/y=w1072:dbl)
        "Save Data Rate (Hz)" <- w1072
        n402 = Reciprocal(x=w1072) -> (1/x=→"Save Data Period (s)":dbl)
        n403 = Multiply(x=w1049, y="# Samples/trap") -> (x*y=w1045:dbl)
        "Counts/DMA" <- w1045
        n404 = Multiply(x=w1053, y="# Samples/trap") -> (x*y=w1052:dbl)
        "# Samples/channel" <- w1052
        n405 = Greater?(x=w1055, y=1.0) -> (0:w1058:bool)
        "FPGA Averaging" <- w1058
        n406 = local read "APD Int. Count"() -> (w1047:u32)
        n407 = Divide(x=w1052, y=u32 2) -> (x/y=w1061:dbl)
        n408 = Select(t=w1052, s=w1058, f=w1061) -> (s? t:f=w1066:dbl)
        n409 = Divide(x=w1045, y=w1047) -> (x/y=w1046:dbl)
        "APD Samples/FIFO Acq." <- w1046
        n410 = Divide(x=w1045, y=40000000.0) -> (x/y=w1043:dbl)
        "DMA Update Period (s)" <- w1043
        n411 = Multiply(x=w1066, y=u32 8) -> (x*y=→"Elements/DMA read":dbl)
        n412 = Multiply(x=2.0, y=w1046) -> (x*y=→"APD Elements/DMA read":dbl)
        n413 = local read "N sets to save"() -> (w1063:u32)
        n414 = Multiply(x=w1043, y=w1063) -> (x*y=→"Total Time (s)":dbl)
      }
      event #1 {
        n415 = event-data() -> ()  [unwired: 7 out]
        n416 = local read "Bead Mean (nm)"() -> (w1186:dbl)
        n417 = Add(x="Amplitude (nm)", y=w1186) -> (x+y=w1184:dbl)
        n418 = Subtract(x=w1186, y="Amplitude (nm)") -> (x-y=w1183:dbl)
        n419 = property on="Bead Separation" class="WFChart (strict)"("YScale.Maximum"=w1184) -> ()  [unwired: 2 in, 2 out]
        n420 = property on="Bead Separation" class="WFChart (strict)"("YScale.Minimum"=w1183) -> ()  [unwired: 2 in, 2 out]
      }
      event #2 {
        n421 = event-data() -> ()  [unwired: 7 out]
        n422 = local read "APD 1 Rate (Hz)"() -> (w1195:dbl)
        n423 = Multiply(x=1000.0, y="Above (kHz)") -> (x*y=w1193:dbl)
        n424 = Multiply(x=1000.0, y="Below (kHz)") -> (x*y=w1191:dbl)
        n425 = Add(x=w1193, y=w1195) -> (x+y=w1188:dbl)
        n426 = Subtract(x=w1195, y=w1191) -> (x-y=w1189:dbl)
        n427 = property on="APD 1 Chart" class="WFChart (strict)"("YScale.Maximum"=w1188) -> ()  [unwired: 2 in, 2 out]
        n428 = property on="APD 1 Chart" class="WFChart (strict)"("YScale.Minimum"=w1189) -> ()  [unwired: 2 in, 2 out]
      }
      event #3 {
        n429 = event-data() -> ()  [unwired: 7 out]
        n430 = Negate(x="Phase adj. (AI1)") -> (-x=w1205:i16)
        n431 = Select(t=w1205, s="- phase (AI1)", f="Phase adj. (AI1)") -> (s? t:f=w1204:i16)
        n432 = xnode "Read/Write Control"("FPGA VI Reference In"=w1208, "error in"=w1207, "Phase count adjustment"=w1204) -> ("FPGA VI Reference Out"=w1203:T15, "error out"=w1202:errorcluster)
        n433 = Or(x="- phase (AI1)", y="+ phase (AI1)") -> (x .or. y?=w1199:bool)
        n434 = xnode "Read/Write Control"("FPGA VI Reference In"=w1203, "error in"=w1202, "+ phase"=w1199) -> ("error out"=w1198:errorcluster)  [unwired: 1 out]
      }
      event #4 {
        w1284 = u32 9868950 ("Color Box")
        n435 = event-data() -> ("Row"=w1286:i32)  [unwired: 9 out]
        n436 = property on="All Signals" class="WFChart (strict)"("Active Plot"=w1286) -> (error out=w1297:errorcluster)  [unwired: 2 in, 1 out]
        n437 = property on="All Signals" class="WFChart (strict)" props=["Plot", "Visible?", "Plot", "Plot Color"](error in=w1297) -> (error out=w1296:errorcluster, "Plot.Visible?"=w1295:bool)  [unwired: 1 in, 2 out]
        n438 = Select(t=FALSE ("Plot.Visible"), s=w1295, f=TRUE ("Plot.Visible")) -> (s? t:f=w1290:bool)
        n439 = property on="All Signals" class="WFChart (strict)"(error in=w1296, "Plot.Visible?"=w1290) -> (error out=w1292:errorcluster)  [unwired: 1 in, 1 out]
        n440 = property on="All Signals" class="WFChart (strict)"(error in=w1292) -> (error out=w1287:errorcluster, "Plot.Plot Color"=w1291:u32)  [unwired: 1 in, 1 out]
        n441 = property on="Signals to Plot" class="LstBox (strict)"(error in=w1287, "Active Row"=w1286) -> (error out=w1285:errorcluster)  [unwired: 1 in, 1 out]
        n442 = Select(t=w1291, s=w1290, f=u32 0) -> (s? t:f=w1288:u32)
        n443 = property on="Signals to Plot" class="LstBox (strict)"(error in=w1285, "CellFontColor"=w1288, "SelColor"=w1284, "CellBG"=w1284, "CellFontSize"=u32 20 ("Active Row:Cell Font:Size"), "CellFontBold"=TRUE ("Active Row:Cell Font:Bold")) -> ()  [unwired: 1 in, 2 out]
      }
      event #5 {
        n444 = event-data() -> ("CtlRef"=w1300:refnum<vi>)  [unwired: 6 out]
        n445 = control-ref of="Trap Delta (MHz)"() -> (w1299:refnum<vi>)
        n446 = Equal?(x=w1299, y=w1300) -> (x = y?=w1298:bool)
        n447 = case shown="False" "Oscillate Set 1" {
          tunnel: w1303 -> [w1323 _]
          tunnel: [w1322 w1326] -> w1302
          tunnel: w1301 -> [w1321 w1326]
          tunnel: w1298 -> [w1306 _]
          frame #0 {
            n448 = local read "BD 1 Frequency 2 (MHz)"() -> (w1310:dbl)
            n449 = local read "BD 1 Frequency 1 (MHz)"() -> (w1308:dbl)
            n450 = Subtract(x=w1310, y="Trap Delta (MHz)") -> (x-y=w1307:dbl)
            n451 = Select(t=w1307, s=w1306, f=w1308) -> (s? t:f=w1305:dbl)
            n452 = local read "Y RF Frequency Limits (MHz)"() -> (w1311:T12)
            n453 = local read "X RF Frequency Limits (MHz)"() -> (w1312:T12)
            n454 = local read "BD 1 Frequency 3 (MHz)"() -> (w1324:dbl)
            n455 = local write "BD 1 Frequency 1 (MHz)"(w1305) -> ()
            n456 = local read "BD 2 Frequency 1 (MHz)"() -> (w1315:dbl)
            n457 = local read "BD 2 Frequency 2 (MHz)"() -> (w1314:dbl)
            n458 = local read "BD 2 Frequency 3 (MHz)"() -> (w1325:dbl)
            n459 = call "set RF board frequency - interlace.vi"("Board 2 Frequency Limits"=w1311, "Board 1 Frequency Limits"=w1312, "error in"=w1321, "FPGA VI Reference In"=w1323, "Board 2 Frequency 3 (MHz)"=w1325, "Board 1 Frequency 3 (MHz)"=w1324, "Board 2 Frequency 2 (MHz)"=w1314, "Board 2 Frequency 1 (MHz)"=w1315, "Board 1 Frequency 2 (MHz)"=w1310, "Board 1 Frequency 1  (MHz)"=w1305) -> ("error out"=w1322:errorcluster)  [unwired: 1 out]
            n460 = Subtract(x=w1315, y=w1314) -> (x-y=w1319:dbl)
            n461 = Subtract(x=w1305, y=w1310) -> (x-y=w1320:dbl)
            n462 = Square(x=w1319) -> (x^2=w1317:dbl)
            n463 = Square(x=w1320) -> (x^2=w1318:dbl)
            n464 = Add(x=w1318, y=w1317) -> (x+y=w1316:dbl)
            n465 = Square Root(x=w1316) -> (sqrt(x)=w1313:dbl)
            n466 = local write "Trap Delta (MHz)"(w1313) -> ()
            n467 = property on="Initial delta (MHz)" class="DigNum (strict)"("Val(Sgnl)"=w1313) -> ()  [unwired: 2 in, 2 out]
          }
          frame #1 {
          }
        }
      }
      event #6 {
        n468 = event-data() -> ()  [unwired: 7 out]
        n469 = local read "BD 1 Frequency 1 (MHz)"() -> (w1329:dbl)
        n470 = Round To Nearest(number=w1329) -> (nearest integer value=w1328:dbl)
        n471 = property on="BD 1 Frequency 1 (MHz)" class="DigNum (strict)"("Val(Sgnl)"=w1328) -> ()  [unwired: 2 in, 2 out]
      }
      event #7 {
        n472 = event-data() -> ()  [unwired: 7 out]
        n473 = local read "BD 1 Frequency 2 (MHz)"() -> (w1331:dbl)
        n474 = Round To Nearest(number=w1331) -> (nearest integer value=w1330:dbl)
        n475 = property on="BD 1 Frequency 2 (MHz)" class="DigNum (strict)"("Val(Sgnl)"=w1330) -> ()  [unwired: 2 in, 2 out]
      }
      event #8 {
        n476 = event-data() -> ()  [unwired: 7 out]
        n477 = local read "Stop All"() -> (w1333:bool)
      }
      event #9 {
        n478 = event-data() -> ()  [unwired: 7 out]
        n479 = flat-sequence {
          frame #0 {
            n480 = Multiply(x="Delay to Interlace (s)", y=1000.0) -> (x*y=w1336:dbl)
            n481 = Wait (ms)(milliseconds to wait=w1336) -> ()  [unwired: 1 out]
          }
          frame #1 {
            n482 = property on="Green laser mode" class="RadioBtnsControl (strict)"("Val(Sgnl)"=enum32{"Laser ON", "Laser OFF", "Interlace"}."Interlace" ("Value (Signaling)")) -> ()  [unwired: 2 in, 2 out]
          }
        }
      }
      event #10 {
        w1360 = i16 1 ("f")
        n483 = event-data() -> ()  [unwired: 7 out]
        n484 = local write "Trap 1 (ON/OFF)"("Trap 1 ON") -> ()
        n485 = local write "Trap 2 (ON/OFF)"("Trap 2 ON") -> ()
        n486 = Boolean To (0,1)(Boolean="Trap 3 ON") -> (0, 1=w1361:i16)
        n487 = Boolean To (0,1)(Boolean="Trap 1 ON") -> (0, 1=w1362:i16)
        n488 = Boolean To (0,1)(Boolean="Trap 2 ON") -> (0, 1=w1363:i16)
        n489 = Select(t=w1363, s="Trap ON/OFF X or Y Amp?", f=w1360) -> (s? t:f=w1358:i16)
        n490 = Select(t=w1362, s="Trap ON/OFF X or Y Amp?", f=w1360) -> (s? t:f=w1359:i16)
        n491 = Select(t=w1361, s="Trap ON/OFF X or Y Amp?", f=w1360) -> (s? t:f=w1357:i16)
        n492 = Select(t=w1360, s="Trap ON/OFF X or Y Amp?", f=w1363) -> (s? t:f=w1355:i16)
        n493 = Select(t=w1360, s="Trap ON/OFF X or Y Amp?", f=w1362) -> (s? t:f=w1356:i16)
        n494 = Select(t=w1360, s="Trap ON/OFF X or Y Amp?", f=w1361) -> (s? t:f=w1354:i16)
        n495 = And(x="All FB On/Off", y="Feedback On/Off") -> (x .and. y?=w1352:cluster{"Set 1":bool, "Set 2":bool})
        n496 = local read "BD 1 Amplitude 1 (%)"() -> (w1372:dbl)
        n497 = local read "BD 1 Amplitude 2 (%)"() -> (w1371:dbl)
        n498 = local read "BD 1 Amplitude 3 (%)"() -> (w1370:dbl)
        n499 = Unbundle By Name(w1352) -> ("Set 1"=w1347:bool, "Set 2"=w1344:bool)
        n500 = local read "Y RF Amplitude Limits (%)"() -> (w1340:T12)
        n501 = local read "X RF Amplitude Limits (%)"() -> (w1341:T12)
        n502 = local read "BD 2 Amplitude 1 (%)"() -> (w1373:dbl)
        n503 = local read "BD 2 Amplitude 2 (%)"() -> (w1374:dbl)
        n504 = local read "BD 2 Amplitude 3 (%)"() -> (w1375:dbl)
        n505 = And(x="Trap 2 ON", y=w1344) -> (x .and. y?=w1342:bool)
        n506 = And(x="Trap 1 ON", y=w1347) -> (x .and. y?=w1345:bool)
        n507 = Multiply(x=w1359, y=w1372) -> (x*y=w1367:dbl)
        n508 = Multiply(x=w1371, y=w1358) -> (x*y=w1365:dbl)
        n509 = Multiply(x=w1370, y=w1357) -> (x*y=w1366:dbl)
        n510 = Multiply(x=w1373, y=w1356) -> (x*y=w1376:dbl)
        n511 = Multiply(x=w1374, y=w1355) -> (x*y=w1377:dbl)
        n512 = Multiply(x=w1375, y=w1354) -> (x*y=w1378:dbl)
        n513 = call "set RF board amplitude - interlace.vi"("Board 2 Amplitude Limits"=w1340, "Board 1 Amplitude Limits"=w1341, "error in"=w1368, "FPGA VI Reference In"=w1369, "Board 2 Amplitude 3 (%)"=w1378, "Board 1 Amplitude 3 (%)"=w1366, "Board 2 Amplitude 2 (%)"=w1377, "Board 2 Amplitude 1 (%)"=w1376, "Board 1 Amplitude 2 (%)"=w1365, "Board 1 Amplitude 1 (%)"=w1367) -> ("error out"=w1349:errorcluster, "FPGA VI Reference Out"=w1350:T15)
        n514 = xnode "Read/Write Control"("FPGA VI Reference In"=w1350, "error in"=w1349, "FB On/Off Set 1"=w1345, "FB On/Off Set 2"=w1342) -> ("error out"=w1348:errorcluster)  [unwired: 1 out]
      }
      event #11 {
        n515 = event-data() -> ()  [unwired: 7 out]
        n516 = local read "Current Stage  Position"() -> (w1439:cluster{dbl, dbl, dbl})
        n517 = local read "Saved Stage Positions"() -> (w1438:T4)
        n518 = Bundle By Name(cluster=w1438, "Position 1"=w1439) -> (w1437:T4)
        n519 = local write "Saved Stage Positions"(w1437) -> ()
      }
      event #12 {
        n520 = event-data() -> ()  [unwired: 7 out]
        n521 = local read "Current Stage  Position"() -> (w1443:cluster{dbl, dbl, dbl})
        n522 = local read "Saved Stage Positions"() -> (w1442:T4)
        n523 = Bundle By Name(cluster=w1442, "Position 2"=w1443) -> (w1441:T4)
        n524 = local write "Saved Stage Positions"(w1441) -> ()
      }
      event #13 {
        n525 = event-data() -> ()  [unwired: 7 out]
        n526 = local read "Saved Stage Positions"() -> (w1447:T4)
        n527 = local read "Current Stage  Position"() -> (w1446:cluster{dbl, dbl, dbl})
        n528 = Bundle By Name(cluster=w1447, "Position 3"=w1446) -> (w1445:T4)
        n529 = local write "Saved Stage Positions"(w1445) -> ()
      }
      event #14 {
        n530 = event-data() -> ()  [unwired: 7 out]
        n531 = local read "Current Stage  Position"() -> (w1450:cluster{dbl, dbl, dbl})
        n532 = local read "Saved Stage Positions"() -> (w1451:T4)
        n533 = Bundle By Name(cluster=w1451, "Position 4"=w1450) -> (w1449:T4)
        n534 = local write "Saved Stage Positions"(w1449) -> ()
      }
      event #15 {
        n535 = event-data() -> ()  [unwired: 7 out]
        n536 = property on="Saved AOD Raster Scan Parameter Sets" class="Arr (strict)"() -> ("Index Values"=w1461:u32[])  [unwired: 2 in, 2 out]
        n537 = Index Array(array=w1461, index=0) -> (element=w1458:u32)
        n538 = Index Array(array="Saved AOD Raster Scan Parameter Sets", index=w1458) -> (element=w1457:T26)
        n539 = Unbundle By Name(w1457) -> ("Scan Range AOD (nm) 2"=w1456:dbl, "Step Size AOD (nm) 2"=w1455:dbl, "Scan Speed AOD (nm/s) 2"=w1454:dbl, "Number of scans (AOD) 2"=w1453:u16)
        n540 = flat-sequence {
          tunnel: w1456 -> [w1465]
          tunnel: w1455 -> [w1464]
          tunnel: w1454 -> [w1463]
          tunnel: w1453 -> [w1466]
          frame #0 {
            n541 = local write "Scan Speed (nm/s)"(w1463) -> ()
            n542 = local write "Scan Range (nm)"(w1465) -> ()
            n543 = local write "Step Size (nm)"(w1464) -> ()
          }
          frame #1 {
            n544 = property on="Number of F/B Scans (AOD)" class="DigNum (strict)"("Val(Sgnl)"=w1466) -> ()  [unwired: 2 in, 2 out]
          }
        }
      }
      event #16 {
        n545 = event-data() -> ()  [unwired: 7 out]
        n546 = property on="Trap 2 ON" class="Bool (strict)"("Val(Sgnl)"="Trap 2 (ON/OFF)") -> ()  [unwired: 2 in, 2 out]
        n547 = property on="Trap 1 ON" class="Bool (strict)"("Val(Sgnl)"="Trap 1 (ON/OFF)") -> ()  [unwired: 2 in, 2 out]
      }
      event #17 {
        n548 = event-data() -> ()  [unwired: 7 out]
        n549 = local read "DIO count 3 (ticks)"() -> (w1479:u32)
        n550 = local read "DIO count 1 (ticks)"() -> (w1481:u32)
        n551 = local read "DIO count 2 (ticks)"() -> (w1480:u32)
        n552 = To Unsigned Byte Integer(number="Not-Interlacing Set") -> (unsigned 8bit integer=w1470:u8)
        n553 = Add(x=w1470, y=u8 1) -> (x+y=w1474:u8)
        n554 = xnode "Read/Write Control"("FPGA VI Reference In"=w1485, "error in"=w1483, "DIO count 1 (ticks)"=w1481, "DIO count 2 (ticks)"=w1480, "DIO count 3 (ticks)"=w1479, "Interlace ON/OFF"="Interlace", "Number Interlace Cycles"="Number Interlace Sets", "Interlace Off Parameters"=w1474) -> ("error out"=w1484:errorcluster)  [unwired: 1 out]
        n555 = Build Array(w1481, w1480, w1479) -> (w1472:u32[])
        n556 = Split 1D Array(array=w1472, index="Number Interlace Sets") -> (first subarray=w1482:u32[])  [unwired: 1 out]
        n557 = Index Array(array=w1472, index=w1470) -> (element=w1471:u32)
        n558 = Add Array Elements(numeric array=w1482) -> (sum=w1476:u32)
        n559 = Select(t=w1476, s="Interlace", f=w1471) -> (s? t:f=→"Total Counts (ticks)":u32)
      }
      event #18 {
        n560 = event-data() -> ()  [unwired: 7 out]
        n561 = Unbundle By Name("Reset Feedback") -> ("Set 1"=w1621:bool, "Set 2"=w1620:bool)
        n562 = xnode "Read/Write Control"("FPGA VI Reference In"=w1623, "error in"=w1618, "FB Reset Set 1"=w1621, "FB Reset Set 2"=w1620) -> ("error out"=w1619:errorcluster)  [unwired: 1 out]
      }
      event #19 {
        n563 = event-data() -> ()  [unwired: 7 out]
        n564 = Unbundle By Name("PID Gains") -> ("Set 1"=w1684:T10, "Set 2"=w1683:T10)
        n565 = xnode "Read/Write Control"("FPGA VI Reference In"=w1685, "error in"=w1681, "FB Gains Set 1"=w1684, "FB Gains Set 2"=w1683) -> ("error out"=w1682:errorcluster)  [unwired: 1 out]
      }
      event #20 {
        n566 = event-data() -> ()  [unwired: 7 out]
        n567 = xnode "Read/Write Control"("FPGA VI Reference In"=w1728, "error in"=w1724) -> ("FPGA VI Reference Out"=w1727:T15, "error out"=w1726:errorcluster, "AI2 Y Sum Set 1"=w1735:i16, "AI2 Y Sum Set 2"=w1734:i16)
        n568 = Cluster To Array(cluster="AI2 to Setpoint") -> (array=w1738:bool[])
        n569 = local read "AI2 (V)"() -> (w1736:cluster{"Set 1":dbl, "Set 2":dbl})
        n570 = Or Array Elements(Boolean array=w1738) -> (logical OR=w1739:bool)
        n571 = Bundle By Name(cluster=w1736, "Set 1"=w1735, "Set 2"=w1734) -> (w1733:cluster{"Set 1":dbl, "Set 2":dbl})
        n572 = Divide(x=w1733, y=3276.7) -> (x/y=w1732:cluster{"Set 1":dbl, "Set 2":dbl})
        "AI2 (V)" <- w1732
        n573 = case shown="True" w1739 {
          tunnel: [w1801 w1818] -> w1731
          tunnel: "AI2 to Setpoint" -> [_ w1814]
          tunnel: "Setpoints (V)" -> [w1802 w1817]
          tunnel: w1732 -> [_ w1811]
          frame #0 {
            n574 = Multiply(x=3276.7, y=w1802) -> (x*y=w1803:cluster{"Set 1":dbl, "Set 2":dbl})
            n575 = To Word Integer(number=w1803) -> (16bit integer=w1801:cluster{"Set 1":i16, "Set 2":i16})
          }
          frame #1 {
            n576 = Unbundle By Name(w1811) -> ("Set 1"=w1810:dbl, "Set 2"=w1809:dbl)
            n577 = Unbundle By Name(w1817) -> ("Set 1"=w1816:dbl, "Set 2"=w1815:dbl)
            n578 = Unbundle By Name(w1814) -> ("Set 1"=w1813:bool, "Set 2"=w1812:bool)
            n579 = Select(t=w1810, s=w1813, f=w1816) -> (s? t:f=w1808:dbl)
            n580 = Select(t=w1809, s=w1812, f=w1815) -> (s? t:f=w1807:dbl)
            n581 = Bundle By Name(cluster=w1817, "Set 1"=w1808, "Set 2"=w1807) -> (w1805:cluster{"Set 1":dbl, "Set 2":dbl})
            n582 = Multiply(x=3276.7, y=w1805) -> (x*y=w1806:cluster{"Set 1":dbl, "Set 2":dbl})
            n583 = local write "Setpoints (V)"(w1805) -> ()
            n584 = To Word Integer(number=w1806) -> (16bit integer=w1818:cluster{"Set 1":i16, "Set 2":i16})
          }
        }
        n585 = Unbundle By Name(w1731) -> ("Set 1"=w1730:i16, "Set 2"=w1729:i16)
        n586 = xnode "Read/Write Control"("FPGA VI Reference In"=w1727, "error in"=w1726, "FB Setpoint Set 1"=w1730, "FB Setpoint Set 2"=w1729) -> ("error out"=w1725:errorcluster)  [unwired: 1 out]
      }
      event #21 {
        n587 = event-data() -> ()  [unwired: 7 out]
        n588 = xnode "Read/Write Control"("FPGA VI Reference In"=w1878, "error in"=w1876, "Invert GI"="Invert GI", "Invert GI 2"="Invert GI") -> ("error out"=w1877:errorcluster)  [unwired: 1 out]
      }
      event #22 {
        n589 = event-data() -> ()  [unwired: 7 out]
        n590 = local read "Green FB Setpoint (mV)"() -> (w1942:dbl)
        n591 = local read "Current When FB OFF (%)"() -> (w1945:dbl)
        n592 = Multiply(x=w1942, y=3.2767) -> (x*y=w1941:dbl)
        n593 = Multiply(x=w1945, y=655.35) -> (x*y=w1946:dbl)
        n594 = To Unsigned Word Integer(number=w1946) -> (unsigned 16bit integer=w1944:u16)
        n595 = local read "Green int current ON count adj"() -> (w1949:u32)
        n596 = local read "Green FB Gains"() -> (w1948:T10)
        n597 = local read "Green Laser ON/Interlacing"() -> (w1939:bool)
        n598 = local read "Green laser mode"() -> (w1938:enum32{"Laser ON", "Laser OFF", "Interlace"})
        n599 = local read "Green FB On/Off"() -> (w1950:bool)
        n600 = Equal?(x=w1938, y=enum32{"Laser ON", "Laser OFF", "Interlace"}."Interlace") -> (x = y?=w1936:bool)
        n601 = Compound Arithmetic op=AND(w1936, w1950, w1939) -> (w1940:bool)
        n602 = xnode "Read/Write Control"("FPGA VI Reference In"=w1953, "error in"=w1952, "Green FB Setpoint"=w1941, "Green FB On/Off"=w1940, "Current Out"=w1944, "Green int current ON count adj"=w1949, "Green FB Gains"=w1948) -> ("error out"=w1951:errorcluster)  [unwired: 1 out]
      }
      event #23 {
        n603 = event-data() -> ()  [unwired: 7 out]
        n604 = case shown="True" "Green Laser ON/Interlacing" {
          tunnel: "Green laser mode" -> [_ w2071]
          tunnel: [enum32{"Laser ON", "Laser OFF", "Interlace"}."Laser OFF" ("Green laser mode") w2071] -> w2059
          tunnel: [FALSE w2067] -> w2058
          frame #0 {
          }
          frame #1 {
            n605 = local read "Green FB On/Off"() -> (w2068:bool)
            n606 = Equal?(x=w2071, y=enum32{"Laser ON", "Laser OFF", "Interlace"}."Interlace") -> (x = y?=w2069:bool)
            n607 = And(x=w2069, y=w2068) -> (x .and. y?=w2067:bool)
          }
        }
        n608 = xnode "Read/Write Control"("FPGA VI Reference In"=w2064, "error in"=w2062, "Operating Mode"=w2059, "Operating Mode 2"=w2059, "Green FB On/Off"=w2058) -> ("error out"=w2063:errorcluster)  [unwired: 1 out]
      }
      event #24 {
        n609 = event-data() -> ()  [unwired: 7 out]
        n610 = local read "Phase Adj. (APD Gate)"() -> (w2147:i16)
        n611 = Negate(x=w2147) -> (-x=w2155:i16)
        n612 = Select(t=w2155, s="- phase (APD Gate)", f=w2147) -> (s? t:f=w2154:i16)
        n613 = Or(x="- phase (APD Gate)", y="+ phase (APD Gate)") -> (x .or. y?=w2150:bool)
        n614 = xnode "Read/Write Control"("FPGA VI Reference In"=w2157, "error in"=w2156, "Phase count adjustment (APD Gate)"=w2154) -> ("FPGA VI Reference Out"=w2152:T15, "error out"=w2153:errorcluster)
        n615 = xnode "Read/Write Control"("FPGA VI Reference In"=w2152, "error in"=w2153, "+ phase (APD Gate)"=w2150) -> ("error out"=w2151:errorcluster)  [unwired: 1 out]
      }
      event #25 {
        n616 = event-data() -> ()  [unwired: 7 out]
        n617 = local read "Phase Adj. (APD Acq)"() -> (w2233:i16)
        n618 = Negate(x=w2233) -> (-x=w2239:i16)
        n619 = Select(t=w2239, s="+ phase (APD Acq)", f=w2233) -> (s? t:f=w2238:i16)
        n620 = Or(x="+ phase (APD Acq)", y="- phase (APD Acq)") -> (x .or. y?=w2234:bool)
        n621 = xnode "Read/Write Control"("FPGA VI Reference In"=w2241, "error in"=w2240, "Phase Count Adjustment (APD Acq)"=w2238) -> ("FPGA VI Reference Out"=w2236:T15, "error out"=w2237:errorcluster)
        n622 = xnode "Read/Write Control"("FPGA VI Reference In"=w2236, "error in"=w2237, "+ phase (APD Acq)"=w2234) -> ("error out"=w2235:errorcluster)  [unwired: 1 out]
      }
      event #26 {
        n623 = event-data() -> ()  [unwired: 7 out]
        n624 = Negate(x="Phase adj. (GI)") -> (-x=w2323:i16)
        n625 = Select(t=w2323, s="+ phase (GI)", f="Phase adj. (GI)") -> (s? t:f=w2322:i16)
        n626 = Or(x="+ phase (GI)", y="- phase (GI)") -> (x .or. y?=w2318:bool)
        n627 = xnode "Read/Write Control"("FPGA VI Reference In"=w2325, "error in"=w2324, "Phase count adjustment (GI)"=w2322) -> ("FPGA VI Reference Out"=w2320:T15, "error out"=w2321:errorcluster)
        n628 = xnode "Read/Write Control"("FPGA VI Reference In"=w2320, "error in"=w2321, "+ phase (GI)"=w2318) -> ("error out"=w2319:errorcluster)  [unwired: 1 out]
      }
      event #27 {
        n629 = event-data() -> ()  [unwired: 7 out]
        n630 = Negate(x="Phase adj. (GI) 2") -> (-x=w2407:i16)
        n631 = Select(t=w2407, s="+ phase (GI) 2", f="Phase adj. (GI) 2") -> (s? t:f=w2406:i16)
        n632 = Or(x="+ phase (GI) 2", y="- phase (GI) 2") -> (x .or. y?=w2402:bool)
        n633 = xnode "Read/Write Control"("FPGA VI Reference In"=w2409, "error in"=w2408, "Phase count adjustment (GI) 2"=w2406) -> ("FPGA VI Reference Out"=w2404:T15, "error out"=w2405:errorcluster)
        n634 = xnode "Read/Write Control"("FPGA VI Reference In"=w2404, "error in"=w2405, "+ phase (GI) 2"=w2402) -> ("error out"=w2403:errorcluster)  [unwired: 1 out]
      }
      event #28 {
        n635 = event-data() -> ()  [unwired: 7 out]
        n636 = Negate(x="Phase adj. (Green FB)") -> (-x=w2491:i16)
        n637 = Select(t=w2491, s="+ phase (Green FB)", f="Phase adj. (Green FB)") -> (s? t:f=w2490:i16)
        n638 = Or(x="+ phase (Green FB)", y="- phase (Green FB)") -> (x .or. y?=w2486:bool)
        n639 = xnode "Read/Write Control"("FPGA VI Reference In"=w2493, "error in"=w2492, "Phase count adjustment (Green FB)"=w2490) -> ("FPGA VI Reference Out"=w2488:T15, "error out"=w2489:errorcluster)
        n640 = xnode "Read/Write Control"("FPGA VI Reference In"=w2488, "error in"=w2489, "+ phase (Green FB)"=w2486) -> ("error out"=w2487:errorcluster)  [unwired: 1 out]
      }
      event #29 {
        n641 = event-data() -> ()  [unwired: 7 out]
        n642 = local read "Invert APD Gate"() -> (w2583:bool)
        n643 = local read "APD Gate ON Count"() -> (w2582:u32)
        n644 = local read "APD Gate OFF Count"() -> (w2581:u32)
        n645 = local read "APD Integration Time (s)"() -> (w2567:dbl)
        n646 = local read "APD Gate"() -> (w2580:enum32{"ON", "OFF", "Interlace"})
        n647 = Multiply(x=w2567, y=40000000.0) -> (x*y=w2578:dbl)
        n648 = Reciprocal(x=w2567) -> (1/x=→"APD Acq Rate (Hz)":dbl)
        n649 = To Unsigned Long Integer(number=w2578) -> (unsigned 32bit integer=w2577:u32)
        n650 = local read "DMA Update Period (s)"() -> (w2568:dbl)
        n651 = Divide(x=w2568, y=w2567) -> (x/y=w2571:dbl)
        n652 = local read "APD 1 AO offset"() -> (w2573:i16)
        n653 = local read "APD 2 AO offset"() -> (w2572:i16)
        n654 = local read "APD 1 AO Mult."() -> (w2575:i16)
        n655 = local read "APD 2 AO Mult."() -> (w2574:i16)
        n656 = Multiply(x=2.0, y=w2571) -> (x*y=w2570:dbl)
        n657 = local write "APD Samples/FIFO Acq."(w2571) -> ()
        n658 = local write "APD Elements/DMA read"(w2570) -> ()
        n659 = xnode "Read/Write Control"("FPGA VI Reference In"=w2586, "error in"=w2585, "Invert APD Gate"=w2583, "APD Gate ON Count"=w2582, "APD Gate OFF Count"=w2581, "APD Acq Rate Count"=w2577, "APD Gate Operating Mode"=w2580, "APD 1 AO scale factor"=w2575, "APD 2 AO scale factor"=w2574, "APD 1 AO offset"=w2573, "APD 2 AO offset"=w2572) -> ("error out"=w2584:errorcluster)  [unwired: 1 out]
      }
      event #30 {
        n660 = event-data() -> ()  [unwired: 7 out]
        n661 = xnode "Read/Write Control"("FPGA VI Reference In"=w2781, "error in"=w2779, "Green interlace ON count"="GI Frequency, ON count", "Green interlace OFF count"="GI Frequency, OFF count", "Green interlace ON count 2"="GI Frequency, ON count", "Green interlace OFF count 2"="GI Frequency, OFF count", "Green FB Count"="Green FB Count") -> ("error out"=w2780:errorcluster)  [unwired: 1 out]
      }
      event #31 {
        w2949 = 123.0  # AOM cal (nm/MHz)
        n662 = event-data() -> ()  [unwired: 7 out]
        n663 = local read "BD 1 Frequency 1 (MHz)"() -> (w2932:dbl)
        n664 = local read "BD 2 Frequency 1 (MHz)"() -> (w2938:dbl)
        n665 = local read "X RF Frequency Limits (MHz)"() -> (w2936:T12)
        n666 = local read "Y RF Frequency Limits (MHz)"() -> (w2933:T12)
        n667 = local read "AOM X Cal (nm/MHz)"() -> (w2924:dbl)
        n668 = Negate(x="Scan Range (nm)") -> (-x=w2901:dbl)
        n669 = Divide(x=w2901, y=w2924) -> (x/y=w2905:dbl)
        n670 = Select(t=w2936, s="Scan BD", f=w2933) -> (s? t:f=w2935:T12)
        n671 = Select(t=w2932, s="Scan BD", f=w2938) -> (s? t:f=w2937:dbl)
        n672 = Unbundle By Name(w2935) -> ("Maximum"=w2944:dbl, "Minimum"=w2943:dbl)
        n673 = Add(x=w2905, y=w2937) -> (x+y=w2941:dbl)
        n674 = Divide(x=w2901, y="Step Size (nm)") -> (x/y=w2921:dbl)
        n675 = Divide(x="Step Size (nm)", y=w2924) -> (x/y=w2930:dbl)
        n676 = Absolute Value(x=w2921) -> (abs(x)=w2904:dbl)
        n677 = Sign(1:w2901) -> (0:w2902:dbl)
        n678 = In Range and Coerce(upper limit=w2944, x=w2941, lower limit=w2943) -> (coerced(x)=w2940:dbl, In Range?=w2942:bool)
        n679 = To Unsigned Quad Integer(1:w2904) -> (0:w2920:u64)
        "Scan steps (AOD)" <- w2920
        n680 = call "IR AOM freq to word.vi"("Frequency In (MHz)"=w2930) -> ("Frequency Word Out (double)"=w2927:dbl)
        n681 = Multiply(x=w2902, y=w2927) -> (x*y=w2903:dbl)
        n682 = Subtract(x=w2941, y=w2940) -> (x-y=w2939:dbl)
        n683 = To Quad Integer(1:w2903) -> (0:w2926:i64)
        "Incr. int (AOD)" <- w2926
        n684 = Subtract(x=w2905, y=w2939) -> (x-y=w2925:dbl)
        "Scan Range (MHz)" <- w2925
        n685 = Select(t=w2905, s=w2942, f=w2925) -> (s? t:f=w2945:dbl)
        n686 = Multiply(x=w2925, y=w2924) -> (x*y=w2923:dbl)
        n687 = Decrement(x=w2920) -> (x-1=w2973:u64)
        n688 = Negate(x=w2923) -> (-x=w2919:dbl)
        n689 = local write "Scan Range (nm)"(w2919) -> ()
        n690 = Divide(x=w2945, y=w2973) -> (x/y=w2929:dbl)
        "Scan Increment (MHz)" <- w2929
        n691 = call "IR AOM freq to word.vi"("Frequency In (MHz)"=w2929) -> ("Frequency Word Out (double)"=w2928:dbl)
        n692 = Divide(x="Step Size (nm)", y="Scan Speed (nm/s)") -> (x/y=w2916:dbl)
        n693 = To Quad Integer(1:w2928) -> ()  [unwired: 1 out]
        n694 = local read "Number Interlace Sets"() -> (w2899:u8)
        n695 = local read "AI Count (ticks)"() -> (w2900:u32)
        n696 = local read "Total Counts (ticks)"() -> (w2898:u32)
        n697 = local read "# Samples/trap"() -> (w2931:dbl)
        n698 = Multiply(x=w2900, y=w2899) -> (x*y=w2897:u32)
        n699 = Divide(x=w2898, y=w2897) -> (x/y=w2896:dbl)
        n700 = Select(t=w2932, s="Scan BD", f=w2938) -> (s? t:f=w2970:dbl)
        "Initial freq. (MHz)" <- w2970
        n701 = Add(x=w2945, y=w2970) -> (x+y=→"Final freq. (MHz)":dbl)
        n702 = Divide(x=w2898, y=40000000.0) -> (x/y=w2915:dbl)
        n703 = Divide(x=w2916, y=w2915) -> (x/y=w2914:dbl)
        n704 = To Unsigned Quad Integer(1:w2914) -> (0:w2913:u64)
        "Cycles/step (AOD)" <- w2913
        n705 = xnode "Read/Write Control"("FPGA VI Reference In"=w2981, "error in"=w2980, "Scan steps"=w2920, "Number of scans"="Number of F/B Scans (AOD)", "Cycles per step"=w2913, "Scan freq.  increment"=w2926, "Scan BD"="Scan BD") -> ("error out"=w2979:errorcluster)  [unwired: 1 out]
        n706 = Multiply(x=w2920, y=w2913) -> (x*y=w2974:u64)
        n707 = Multiply(x=w2974, y=u64 2) -> (x*y=w2895:u64)
        n708 = Multiply(x=w2896, y=w2895) -> (x*y=w2894:dbl)
        "Data points/scan (f/b)" <- w2894
        n709 = Multiply(x=w2894, y="Number of F/B Scans (AOD)") -> (x*y=w2977:dbl)
        "Data points/scans" <- w2977
        n710 = Divide(x=w2977, y=w2931) -> (x/y=→"N sets should be saved":dbl)
        n711 = Multiply(x=w2974, y=w2915) -> (x*y=w2912:dbl)
        "Time/Scan (s) (AOD)" <- w2912
        n712 = Select(t=w2945, s="Scan BD", f=0.0) -> (s? t:f=w2971:dbl)
        n713 = Select(t=0.0, s="Scan BD", f=w2945) -> (s? t:f=w2967:dbl)
        n714 = local read "BD 2 Frequency 2 (MHz)"() -> (w2963:dbl)
        n715 = local read "BD 1 Frequency 2 (MHz)"() -> (w2966:dbl)
        n716 = Add(x=w2967, y=w2938) -> (x+y=w2964:dbl)
        n717 = Add(x=w2932, y=w2971) -> (x+y=w2965:dbl)
        n718 = Multiply(x=w2912, y=2.0) -> (x*y=w2911:dbl)
        n719 = Multiply(x=w2911, y="Number of F/B Scans (AOD)") -> (x*y=w2908:dbl)
        n720 = Divide(x=w2908, y=60.0) -> (x/y=→"Time to Finish All (min)":dbl)
        n721 = Add(x="Trap 2 Bead Size (nm)", y="Trap 1 Bead Size (nm)") -> (x+y=w2953:dbl)
        n722 = Divide(x=w2953, y=2.0) -> (x/y=w2947:dbl)
        n723 = Subtract(x=w2964, y=w2963) -> (x-y=w2961:dbl)
        n724 = Subtract(x=w2965, y=w2966) -> (x-y=w2962:dbl)
        n725 = local read "Initial delta (MHz)"() -> (w2950:dbl)
        n726 = Square(x=w2961) -> (x^2=w2960:dbl)
        n727 = Square(x=w2962) -> (x^2=w2959:dbl)
        n728 = Add(x=w2959, y=w2960) -> (x+y=w2958:dbl)
        n729 = Square Root(x=w2958) -> (sqrt(x)=w2957:dbl)
        "Final delta (MHz)" <- w2957
        n730 = Multiply(x=w2949, y=w2957) -> (x*y=w2956:dbl)
        n731 = Multiply(x=w2950, y=w2949) -> (x*y=w2948:dbl)
        n732 = Subtract(x=w2948, y=w2947) -> (x-y=→"Initial sep (nm)":dbl)
        n733 = Subtract(x=w2956, y=w2947) -> (x-y=→"Final sep (nm)":dbl)
      }
      event #32 {
        n734 = event-data() -> ()  [unwired: 7 out]
        n735 = local read "Freq or Amp switch first"() -> (w3068:bool)
        n736 = local read "Freq switch delay"() -> (w3071:u16)
        n737 = local read "Amp switch delay"() -> (w3069:u16)
        n738 = local read "Swap F1 and F2"() -> (w3070:bool)
        n739 = xnode "Read/Write Control"("FPGA VI Reference In"=w3074, "error in"=w3073, "Freq switch delay"=w3071, "Swap F1 and F2"=w3070, "Amp switch delay"=w3069, "Freq or Amp switch first"=w3068) -> ("error out"=w3072:errorcluster)  [unwired: 1 out]
      }
      event #33 {
        w3171 = 32767.0 ("y")
        n740 = event-data() -> ()  [unwired: 7 out]
        n741 = Select(t="Scan lines (y)", s="2D or 1D Scan", f="Number of scans (MCL)") -> (s? t:f=w3176:u64)
        n742 = Decrement(x="Scan steps (MCL)") -> (x-1=w3192:u64)
        n743 = Divide(x="Scan Range (V)\n(of steps)", y=w3192) -> (x/y=w3191:dbl)
        "Desired Scan Incr (V)" <- w3191
        n744 = local read "APD Integration Time (s)"() -> (w3184:dbl)
        n745 = Multiply(x=w3191, y=w3171) -> (x*y=w3200:dbl)
        n746 = Divide(x=w3200, y=10.0) -> (x/y=w3190:dbl)
        "Desired incr (int)" <- w3190
        n747 = local read "Update Count (MCL)"() -> (w3196:u32)
        n748 = Round Toward -Infinity(1:w3190) -> (0:w3199:dbl)
        n749 = To Word Integer(number=w3199) -> (16bit integer=w3174:i16)
        "Actual Incr. int (MCL)" <- w3174
        n750 = Multiply(x=w3184, y=40000000.0) -> (x*y=w3197:dbl)
        n751 = Divide(x=w3197, y=w3196) -> (x/y=w3195:dbl)
        n752 = Multiply(x=i16 10, y=w3174) -> (x*y=w3172:i16)
        n753 = Multiply(x="N APD Samp/step", y=w3195) -> (x*y=w3194:dbl)
        "Cycles/step (MCL)" <- w3194
        n754 = Divide(x=w3172, y=w3171) -> (x/y=→"Actual MCL Inc (V)":dbl)
        n755 = Multiply(x="N APD Samp/step", y="Scan steps (MCL)") -> (x*y=w3186:dbl)
        n756 = local read "APD Samples/FIFO Acq."() -> (w3183:dbl)
        n757 = Multiply(x=w3186, y=u64 2) -> (x*y=w3185:dbl)
        "Data points/scan (f+b)" <- w3185
        n758 = Multiply(x=w3185, y=w3176) -> (x*y=w3203:dbl)
        "Data points/scans (MCL)" <- w3203
        n759 = Multiply(x=w3184, y=w3185) -> (x*y=w3177:dbl)
        "Time/f+b scan (s) (MCL)" <- w3177
        n760 = Divide(x=w3203, y=w3183) -> (x/y=→"N sets should be saved (MCL)":dbl)
        n761 = Multiply(x=w3177, y=w3176) -> (x*y=→"Total Time (s)":dbl)
        n762 = Not(x="Fast Scan Dir") -> (.not. x?=w3181:bool)
        n763 = xnode "Read/Write Control"("FPGA VI Reference In"=w3207, "error in"=w3206, "Scan steps (MCL)"="Scan steps (MCL)", "Number of scans (MCL)"=w3176, "Cycles per step (MCL)"=w3194, "Scan freq.  increment (MCL)"=w3174, "1D or 2D Scan?"="2D or 1D Scan", "MCL Scan Axis"=w3181, "Cont. Scan (MCL)"="Continuous MCL Scanning") -> ("error out"=w3205:errorcluster)  [unwired: 1 out]
      }
      event #34 {
        w3344 = 1000.0 ("y")
        n764 = event-data() -> ()  [unwired: 7 out]
        n765 = local read "Save file name"() -> (w3369:path)
        n766 = local write "Read Cal"(FALSE ("Read Cal")) -> ()
        n767 = Strip Path(path=w3369) -> (stripped path=w3368:path)  [unwired: 1 out]
        n768 = Path To String(path=w3368) -> (string=w3367:string)
        n769 = Concatenate Strings(w3367, "\\current.cal" ("string")) -> (w3365:string)
        n770 = String To Path(string=w3365) -> (path=w3364:path)
        n771 = Open/Create/Replace File(file path (use dialog)=w3364, operation (0:open)=T25."open", access (0:read/write)=enum16{"read/write", "read-only", "write-only"}."read-only") -> (refnum out=w3372:refnum<file>, error out=w3358:errorcluster)  [unwired: 1 in, 3 out]
        n772 = Deny Access(4:w3358, 7:w3372) -> (0:w3357:errorcluster, 3:w3363:refnum<file>)  [unwired: 1 out]
        n773 = Read from Binary File(5:0.0, 8:w3357, 9:T24."big-endian, network order" ("byte order (0:big-endian, network order)"), 10:-1 ("count (1)"), 11:w3363) -> (0:w3356:errorcluster, 2:w3354:dbl[], 3:w3359:refnum<file>)  [unwired: 2 out]
        n774 = Array To Cluster(array=w3354) -> (cluster=w3353:T27)
        n775 = Unbundle(w3353) -> ("[0]"=w3352:dbl, "[1]"=w3351:dbl, "[2]"=w3350:dbl, "[3]"=w3349:dbl, "[4]"=w3348:dbl, "[5]"=w3347:dbl)
        n776 = Close File(refnum=w3359, error in=w3356) -> (error out=→"Read cal error":errorcluster)  [unwired: 1 out]
        n777 = Multiply(x=w3347, y=w3344) -> (x*y=w3345:dbl)
        n778 = local write "T2 kappa_x (pN/nm)"(w3349) -> ()
        n779 = local write "T1 kappa_x (pN/nm)"(w3350) -> ()
        n780 = local write "T1 alpha_x (nm/V)"(w3352) -> ()
        n781 = local write "T2 alpha_x (nm/V)"(w3351) -> ()
        n782 = Multiply(x=w3348, y=w3344) -> (x*y=w3346:dbl)
        n783 = local write "T1 offset_x (mV)"(w3346) -> ()
        n784 = local write "T2 offset_x (mV)"(w3345) -> ()
      }
      event #35 {
        n785 = event-data() -> ()  [unwired: 7 out]
        n786 = local write "MCL Scanning"(FALSE ("MCL Scanning")) -> ()
        n787 = xnode "Read/Write Control"("FPGA VI Reference In"=w3377, "error in"=w3376, "Abort scan (MCL)"="Abort MCL Scan") -> ("error out"=w3375:errorcluster)  [unwired: 1 out]
      }
      event #36 {
        n788 = event-data() -> ()  [unwired: 7 out]
        n789 = xnode "Read/Write Control"("FPGA VI Reference In"=w3418, "error in"=w3417, "MCL count"="Update Count (MCL)") -> ("error out"=w3416:errorcluster)  [unwired: 1 out]
      }
      event #37 {
        n790 = event-data() -> ()  [unwired: 7 out]
        n791 = Negate(x="Phase adjust (MCL)") -> (-x=w3463:i16)
        n792 = Select(t=w3463, s="- phase (MCL)", f="Phase adjust (MCL)") -> (s? t:f=w3461:i16)
        n793 = Or(x="- phase (MCL)", y="+ phase (MCL)") -> (x .or. y?=w3456:bool)
        n794 = xnode "Read/Write Control"("FPGA VI Reference In"=w3465, "error in"=w3464, "Phase count adjustment (MCL)"=w3461) -> ("FPGA VI Reference Out"=w3457:T15, "error out"=w3458:errorcluster)
        n795 = xnode "Read/Write Control"("FPGA VI Reference In"=w3457, "error in"=w3458, "+ phase (MCL)"=w3456) -> ("error out"=w3455:errorcluster)  [unwired: 1 out]
      }
      event #38 {
        n796 = event-data() -> ()  [unwired: 7 out]
        n797 = xnode "Read/Write Control"("FPGA VI Reference In"=w3542, "error in"=w3541, "Abort scan"="Abort AOD Scan") -> ("error out"=w3540:errorcluster)  [unwired: 1 out]
      }
      event #39 {
        n798 = event-data() -> ()  [unwired: 7 out]
        n799 = xnode "Read/Write Control"("FPGA VI Reference In"=w3583, "error in"=w3582, "Cont. Scan"="Continuous AOD Scanning") -> ("error out"=w3581:errorcluster)  [unwired: 1 out]
      }
      event #40 {
        n800 = event-data() -> ()  [unwired: 7 out]
        n801 = call "Create new save file.vi"("Insert"="", "Ext"=".dat" ("string"), "Index In"="Index") -> ("Path Out"=→"Save file name":path, "Index Out"=w3621:dbl)
        "Save index" <- w3621
        n802 = local write "Index"(w3621) -> ()
      }
      event #41 {
        w3636 = 10.0 ("y")
        w3635 = 32767.0 ("y")
        n803 = event-data() -> ()  [unwired: 7 out]
        n804 = local read "AO2"() -> (w3634:dbl)
        n805 = local read "AO1"() -> (w3631:dbl)
        n806 = Multiply(x=w3631, y=w3635) -> (x*y=w3630:dbl)
        n807 = Multiply(x=w3634, y=w3635) -> (x*y=w3633:dbl)
        n808 = Divide(x=w3630, y=w3636) -> (x/y=w3629:dbl)
        n809 = Divide(x=w3633, y=w3636) -> (x/y=w3632:dbl)
        n810 = To Word Integer(number=w3629) -> (16bit integer=w3637:i16)
        n811 = To Word Integer(number=w3632) -> (16bit integer=w3638:i16)
        n812 = xnode "Read/Write Control"("FPGA VI Reference In"=w3628, "error in"=w3627, "AO1"=w3637, "AO2"=w3638) -> ("error out"=w3626:errorcluster)  [unwired: 1 out]
      }
      event #42 {
        n813 = event-data() -> ()  [unwired: 7 out]
        n814 = local read "Syringe Pump Serial Port"() -> (w3694:refnum<visa-resource-name>)
        n815 = local read "Pump write delay (ms)"() -> (w3695:dbl)
        n816 = case shown="True" "Inject Top Channel" {
          tunnel: w3695 -> [w3700 w3708]
          tunnel: w3694 -> [w3697 w3707]
          frame #0 {
            n817 = flat-sequence {
              tunnel: w3697 -> [w3701]
              tunnel: [w3701] -> w3698
              tunnel: w3700 -> [_]
              tunnel: [w3704] -> w3699
              tunnel: w3698 -> [w3704]
              tunnel: w3699 -> [w3705]
              frame #0 {
                n818 = call "Write to pump.vi"("string"="enter pump1", "VISA resource name"=w3701) -> ()  [unwired: 1 out]
              }
              frame #1 {
                n819 = Wait (ms)(milliseconds to wait="Pump pause delay (ms)") -> ()  [unwired: 1 out]
              }
              frame #2 {
                n820 = call "Write to pump.vi"("string"="stop", "VISA resource name"=w3705) -> ()  [unwired: 1 out]
              }
            }
          }
          frame #1 {
            n821 = flat-sequence {
              tunnel: w3707 -> [w3717]
              tunnel: w3708 -> [w3712]
              tunnel: w3708 -> [w3719]
              tunnel: w3707 -> [w3720]
              frame #0 {
                n822 = local read "All Pump Parameters"() -> (w3711:T5)
                n823 = Unbundle By Name(w3711) -> ("Pump 1"=w3718:T28)
                n824 = call "Set pump parameters.vi"("Pump write delay (ms)"=w3712, "Volume (uL)"="Top Ch Inject Volume (uL)", "Rate (uL/h)"="Top Ch Inject Rate (ul/h)", "Units"=4.0, "Pump #"=1.0, "Pump Parameters In"=w3718, "VISA resource name"=w3717) -> ("Pump Parameters Out"=w3710:T28)  [unwired: 3 in]
                n825 = Bundle By Name(cluster=w3711, "Pump 1"=w3710) -> (w3709:T5)
                n826 = local write "All Pump Parameters"(w3709) -> ()
              }
              frame #1 {
                n827 = Wait (ms)(milliseconds to wait=w3719) -> ()  [unwired: 1 out]
              }
              frame #2 {
                n828 = call "Write to pump.vi"("string"="start", "VISA resource name"=w3720) -> ()  [unwired: 1 out]
              }
            }
          }
        }
      }
      event #43 {
        n829 = event-data() -> ()  [unwired: 7 out]
        n830 = local read "Pump write delay (ms)"() -> (w3723:dbl)
        n831 = case shown="False" "Inject Bottom Channel" {
          tunnel: w3723 -> [w3728 w3736]
          tunnel: "Syringe Pump Serial Port" -> [w3725 w3735]
          frame #0 {
            n832 = flat-sequence {
              tunnel: w3725 -> [w3729]
              tunnel: [w3729] -> w3726
              tunnel: w3728 -> [_]
              tunnel: [w3732] -> w3727
              tunnel: w3726 -> [w3732]
              tunnel: w3727 -> [w3733]
              frame #0 {
                n833 = call "Write to pump.vi"("string"="enter pump3", "VISA resource name"=w3729) -> ()  [unwired: 1 out]
              }
              frame #1 {
                n834 = local read "Pump pause delay (ms)"() -> (w3731:u32)
                n835 = Wait (ms)(milliseconds to wait=w3731) -> ()  [unwired: 1 out]
              }
              frame #2 {
                n836 = call "Write to pump.vi"("string"="stop", "VISA resource name"=w3733) -> ()  [unwired: 1 out]
              }
            }
          }
          frame #1 {
            n837 = flat-sequence {
              tunnel: w3735 -> [w3745]
              tunnel: w3736 -> [w3740]
              tunnel: w3736 -> [w3747]
              tunnel: w3735 -> [w3748]
              frame #0 {
                n838 = local read "All Pump Parameters"() -> (w3739:T5)
                n839 = Unbundle By Name(w3739) -> ("Pump 3"=w3746:T28)
                n840 = call "Set pump parameters.vi"("Pump write delay (ms)"=w3740, "Volume (uL)"="Bottom Ch Inject Volume (uL)", "Rate (uL/h)"="Bottom Ch Inject Rate (ul/h)", "Units"=4.0, "Pump #"=3.0, "Pump Parameters In"=w3746, "VISA resource name"=w3745) -> ("Pump Parameters Out"=w3738:T28)  [unwired: 3 in]
                n841 = Bundle By Name(cluster=w3739, "Pump 3"=w3738) -> (w3737:T5)
                n842 = local write "All Pump Parameters"(w3737) -> ()
              }
              frame #1 {
                n843 = Wait (ms)(milliseconds to wait=w3747) -> ()  [unwired: 1 out]
              }
              frame #2 {
                n844 = call "Write to pump.vi"("string"="start", "VISA resource name"=w3748) -> ()  [unwired: 1 out]
              }
            }
          }
        }
      }
      event #44 {
        n845 = event-data() -> ()  [unwired: 7 out]
        n846 = local read "Pump write delay (ms)"() -> (w3752:dbl)
        n847 = flat-sequence {
          tunnel: w3750 -> [w3765]
          tunnel: w3752 -> [w3761]
          tunnel: "Flush Center Channel" -> [_]
          tunnel: w3752 -> [w3767]
          tunnel: w3750 -> [w3768]
          frame #0 {
            n848 = local read "All Pump Parameters"() -> (w3760:T5)
            n849 = Multiply(x=60.0, y="Flush Center Ch Rate (ul/m)") -> (x*y=w3757:dbl)
            n850 = Unbundle By Name(w3760) -> ("Pump 2"=w3766:T28)
            n851 = call "Set pump parameters.vi"("Pump write delay (ms)"=w3761, "Volume (uL)"="Flush Center Ch Volume (uL)", "Rate (uL/h)"=w3757, "Units"=3.0, "Pump #"=2.0, "Pump Parameters In"=w3766, "VISA resource name"=w3765) -> ("Pump Parameters Out"=w3759:T28)  [unwired: 3 in]
            n852 = Bundle By Name(cluster=w3760, "Pump 2"=w3759) -> (w3758:T5)
            n853 = Add(x="Flush Center Ch Volume (uL)", y="Total Volume\nFlushed (uL)") -> (x+y=w3754:dbl)
            n854 = local write "All Pump Parameters"(w3758) -> ()
            n855 = local write "Total Volume\nFlushed (uL)"(w3754) -> ()
          }
          frame #1 {
            n856 = Wait (ms)(milliseconds to wait=w3767) -> ()  [unwired: 1 out]
          }
          frame #2 {
            n857 = call "Write to pump.vi"("string"="start", "VISA resource name"=w3768) -> ()  [unwired: 1 out]
          }
        }
        n858 = local read "Syringe Pump Serial Port"() -> (w3750:refnum<visa-resource-name>)
      }
    }
    "error out 2" <- w1039
    n859 = node-c288() -> ()  [unwired: 2 out]
  }
  n860 = timed-loop "Acquire Data" {
    tunnel: w77 -> [w3945]
    tunnel: w76 -> [w3944]
    tunnel: [w3982] -> w233
    tunnel: [w3976] -> w231
    timing: w130 -> [_]
    timing-out: [_] -> w129
    tunnel: w6 -> [w3777]
    tunnel: w2 -> [w3775]
    tunnel: w1 -> [w3774]
    stop <- "Stop All" stop-if-true
    w3827 = "NI_ChannelName" ("name")
    n861 = node-c288() -> ()  [unwired: 2 out]
    n862 = case "Reset data stream" shown="True" "Reset" {
      tunnel: w3945 -> [w6166 w6173]
      tunnel: w3944 -> [w6165 w6172]
      tunnel: [w6166 w6168] -> w3940
      tunnel: [w6165 w6167] -> w3939
      frame #0 {
      }
      frame #1 {
        w6171 = TRUE ("AI to FIFO")
        w6178 = FALSE ("AI to FIFO")
        n863 = local write "Overflow (data lost)"(FALSE ("Overflow (data lost)")) -> ()
        n864 = xnode "Read/Write Control"("FPGA VI Reference In"=w6173, "error in"=w6172, "AI to FIFO"=w6178, "APD to FIFO"=w6178) -> ("FPGA VI Reference Out"=w6176:T15, "error out"=w6177:errorcluster)
        n865 = xnode "Invoke Method"("FPGA VI Reference In"=w6176, "error in"=w6177) -> ("FPGA VI Reference Out"=w6174:T15, "error out"=w6175:errorcluster)
        n866 = xnode "Invoke Method"("FPGA VI Reference In"=w6174, "error in"=w6175) -> ("FPGA VI Reference Out"=w6170:T15, "error out"=w6169:errorcluster)
        n867 = xnode "Read/Write Control"("FPGA VI Reference In"=w6170, "error in"=w6169, "AI to FIFO"=w6171, "APD to FIFO"=w6171) -> ("FPGA VI Reference Out"=w6168:T15, "error out"=w6167:errorcluster)
      }
    }
    n868 = Or(x="Start AOD Scan", y="Trap Raster Scan") -> (x .or. y?=w3887:bool)
    n869 = And(x="Save scans", y=w3887) -> (x .and. y?=w3936:bool)
    n870 = case "Start AOM raster scan" shown="True" w3887 {
      tunnel: w3940 -> [w5405 w5414]
      tunnel: w3939 -> [w5404 w5413]
      tunnel: [w5405 w5407] -> w3938
      tunnel: [w5404 w5406] -> w3937
      frame #0 {
      }
      frame #1 {
        n871 = case shown="True" "Restart DMA? (AOD)" {
          tunnel: [w5780 w5781] -> w5408
          tunnel: [w5779 w5782] -> w5409
          tunnel: w5414 -> [w5780 w5788]
          tunnel: w5413 -> [w5779 w5787]
          frame #0 {
          }
          frame #1 {
            w5784 = FALSE ("AI to FIFO")
            n872 = xnode "Read/Write Control"("FPGA VI Reference In"=w5788, "error in"=w5787, "AI to FIFO"=w5784, "APD to FIFO"=w5784) -> ("FPGA VI Reference Out"=w5786:T15, "error out"=w5785:errorcluster)
            n873 = xnode "Invoke Method"("FPGA VI Reference In"=w5786, "error in"=w5785) -> ("FPGA VI Reference Out"=w5790:T15, "error out"=w5789:errorcluster)
            n874 = xnode "Invoke Method"("FPGA VI Reference In"=w5790, "error in"=w5789) -> ("FPGA VI Reference Out"=w5781:T15, "error out"=w5782:errorcluster)
            n875 = local write "Overflow (data lost)"(FALSE ("Overflow (data lost)")) -> ()
          }
        }
        n876 = case shown="True" "Move MCL Also?" {
          tunnel: w5409 -> [w5417 w5523]
          tunnel: w5408 -> [w5418 w5524]
          tunnel: [w5416 w5527] -> w5407
          tunnel: [w5415 w5526] -> w5406
          frame #0 {
            w5419 = TRUE ("AI to FIFO")
            n877 = xnode "Read/Write Control"("FPGA VI Reference In"=w5418, "error in"=w5417, "AI to FIFO"=w5419, "APD to FIFO"=w5419, "Start scan"=w5419) -> ("FPGA VI Reference Out"=w5416:T15, "error out"=w5415:errorcluster)
          }
          frame #1 {
            w5520 = FALSE ("1D or 2D Scan?")
            w5525 = TRUE ("AI to FIFO")
            # "Count for MCL loop"
            # "N total cycles"
            # "N steps"
            # "V_int"
            n878 = local read "Scan Range (nm)"() -> (w5502:dbl)
            n879 = local read "Number of F/B Scans (AOD)"() -> (w5519:u16)
            n880 = Sign(1:w5502) -> (0:w5501:dbl)
            n881 = Compound Arithmetic op=MULTIPLY(w5502, "MCL Step Position Ratio", "MCL/AOM Scale Tweak") -> (w5506:dbl)
            n882 = Negate(x=w5501) -> (-x=w5498:dbl)
            n883 = Multiply(x=w5498, y="MCL Step Increment (V_int)") -> (x*y=w5500:dbl)
            n884 = Divide(x=w5506, y="MCL X Cal (nm/V)") -> (x/y=w5512:dbl)
            n885 = Multiply(x=32767.0 ("y"), y=w5512) -> (x*y=w5518:dbl)
            n886 = local read "Total Counts (ticks)"() -> (w5503:u32)
            n887 = local read "Cycles/step (AOD)"() -> (w5514:u64)
            n888 = local read "Scan steps (AOD)"() -> (w5515:u64)
            n889 = Divide(x=w5518, y=10.0) -> (x/y=w5511:dbl)
            n890 = Divide(x=w5511, y="MCL Step Increment (V_int)") -> (x/y=w5509:dbl)
            n891 = Absolute Value(x=w5509) -> (abs(x)=w5497:dbl)
            n892 = Compound Arithmetic op=MULTIPLY(w5515, w5514, w5503) -> (w5510:u64)
            n893 = local write "wait to reset values"(w5525) -> ()
            n894 = local write "MCL Scanning"(w5525) -> ()
            n895 = Divide(x=w5510, y=w5497) -> (x/y=w5507:dbl)
            "MCL Count" <- w5507
            n896 = xnode "Read/Write Control"("FPGA VI Reference In"=w5524, "error in"=w5523, "Scan steps (MCL)"=w5497, "Number of scans (MCL)"=w5519, "Cycles per step (MCL)"=u64 1, "Scan freq.  increment (MCL)"=w5500, "1D or 2D Scan?"=w5520, "MCL Scan Axis"=w5520, "Cont. Scan (MCL)"=w5520, "MCL count"=w5507) -> ("FPGA VI Reference Out"=w5522:T15, "error out"=w5521:errorcluster)
            n897 = xnode "Read/Write Control"("FPGA VI Reference In"=w5522, "error in"=w5521, "AI to FIFO"=w5525, "APD to FIFO"=w5525, "Start scan"=w5525, "Start scan (MCL)"=w5525) -> ("FPGA VI Reference Out"=w5527:T15, "error out"=w5526:errorcluster)
          }
        }
        "Raster Scanning..." <- TRUE ("Scanning...")
      }
    }
    n898 = Compound Arithmetic op=OR("Start MCL Scan", "Confocal Image", "Confocal Linescan") -> (w3885:bool)
    n899 = And(x="Save Data (MCL)", y=w3885) -> (x .and. y?=w3935:bool)
    n900 = case "Start MCL raster scan" shown="True" w3885 {
      tunnel: w3938 -> [w4589 w4604]
      tunnel: w3937 -> [w4588 w4603]
      tunnel: [w4589 w4599] -> w3822
      tunnel: [w4588 w4598] -> w3821
      tunnel: [FALSE w4597] -> w3921
      tunnel: "Start MCL Scan" -> [_ w4592]
      tunnel: "Confocal Image" -> [_ w4591]
      tunnel: "Confocal Linescan" -> [_ _]
      frame #0 {
      }
      frame #1 {
        w4597 = TRUE
        n901 = case shown="True" "Restart DMA? (MCL)" {
          tunnel: [w4841 w4844] -> w4602
          tunnel: [w4840 w4843] -> w4601
          tunnel: w4604 -> [w4841 w4849]
          tunnel: w4603 -> [w4840 w4848]
          frame #0 {
          }
          frame #1 {
            w4845 = FALSE ("AI to FIFO")
            n902 = xnode "Read/Write Control"("FPGA VI Reference In"=w4849, "error in"=w4848, "AI to FIFO"=w4845, "APD to FIFO"=w4845) -> ("FPGA VI Reference Out"=w4847:T15, "error out"=w4846:errorcluster)
            n903 = xnode "Invoke Method"("FPGA VI Reference In"=w4847, "error in"=w4846) -> ("FPGA VI Reference Out"=w4851:T15, "error out"=w4850:errorcluster)
            n904 = xnode "Invoke Method"("FPGA VI Reference In"=w4851, "error in"=w4850) -> ("FPGA VI Reference Out"=w4844:T15, "error out"=w4843:errorcluster)
            n905 = local write "Overflow (data lost)"(FALSE ("Overflow (data lost)")) -> ()
          }
        }
        n906 = case shown="False" w4592 {
          selector: w4592 -> [_ w4608]
          tunnel: w4591 -> [w4607 _]
          tunnel: [w4607 w4608] -> w4590
          frame #0 {
            n907 = property on="2D or 1D Scan" class="Bool (strict)"("Val(Sgnl)"=w4607) -> ()  [unwired: 2 in, 2 out]
            n908 = property on="Confocal Image" class="Bool (strict)"("Value"=FALSE ("Start Confocal Map")) -> ()  [unwired: 2 in, 2 out]
          }
          frame #1 {
          }
        }
        n909 = local write "MCL Scanning"(w4597) -> ()
        n910 = local read "AO1"() -> (w4594:dbl)
        n911 = local read "AO2"() -> (w4593:dbl)
        n912 = case shown="True" "Center Scan" {
          tunnel: w4602 -> [w4615 w4724]
          tunnel: w4601 -> [w4614 w4723]
          tunnel: [w4613 w4722] -> w4599
          tunnel: [w4612 w4721] -> w4598
          tunnel: [w4610 w4708] -> w4596
          tunnel: [w4609 w4707] -> w4595
          tunnel: w4594 -> [w4610 w4713]
          tunnel: w4593 -> [w4609 w4716]
          tunnel: w4590 -> [_ _]
          frame #0 {
            w4611 = TRUE ("AI to FIFO")
            n913 = xnode "Read/Write Control"("FPGA VI Reference In"=w4615, "error in"=w4614, "AI to FIFO"=w4611, "APD to FIFO"=w4611, "Start scan (MCL)"=w4611) -> ("FPGA VI Reference Out"=w4613:T15, "error out"=w4612:errorcluster)
          }
          frame #1 {
            w4720 = TRUE ("AI to FIFO")
            n914 = local read "Scan steps (MCL)"() -> (w4699:u64)
            n915 = local read "Scan lines (y)"() -> (w4695:u64)
            n916 = local read "Fast Scan Dir"() -> (w4706:bool)
            n917 = local read "Actual MCL Inc (V)"() -> (w4696:dbl)
            n918 = Decrement(x=w4695) -> (x-1=w4694:u64)
            n919 = Decrement(x=w4699) -> (x-1=w4698:u64)
            n920 = Multiply(x=w4696, y=w4694) -> (x*y=w4693:dbl)
            n921 = Divide(x=w4693, y=2.0) -> (x/y=w4703:dbl)
            n922 = Multiply(x=w4696, y=w4698) -> (x*y=w4697:dbl)
            n923 = Divide(x=w4697, y=2.0) -> (x/y=w4702:dbl)
            n924 = Select(t=w4702, s=w4706, f=w4703) -> (s? t:f=w4701:dbl)
            n925 = Select(t=w4703, s=w4706, f=w4702) -> (s? t:f=w4705:dbl)
            n926 = Subtract(x=w4713, y=w4705) -> (x-y=w4704:dbl)
            n927 = Subtract(x=w4716, y=w4701) -> (x-y=w4700:dbl)
            n928 = local read "2D or 1D Scan"() -> (w4718:bool)
            n929 = Not(x=w4706) -> (.not. x?=w4712:bool)
            n930 = Not(x=w4718) -> (.not. x?=w4714:bool)
            n931 = And(x=w4706, y=w4714) -> (x .and. y?=w4715:bool)
            n932 = And(x=w4714, y=w4712) -> (x .and. y?=w4717:bool)
            n933 = Select(t=w4716, s=w4717, f=w4700) -> (s? t:f=w4707:dbl)
            n934 = Select(t=w4713, s=w4715, f=w4704) -> (s? t:f=w4708:dbl)
            n935 = call "Volt to I16.vi"("Voltage In"=w4708) -> ("I16 Voltage Out"=w4711:i16)
            n936 = call "Volt to I16.vi"("Voltage In"=w4707) -> ("I16 Voltage Out"=w4710:i16)
            n937 = xnode "Read/Write Control"("FPGA VI Reference In"=w4724, "error in"=w4723, "AI to FIFO"=w4720, "APD to FIFO"=w4720, "Start scan (MCL)"=w4720, "AO1"=w4711, "AO2"=w4710) -> ("FPGA VI Reference Out"=w4722:T15, "error out"=w4721:errorcluster)
          }
        }
        "Initial Y" <- w4596
        "Initial X" <- w4595
        "wait to reset values" <- w4597
      }
    }
    n938 = local read "APD Elements/DMA read"() -> (w3790:u32)
    n939 = local read "Elements/DMA read"() -> (w3845:u32)
    n940 = xnode "Get APD Data"("FPGA VI Reference In"=w3822, "error in"=w3821, "Number of Elements"=w3790, "Timeout (ms)"=-1) -> ("Data"=w3789:u32[], "Elements Remaining"=→"APD FIFO Elements Remaining":u32)  [unwired: 2 out]
    n941 = xnode "Get Trap Data"("FPGA VI Reference In"=w3822, "error in"=w3821, "Number of Elements"=w3845, "Timeout (ms)"=-1 ("Timeout")) -> ("FPGA VI Reference Out"=w3824:T15, "error out"=w3823:errorcluster, "Data"=w3961:u32[], "Elements Remaining"=w3991:u32)
    "FIFO El. Rem." <- w3991
    n942 = local read "FIFO Depth"() -> (w3993:u32)
    n943 = Subtract(x=w3993, y=w3845) -> (x-y=w3992:u32)
    n944 = Divide(x=w3991, y=w3992) -> (x/y=w3990:dbl)
    "Buffer Status" <- w3990
    n945 = Equal?(x=w3990, y=1.0) -> (x = y?=w3988:bool)
    n946 = case "Alert buffer overflow" shown="True" w3988 {
      frame #0 {
      }
      frame #1 {
        n947 = call <vilib>:"Beep.vi"() -> ()  [unwired: 3 in, 9 out]
        "Overflow (data lost)" <- TRUE ("Overflow (data lost)")
      }
    }
    n948 = local read "FPGA Averaging"() -> (w3844:bool)
    n949 = case "Special unpacking case if no averaging done by FPGA" shown="False" w3844 {
      tunnel: w3961 -> [w5001 w5027]
      tunnel: [w4972 w5002] -> w3960
      frame #0 {
        n950 = Decimate 1D Array(w5001) -> (w5000:u32[], w4999:u32[], w4998:u32[], w4997:u32[])
        n951 = Split Number(x=w5000) -> (hi(x)=w4996:u16[], lo(x)=w4995:u16[])
        n952 = Split Number(x=w4999) -> (hi(x)=w4994:u16[], lo(x)=w4993:u16[])
        n953 = Split Number(x=w4998) -> (hi(x)=w4992:u16[], lo(x)=w4991:u16[])
        n954 = Split Number(x=w4997) -> (hi(x)=w4990:u16[], lo(x)=w4989:u16[])
        n955 = To Word Integer(number=w4996) -> (16bit integer=w4988:i16[])
        n956 = To Word Integer(number=w4995) -> (16bit integer=w4987:i16[])
        n957 = To Word Integer(number=w4994) -> (16bit integer=w4986:i16[])
        n958 = To Word Integer(number=w4993) -> (16bit integer=w4985:i16[])
        n959 = To Word Integer(number=w4992) -> (16bit integer=w4984:i16[])
        n960 = To Word Integer(number=w4991) -> (16bit integer=w4983:i16[])
        n961 = To Word Integer(number=w4990) -> (16bit integer=w4982:i16[])
        n962 = To Word Integer(number=w4989) -> (16bit integer=w4981:i16[])
        n963 = To Double Precision Float(number=w4988) -> (double precision float=w4980:dbl[])
        n964 = To Double Precision Float(number=w4987) -> (double precision float=w4979:dbl[])
        n965 = To Double Precision Float(number=w4986) -> (double precision float=w4978:dbl[])
        n966 = To Double Precision Float(number=w4985) -> (double precision float=w4977:dbl[])
        n967 = To Double Precision Float(number=w4984) -> (double precision float=w4976:dbl[])
        n968 = To Double Precision Float(number=w4983) -> (double precision float=w4975:dbl[])
        n969 = To Double Precision Float(number=w4982) -> (double precision float=w4974:dbl[])
        n970 = To Double Precision Float(number=w4981) -> (double precision float=w4973:dbl[])
        n971 = Interleave 1D Arrays(w4980, w4979, w4978, w4977, w4976, w4975, w4974, w4973) -> (w4972:dbl[])
      }
      frame #1 {
        n972 = Decimate 1D Array(w5027) -> (w5018:u32[], w5016:u32[], w5014:u32[], w5012:u32[], w5010:u32[], w5008:u32[], w5006:u32[], w5004:u32[])
        n973 = To Long Integer(number=w5018) -> (32bit integer=w5026:i32[])
        n974 = To Long Integer(number=w5016) -> (32bit integer=w5025:i32[])
        n975 = To Long Integer(number=w5014) -> (32bit integer=w5024:i32[])
        n976 = To Long Integer(number=w5012) -> (32bit integer=w5023:i32[])
        n977 = To Long Integer(number=w5010) -> (32bit integer=w5022:i32[])
        n978 = To Long Integer(number=w5008) -> (32bit integer=w5021:i32[])
        n979 = To Long Integer(number=w5006) -> (32bit integer=w5020:i32[])
        n980 = To Long Integer(number=w5004) -> (32bit integer=w5019:i32[])
        n981 = To Double Precision Float(number=w5026) -> (double precision float=w5017:dbl[])
        n982 = To Double Precision Float(number=w5025) -> (double precision float=w5015:dbl[])
        n983 = To Double Precision Float(number=w5024) -> (double precision float=w5013:dbl[])
        n984 = To Double Precision Float(number=w5023) -> (double precision float=w5011:dbl[])
        n985 = To Double Precision Float(number=w5022) -> (double precision float=w5009:dbl[])
        n986 = To Double Precision Float(number=w5021) -> (double precision float=w5007:dbl[])
        n987 = To Double Precision Float(number=w5020) -> (double precision float=w5005:dbl[])
        n988 = To Double Precision Float(number=w5019) -> (double precision float=w5003:dbl[])
        n989 = Interleave 1D Arrays(w5017, w5015, w5013, w5011, w5009, w5007, w5005, w5003) -> (w5002:dbl[])
      }
    }
    n990 = local read "FPGA Ave."() -> (w3843:dbl)
    n991 = feedback #4(i16 -1 ("Trap Sets")) -> (w3841:i16)
    n992 = feedback #5("" ("Detector Type")) -> (w3838:string)
    n993 = Not Equal?(x=w3838, y="Detector Type") -> (x != y?=w3836:bool)
    n994 = local read "Trap Sets"() -> (w3840:i16)
    n995 = Not Equal?(x=w3841, y=w3840) -> (x != y?=w3835:bool)
    n996 = Or(x=w3836, y=w3835) -> (x .or. y?=w3834:bool)
    n997 = Divide(x=w3960, y=w3843) -> (x/y=w3968:dbl[])
    n998 = case "Deinterlace trap data, average down PSD" shown="2" w3840 {
      tunnel: w3968 -> [w5046 w5111]
      tunnel: [w5043 w5108] -> w3828
      tunnel: [w5046 w5110] -> w3967
      tunnel: "Detector Type" -> [w5045 w5106]
      tunnel: [w5044 w5109] -> w3826
      tunnel: [w5042 w5107] -> w3959
      frame #0 {
        n999 = Divide(x=w5046, y=3276.7) -> (x/y=w5047:dbl[])
        n1000 = Decimate 1D Array(w5047) -> (w5056:dbl[], w5055:dbl[], w5054:dbl[], w5053:dbl[], w5052:dbl[], w5051:dbl[], w5050:dbl[], w5049:dbl[])
        n1001 = case shown="\"IR-QPD + PSD + FB-QPD position\"" w5045 {
          tunnel: w5056 -> [w5080 w5105]
          tunnel: w5055 -> [w5079 w5104]
          tunnel: w5054 -> [w5064 w5082]
          tunnel: w5053 -> [w5065 w5092]
          tunnel: w5052 -> [w5078 w5103]
          tunnel: w5051 -> [w5077 w5102]
          tunnel: w5050 -> [w5061 w5083]
          tunnel: w5049 -> [w5060 w5081]
          tunnel: [w5059 w5089] -> w5044
          tunnel: [w5058 w5088] -> w5043
          tunnel: [w5057 w5087] -> w5042
          frame #0 {
            w5057 = 0  # Channel pattern
            n1002 = Divide(x=w5080, y=w5065) -> (x/y=w5067:dbl[])
            n1003 = Divide(x=w5079, y=w5065) -> (x/y=w5066:dbl[])
            n1004 = Divide(x=w5078, y=w5061) -> (x/y=w5063:dbl[])
            n1005 = Divide(x=w5077, y=w5060) -> (x/y=w5062:dbl[])
            n1006 = Build Array(w5067, w5066, w5065, w5064, w5063, w5062, w5061, w5060) -> (w5058:dbl[][])
            n1007 = Bundle("T1 Y", "T1 X", "T1 Sum", "FB Sum", "PSD Y", "PSD X", "PSD Y Sum", "PSD X Sum") -> (w5076:T36)  [unwired: 1 out]
            n1008 = Cluster To Array(cluster=w5076) -> (array=w5059:string[])
          }
          frame #1 {
            w5087 = 3  # Channel pattern
            n1009 = Negate(x=w5083) -> (-x=w5084:dbl[])
            n1010 = Divide(x=w5105, y=w5092) -> (x/y=w5094:dbl[])
            n1011 = Divide(x=w5104, y=w5092) -> (x/y=w5093:dbl[])
            n1012 = Divide(x=w5103, y=w5083) -> (x/y=w5091:dbl[])
            n1013 = Divide(x=w5102, y=w5084) -> (x/y=w5090:dbl[])
            n1014 = Build Array(w5094, w5093, w5092, w5081, w5082, w5091, w5090, w5083) -> (w5088:dbl[][])
            n1015 = Bundle("T1 Y", "T1 X", "T1 Sum", "FB X", "FB Sum", "PSD Y", "PSD X", "PSD Y Sum") -> (w5101:T36)  [unwired: 1 out]
            n1016 = Cluster To Array(cluster=w5101) -> (array=w5089:string[])
          }
        }
      }
      frame #1 {
        n1017 = case shown="\"IR-QPD + PSD + FB-QPD X position\"" w5106 {
          tunnel: w5111 -> [w5172 w5239 w5309]
          tunnel: [w5152 w5224 w5296] -> w5110
          tunnel: [w5138 w5215 w5287] -> w5109
          tunnel: [w5137 w5175 w5254] -> w5108
          tunnel: [w5131 w5213 w5285] -> w5107
          frame #0 {
            w5131 = 1  # Channel pattern
            # "time average x2 the 4th signal and the 4 psd signals (detection laser)"
            # "deinterlace 3 signals from qpd"
            n1018 = Decimate 1D Array(w5172) -> (w5171:dbl[], w5170:dbl[], w5136:dbl[], w5169:dbl[], w5159:dbl[], w5157:dbl[], w5156:dbl[], w5154:dbl[])
            n1019 = Decimate 1D Array(w5136) -> (w5135:dbl[], w5134:dbl[])
            n1020 = Decimate 1D Array(w5171) -> (w5168:dbl[], w5140:dbl[])
            n1021 = Decimate 1D Array(w5170) -> (w5167:dbl[], w5165:dbl[])
            n1022 = Decimate 1D Array(w5169) -> (w5166:dbl[], w5164:dbl[])
            n1023 = call "downsample 1D array - double.vi"("Ave N"=2.0, "Array In"=w5159) -> ("Array Out"=w5158:dbl[])  [unwired: 1 out]
            n1024 = call "downsample 1D array - double.vi"("Ave N"=2.0, "Array In"=w5157) -> ("Array Out"=w5139:dbl[])  [unwired: 1 out]
            n1025 = call "downsample 1D array - double.vi"("Ave N"=2.0, "Array In"=w5156) -> ("Array Out"=w5155:dbl[])  [unwired: 1 out]
            n1026 = call "downsample 1D array - double.vi"("Ave N"=2.0, "Array In"=w5154) -> ("Array Out"=w5153:dbl[])  [unwired: 1 out]
            n1027 = Interleave 1D Arrays(w5168, w5167, w5166, w5140, w5165, w5164, w5135, w5134, w5158, w5139, w5155, w5153) -> (w5152:dbl[])
            n1028 = Divide(x=w5152, y=3276.7) -> (x/y=w5151:dbl[])
            n1029 = Decimate 1D Array(w5151) -> (w5150:dbl[], w5149:dbl[], w5148:dbl[], w5147:dbl[], w5146:dbl[], w5145:dbl[], w5133:dbl[], w5132:dbl[], w5144:dbl[], w5143:dbl[], w5142:dbl[], w5141:dbl[])
            n1030 = Divide(x=w5150, y=w5148) -> (x/y=w5118:dbl[])
            n1031 = Divide(x=w5149, y=w5148) -> (x/y=w5117:dbl[])
            n1032 = Divide(x=w5147, y=w5145) -> (x/y=w5116:dbl[])
            n1033 = Divide(x=w5146, y=w5145) -> (x/y=w5115:dbl[])
            n1034 = Divide(x=w5144, y=w5142) -> (x/y=w5114:dbl[])
            n1035 = Divide(x=w5143, y=w5141) -> (x/y=w5113:dbl[])
            n1036 = Build Array(w5118, w5117, w5148, w5116, w5115, w5145, w5133, w5132, w5114, w5113, w5142, w5141) -> (w5137:dbl[][])
            n1037 = Bundle("T1 Y", "T1 X", "T1 Sum", "T2 Y", "T2 X", "T2 Sum", "T1 FB Sum", "T2 FB Sum", "PSD Y", "PSD X", "PSD Y Sum", "PSD X Sum") -> (w5119:T37)  [unwired: 1 out]
            n1038 = Cluster To Array(cluster=w5119) -> (array=w5138:string[])
          }
          frame #1 {
            w5213 = 2  # Channel pattern
            # "time average x2 the 3 psd signals (detection laser)"
            # "deinterlace 3 signals from qpds"
            n1039 = Decimate 1D Array(w5239) -> (w5238:dbl[], w5237:dbl[], w5214:dbl[], w5236:dbl[], w5227:dbl[], w5226:dbl[], w5225:dbl[], w5201:dbl[])
            n1040 = Decimate 1D Array(w5214) -> (w5196:dbl[], w5194:dbl[])
            n1041 = Decimate 1D Array(w5238) -> (w5235:dbl[], w5216:dbl[])
            n1042 = Decimate 1D Array(w5237) -> (w5234:dbl[], w5232:dbl[])
            n1043 = Decimate 1D Array(w5236) -> (w5233:dbl[], w5231:dbl[])
            n1044 = Decimate 1D Array(w5201) -> (w5197:dbl[], w5195:dbl[])
            n1045 = call "downsample 1D array - double.vi"("Ave N"=2.0, "Array In"=w5227) -> ("Array Out"=w5200:dbl[])  [unwired: 1 out]
            n1046 = call "downsample 1D array - double.vi"("Ave N"=2.0, "Array In"=w5226) -> ("Array Out"=w5199:dbl[])  [unwired: 1 out]
            n1047 = call "downsample 1D array - double.vi"("Ave N"=2.0, "Array In"=w5225) -> ("Array Out"=w5198:dbl[])  [unwired: 1 out]
            n1048 = Interleave 1D Arrays(w5235, w5234, w5233, w5216, w5232, w5231, w5197, w5196, w5195, w5194, w5200, w5199, w5198) -> (w5224:dbl[])
            n1049 = Divide(x=w5224, y=3276.7) -> (x/y=w5223:dbl[])
            n1050 = Decimate 1D Array(w5223) -> (w5222:dbl[], w5221:dbl[], w5220:dbl[], w5219:dbl[], w5218:dbl[], w5217:dbl[], w5186:dbl[], w5184:dbl[], w5183:dbl[], w5181:dbl[], w5180:dbl[], w5179:dbl[], w5176:dbl[])
            n1051 = Negate(x=w5176) -> (-x=w5174:dbl[])
            n1052 = Divide(x=w5180, y=w5176) -> (x/y=w5178:dbl[])
            n1053 = Divide(x=w5179, y=w5174) -> (x/y=w5177:dbl[])
            n1054 = Divide(x=w5222, y=w5220) -> (x/y=w5205:dbl[])
            n1055 = Divide(x=w5221, y=w5220) -> (x/y=w5204:dbl[])
            n1056 = Divide(x=w5219, y=w5217) -> (x/y=w5203:dbl[])
            n1057 = Divide(x=w5218, y=w5217) -> (x/y=w5202:dbl[])
            n1058 = Divide(x=w5186, y=w5184) -> (x/y=w5185:dbl[])
            n1059 = Divide(x=w5183, y=w5181) -> (x/y=w5182:dbl[])
            n1060 = Build Array(w5205, w5204, w5220, w5203, w5202, w5217, w5185, w5184, w5182, w5181, w5178, w5177, w5176) -> (w5175:dbl[][])
            n1061 = Bundle("T1 Y", "T1 X", "T1 Sum", "T2 Y", "T2 X", "T2 Sum", "T1 FB X", "T1 FB Sum", "T2 FB X", "T2 FB Sum", "PSD Y", "PSD X", "PSD Y Sum") -> (w5206:T38)  [unwired: 1 out]
            n1062 = Cluster To Array(cluster=w5206) -> (array=w5215:string[])
          }
          frame #2 {
            w5285 = 4  # Channel pattern
            # "time average x2 the 3 psd signals (detection laser)"
            # "deinterlace 3 signals from qpds"
            n1063 = Decimate 1D Array(w5309) -> (w5308:dbl[], w5307:dbl[], w5286:dbl[], w5306:dbl[], w5252:dbl[], w5298:dbl[], w5297:dbl[], w5274:dbl[])
            n1064 = Decimate 1D Array "Feedback Sum"(w5286) -> (w5270:dbl[], w5268:dbl[])
            n1065 = Decimate 1D Array "QPD Y"(w5308) -> (w5305:dbl[], w5288:dbl[])
            n1066 = Decimate 1D Array "QPD X"(w5307) -> (w5304:dbl[], w5302:dbl[])
            n1067 = Decimate 1D Array "Feedback Y"(w5252) -> (w5251:dbl[], w5250:dbl[])
            n1068 = Decimate 1D Array "QPD Sum"(w5306) -> (w5303:dbl[], w5301:dbl[])
            n1069 = Decimate 1D Array "Feedback X"(w5274) -> (w5271:dbl[], w5269:dbl[])
            n1070 = call "downsample 1D array - double.vi"("Ave N"=2.0, "Array In"=w5298) -> ("Array Out"=w5273:dbl[])  [unwired: 1 out]
            n1071 = call "downsample 1D array - double.vi"("Ave N"=2.0, "Array In"=w5297) -> ("Array Out"=w5272:dbl[])  [unwired: 1 out]
            n1072 = Interleave 1D Arrays(w5305, w5304, w5303, w5288, w5302, w5301, w5251, w5271, w5270, w5250, w5269, w5268, w5273, w5272) -> (w5296:dbl[])
            n1073 = Divide(x=w5296, y=3276.7) -> (x/y=w5295:dbl[])
            n1074 = Decimate 1D Array(w5295) -> (w5294:dbl[], w5293:dbl[], w5292:dbl[], w5291:dbl[], w5290:dbl[], w5289:dbl[], w5247:dbl[], w5261:dbl[], w5245:dbl[], w5246:dbl[], w5259:dbl[], w5243:dbl[], w5257:dbl[], w5255:dbl[])
            n1075 = Negate(x=w5255) -> (-x=w5253:dbl[])
            n1076 = Divide(x=w5257, y=w5253) -> (x/y=w5256:dbl[])
            n1077 = Divide(x=w5246, y=w5243) -> (x/y=w5242:dbl[])
            n1078 = Divide(x=w5247, y=w5245) -> (x/y=w5244:dbl[])
            n1079 = Divide(x=w5294, y=w5292) -> (x/y=w5278:dbl[])
            n1080 = Divide(x=w5293, y=w5292) -> (x/y=w5277:dbl[])
            n1081 = Divide(x=w5291, y=w5289) -> (x/y=w5276:dbl[])
            n1082 = Divide(x=w5290, y=w5289) -> (x/y=w5275:dbl[])
            n1083 = Divide(x=w5261, y=w5245) -> (x/y=w5260:dbl[])
            n1084 = Divide(x=w5259, y=w5243) -> (x/y=w5258:dbl[])
            n1085 = Build Array(w5278, w5277, w5292, w5276, w5275, w5289, w5244, w5260, w5245, w5242, w5258, w5243, w5256, w5255) -> (w5254:dbl[][])
            n1086 = Bundle("T1 Y", "T1 X", "T1 Sum", "T2 Y", "T2 X", "T2 Sum", "T1 FB Y", "T1 FB X", "T1 FB Sum", "T2 FB Y", "T2 FB X", "T2 FB Sum", "PSD X", "PSD Y Sum") -> (w5241:T39)  [unwired: 1 out]
            n1087 = Cluster To Array(cluster=w5241) -> (array=w5287:string[])
          }
        }
      }
    }
    n1088 = case "Update these things only if detector type or number of traps changes" shown="True" w3834 {
      tunnel: w3826 -> [_ w4114]
      frame #0 {
      }
      frame #1 {
        n1089 = property on="High Res. Display" class="Ring (strict)"("Strings []"=w4114) -> ()  [unwired: 2 in, 2 out]
        n1090 = Build Array (concatenate)(w4114, "none") -> (w4107:string[])
        n1091 = property on="FFT 1 Choice 1" class="Ring (strict)"("Strings []"=w4107) -> ()  [unwired: 2 in, 2 out]
        n1092 = property on="FFT 1 Choice 2" class="Ring (strict)"("Strings []"=w4107) -> ()  [unwired: 2 in, 2 out]
        n1093 = property on="FFT 2 Choice 1" class="Ring (strict)"("Strings []"=w4107) -> ()  [unwired: 2 in, 2 out]
        n1094 = property on="FFT 2 Choice 2" class="Ring (strict)"("Strings []"=w4107) -> ()  [unwired: 2 in, 2 out]
        n1095 = Bundle("APD 1", "APD 2") -> (w4110:cluster{string, string})  [unwired: 1 out]
        n1096 = Cluster To Array(cluster=w4110) -> (array=w4108:string[])
        n1097 = Build Array (concatenate)(w4108, w4107) -> (w4112:string[])
        n1098 = Array Size(array=w4112) -> (size(s)=w4113:i32)
        n1099 = property on="Signals to Plot" class="LstBox (strict)"("Item Names"=w4112) -> ()  [unwired: 2 in, 2 out]
        n1100 = property on="Signals to Plot" class="LstBox (strict)"("Number of Rows"=w4113) -> ()  [unwired: 2 in, 2 out]
        n1101 = property on="All Signals" class="WFChart (strict)"("LegNumRows"=w4113) -> ()  [unwired: 2 in, 2 out]
      }
    }
    n1102 = local read "Data points/scans (MCL)"() -> (w3930:dbl)
    n1103 = Increment(x=w3930) -> (x+1=w3931:dbl)
    n1104 = feedback #6(w3931) -> (w3934:dbl)
    n1105 = Select(t=0, s=w3921, f=w3934) -> (s? t:f=w3927:dbl)
    n1106 = To Word Integer(number=w3967) -> (16bit integer=w3994:i16[])
    n1107 = Decimate 1D Array(w3789) -> (w3820:u32[], w3957:u32[])
    n1108 = To Double Precision Float(number=w3820) -> (double precision float=w3819:dbl[])
    n1109 = Array Size(array=w3819) -> (size(s)=w3933:i32)
    n1110 = Add(x=w3933, y=w3927) -> (x+y=w3928:dbl)
    n1111 = Greater?(x=w3928, y=w3930) -> (0:w3929:bool)
    n1112 = local read "DMA Update Period (s)"() -> (w3847:dbl)
    n1113 = Select(t=w3927, s=w3929, f=w3928) -> (s? t:f=w3926:dbl)
    n1114 = Build Array(w3820, w3957) -> (w3918:u32[][])
    n1115 = local read "MCL Scanning"() -> (w3924:bool)
    n1116 = local read "Data Period (s)"() -> (w3805:dbl)
    n1117 = To Double Precision Float(number=w3918) -> (double precision float=w3919:dbl[][])
    n1118 = Not(x=w3929) -> (.not. x?=w3923:bool)
    n1119 = local read "APD Integration Time (s)"() -> (w3846:dbl)
    n1120 = And(x=w3923, y=w3924) -> (x .and. y?=w3925:bool)
    n1121 = feedback #7(0.0) -> (w3954:dbl)
    n1122 = Add(x=w3847, y=w3954) -> (x+y=w3963:dbl)
    n1123 = Or(x=w3925, y=w3921) -> (x .or. y?=w3922:bool)
    n1124 = Multiply(x=w3805, y="Trap Disp. Downsample") -> (x*y=w3803:dbl)
    "Display Period (s)" <- w3803
    n1125 = Equal?(x="Tab Control 6", y=T29."High Res Display") -> (x = y?=w3831:bool)
    n1126 = for {
      tunnel: [w5041] -> w3953 mode=indexing
      tunnel: w3954 -> [w5040]
      tunnel: "Trap Disp. Downsample" -> [w5037]
      tunnel: w3828 -> [w5035] mode=indexing
      tunnel: w3805 -> [w5034]
      tunnel: w3826 -> [w5033] mode=indexing
      tunnel: w3827 -> [w5032]
      tunnel: [w5031] -> w3776 mode=indexing
      tunnel: w3803 -> [w5030]
      n1127 = Bundle By Name("Y"=w5035, "dt"=w5034) -> (w5036:waveform(dbl))  [unwired: 1 out]
      n1128 = Set Waveform Attribute(5:w5033, 6:w5032, 7:w5036) -> (3:w5031:waveform(dbl))  [unwired: 1 in, 2 out]
      n1129 = call "downsample 1D array - double.vi"("Ave N"=w5037, "Array In"=w5035) -> ("Array Out"=w5038:dbl[])  [unwired: 1 out]
      n1130 = To Time Stamp(1:w5040) -> (0:w5039:timestamp)
      n1131 = Bundle By Name(cluster=w5031, "t0"=w5039, "Y"=w5038, "dt"=w5030) -> (w5041:waveform(dbl))
    }
    n1132 = case "For plotting results of scanning MCL" shown="True" w3922 {
      tunnel: w3921 -> [_ w4564]
      tunnel: w3819 -> [_ w4577]
      tunnel: w3930 -> [_ _]
      tunnel: w3776 -> [_ w4548]
      tunnel: w3777 -> [_ w4480]
      tunnel: w3775 -> [_ w4478]
      tunnel: w3774 -> [_ w4477]
      frame #0 {
      }
      frame #1 {
        w4485 = u32 0 items=["Horizontal", "Vertical", "Central", "1st Diagonal", "2nd Diagonal"] ("Type of Symmetry")
        w4488 = u32 0 items=["Horizontal", "Vertical", "Central", "1st Diagonal", "2nd Diagonal"] ("Type of Symmetry")
        w4518 = u32 0 items=["Horizontal", "Vertical", "Central", "1st Diagonal", "2nd Diagonal"] ("Type of Symmetry")
        n1133 = Index Array(array=w4548, index=10) -> (element=w4554:waveform(dbl))
        n1134 = Index Array(array=w4548, index=11) -> (element=w4551:waveform(dbl))
        n1135 = Index Array(array=w4548, index="Channel") -> (element=w4550:waveform(dbl))
        n1136 = local read "Cycles/step (MCL)"() -> (w4502:u64)
        n1137 = Unbundle By Name(w4554) -> ("Y"=w4504:dbl[])
        n1138 = Unbundle By Name(w4551) -> ("Y"=w4506:dbl[])
        n1139 = Unbundle By Name(w4550) -> ("Y"=w4511:dbl[])
        n1140 = call "downsample 1D array - double.vi"("Ave N"=w4502, "Array In"=w4504) -> ("Array Out"=w4503:dbl[])  [unwired: 1 out]
        n1141 = call "downsample 1D array - double.vi"("Ave N"=w4502, "Array In"=w4506) -> ("Array Out"=w4505:dbl[])  [unwired: 1 out]
        n1142 = call "downsample 1D array - double.vi"("Ave N"=w4502, "Array In"=w4511) -> ("Array Out"=w4510:dbl[])  [unwired: 1 out]
        n1143 = feedback #8(w4577) -> (w4578:dbl[])
        n1144 = Build Array (concatenate)(w4578, w4577) -> (w4556:dbl[])
        n1145 = Select(t=w4577, s=w4564, f=w4556) -> (s? t:f=w4561:dbl[])
        n1146 = feedback #9(w4503) -> (w4565:dbl[])
        n1147 = Build Array (concatenate)(w4565, w4503) -> (w4553:dbl[])
        n1148 = feedback #10(w4510) -> (w4575:dbl[])
        n1149 = Build Array (concatenate)(w4575, w4510) -> (w4574:dbl[])
        n1150 = feedback #11(w4505) -> (w4567:dbl[])
        n1151 = Build Array (concatenate)(w4567, w4505) -> (w4568:dbl[])
        n1152 = Select(t=w4503, s=w4564, f=w4553) -> (s? t:f=w4507:dbl[])
        n1153 = Select(t=w4510, s=w4564, f=w4574) -> (s? t:f=w4509:dbl[])
        n1154 = Select(t=w4505, s=w4564, f=w4568) -> (s? t:f=w4508:dbl[])
        n1155 = local read "N APD Samp/step"() -> (w4560:dbl)
        n1156 = local read "Scan steps (MCL)"() -> (w4515:u64)
        n1157 = local read "Scan lines (y)"() -> (w4547:u64)
        n1158 = call "integrate 1D array interval - double.vi"("Ave N"=w4560, "Array In"=w4561) -> ("Array Out"=w4559:dbl[])  [unwired: 1 out]
        n1159 = Array Size(array=w4559) -> (size(s)=w4563:i32)
        n1160 = Multiply(x=w4515, y=u64 2) -> (x*y=w4562:u64)
        n1161 = Multiply(x=w4547, y=w4562) -> (x*y=w4572:u64)
        n1162 = Subtract(x=w4572, y=w4563) -> (x-y=w4501:u64)
        n1163 = call <vilib>:"Mean.vi"("X"=w4559) -> ("mean"=w4498:dbl)  [unwired: 1 out]
        n1164 = call <vilib>:"Mean.vi"("X"=w4507) -> ("mean"=w4491:dbl)  [unwired: 1 out]
        n1165 = call <vilib>:"Mean.vi"("X"=w4509) -> ("mean"=w4496:dbl)  [unwired: 1 out]
        n1166 = call <vilib>:"Mean.vi"("X"=w4508) -> ("mean"=w4494:dbl)  [unwired: 1 out]
        n1167 = Initialize Array(1.0 ("element"), w4501) -> (w4492:dbl[])
        n1168 = Multiply(x=w4492, y=w4498) -> (x*y=w4499:dbl[])
        n1169 = Multiply(x=w4492, y=w4494) -> (x*y=w4495:dbl[])
        n1170 = Multiply(x=w4492, y=w4496) -> (x*y=w4497:dbl[])
        n1171 = Multiply(x=w4492, y=w4491) -> (x*y=w4493:dbl[])
        n1172 = Build Array (concatenate)(w4559, w4499) -> (w4571:dbl[])
        n1173 = Build Array (concatenate)(w4507, w4493) -> (w4566:dbl[])
        n1174 = Build Array (concatenate)(w4509, w4497) -> (w4570:dbl[])
        n1175 = Build Array (concatenate)(w4508, w4495) -> (w4569:dbl[])
        n1176 = Reshape Array(w4571, w4547, w4562) -> (w4545:dbl[][])
        n1177 = Reshape Array(w4566, w4547, w4562) -> (w4528:dbl[][])
        n1178 = Reshape Array(w4570, w4547, w4562) -> (w4520:dbl[][])
        n1179 = Reshape Array(w4569, w4547, w4562) -> (w4535:dbl[][])
        n1180 = Index Array(array=w4545, index (row)=0) -> (element=→"Waveform Graph":dbl[])  [unwired: 1 in]
        n1181 = Array Subset(array=w4535, index (col)=0 ("index"), length (col)=w4515) -> (w4540:dbl[][])  [unwired: 2 in]
        n1182 = Array Subset(array=w4545, index (col)=0 ("index"), length (col)=w4515) -> (w4544:dbl[][])  [unwired: 2 in]
        n1183 = Array Subset(array=w4535, index (col)=w4515) -> (w4538:dbl[][])  [unwired: 3 in]
        n1184 = Array Subset(array=w4545, index (col)=w4515) -> (w4542:dbl[][])  [unwired: 3 in]
        n1185 = Array Subset(array=w4520, index (col)=0 ("index"), length (col)=w4515) -> (w4526:dbl[][])  [unwired: 2 in]
        n1186 = Array Subset(array=w4520, index (col)=w4515) -> (w4524:dbl[][])  [unwired: 3 in]
        n1187 = Array Subset(array=w4528, index (col)=0 ("index"), length (col)=w4515) -> (w4533:dbl[][])  [unwired: 2 in]
        n1188 = Array Subset(array=w4528, index (col)=w4515) -> (w4531:dbl[][])  [unwired: 3 in]
        n1189 = for {
          tunnel: w4540 -> [w4584] mode=indexing
          tunnel: [w4583] -> w4539 mode=indexing
          n1190 = Reverse 1D Array(array=w4584) -> (reversed array=w4583:dbl[])
        }
        n1191 = for {
          tunnel: w4544 -> [w4586] mode=indexing
          tunnel: [w4585] -> w4543 mode=indexing
          n1192 = Reverse 1D Array(array=w4586) -> (reversed array=w4585:dbl[])
        }
        n1193 = for {
          tunnel: w4526 -> [w4580] mode=indexing
          tunnel: [w4579] -> w4525 mode=indexing
          n1194 = Reverse 1D Array(array=w4580) -> (reversed array=w4579:dbl[])
        }
        n1195 = for {
          tunnel: w4533 -> [w4582] mode=indexing
          tunnel: [w4581] -> w4532 mode=indexing
          n1196 = Reverse 1D Array(array=w4582) -> (reversed array=w4581:dbl[])
        }
        n1197 = Add(x=w4539, y=w4538) -> (x+y=w4537:dbl[][])
        n1198 = Add(x=w4543, y=w4542) -> (x+y=w4517:dbl[][])
        n1199 = Add(x=w4525, y=w4524) -> (x+y=w4523:dbl[][])
        n1200 = Add(x=w4532, y=w4531) -> (x+y=w4530:dbl[][])
        n1201 = Divide(x=w4523, y=2) -> (x/y=w4521:dbl[][])
        n1202 = Divide(x=w4537, y=2) -> (x/y=w4481:dbl[][])
        n1203 = To Single Precision Float(number=w4517) -> (single precision float=w4516:sgl[][])
        n1204 = Divide(x=w4530, y=2) -> (x/y=w4483:dbl[][])
        n1205 = Transpose 2D Array(2D array=w4521) -> (transposed array=→"Data map":dbl[][])
        n1206 = To Single Precision Float(number=w4481) -> (single precision float=w4487:sgl[][])
        n1207 = To Single Precision Float(number=w4483) -> (single precision float=w4484:sgl[][])
        n1208 = call "IMAQ ArrayToImage"("Image Pixels (Float)"=w4516, "Image"=w4480) -> ("Image Out"=w4519:T2)  [unwired: 8 in, 1 out]
        n1209 = call "IMAQ ArrayToImage"("Image Pixels (Float)"=w4487, "Image"=w4478) -> ("Image Out"=w4489:T2)  [unwired: 8 in, 1 out]
        n1210 = call "IMAQ Symmetry"("Type of Symmetry"=w4518, "Image Src"=w4519) -> ("Image Dst Out"=w4513:T2)  [unwired: 3 in, 1 out]
        n1211 = call "IMAQ ArrayToImage"("Image Pixels (Float)"=w4484, "Image"=w4477) -> ("Image Out"=w4486:T2)  [unwired: 8 in, 1 out]
        n1212 = call "IMAQ Symmetry"("Type of Symmetry"=w4488, "Image Src"=w4489) -> ("Image Dst Out"=→"Detection Laser X":T2)  [unwired: 3 in, 1 out]
        n1213 = call "IMAQ Symmetry"("Type of Symmetry"=w4485, "Image Src"=w4486) -> ("Image Dst Out"=→"Detection Laser Y":T2)  [unwired: 3 in, 1 out]
        n1214 = call "IMAQ Set Simple Calibration"("Calibration Axis Info"=T30 {"Origin Pixel"={"X"=0.0, "Y"=0.0}, "Angle Relative to Horizontal (deg)"=0.0, "Axis Reference"=0}, "Grid Descriptor"=T31 {"X Step"=0.3, "Y Step"=0.3, "Unit"=enum."Undefined"}, "Image"=w4513) -> ("Calibrated Image"=→"APD 1":T2)  [unwired: 7 in, 1 out]
      }
    }
    n1215 = Reciprocal(x=w3803) -> (1/x=→"Trap Disp. Freq. (Hz)":dbl)
    n1216 = case shown="True" w3831 {
      tunnel: w3776 -> [_ w4083]
      frame #0 {
      }
      frame #1 {
        n1217 = Index Array(array=w4083, index="High Res. Display") -> (element=w4084:waveform(dbl))
        n1218 = call <vilib>:"Std Deviation and Variance.vi"("X"=w4084) -> ("mean"=w4091:dbl, "standard deviation"=w4096:dbl)  [unwired: 1 in, 1 out]
        "Mean Intensity" <- w4091
        "Sigma" <- w4096
        n1219 = Subtract(x=w4084, y=w4091) -> (x-y=w4090:waveform(dbl))
        n1220 = Select(t=w4090, s="Subtract mean", f=w4084) -> (s? t:f=→"1 Channel":waveform(dbl))
        n1221 = Divide(x=w4096, y=w4091) -> (x/y=→"Sigma/Mean":dbl)
        n1222 = feedback #12(1) -> (w4085:i32)
        n1223 = Greater Or Equal?(x=w4085, y="Slow mean N ave.") -> (x >= y?=w4098:bool)
        n1224 = Increment(x=w4085) -> (x+1=w4100:i32)
        n1225 = Select(t=1, s=w4098, f=w4100) -> (s? t:f=w4087:i32)
        n1226 = feedback #13() -> (w4088:waveform(dbl))  [unwired: 1 out]
        n1227 = case shown="Default" w4085 {
          tunnel: [w4103 w4106] -> w4089
          tunnel: w4088 -> [w4105 _]
          tunnel: w4084 -> [w4104 w4106]
          frame #0 {
            n1228 = call-poly <vilib>:"Append Waveforms.vi"("waveform B"=w4104, "waveform A"=w4105) -> ("waveform out"=w4103:waveform(dbl))  [unwired: 1 in, 8 out]
          }
          frame #1 {
          }
        }
        n1229 = case shown="True" w4098 {
          tunnel: w4089 -> [_ w4102]
          frame #0 {
          }
          frame #1 {
            n1230 = call <vilib>:"Mean.vi"("X"=w4102) -> ("mean"=→"Slow mean":dbl)  [unwired: 1 out]
          }
        }
      }
    }
    n1231 = case "For computing FFTs for display" shown="True" "Compute FFT" {
      tunnel: w3776 -> [_ w5925]
      frame #0 {
      }
      frame #1 {
        n1232 = Build Array("FFT 1 Choice 1", "FFT 1 Choice 2", "FFT 2 Choice 1", "FFT 2 Choice 2") -> (w5918:u16[])
        n1233 = Array Size(array=w5925) -> (size(s)=w5924:i32)
        n1234 = feedback #14(u16[] [100, 100, 100, 100]) -> (w5919:u16[])
        n1235 = feedback #15("# Spectra to Ave.") -> (w5916:dbl)
        n1236 = Not Equal?(x="# Spectra to Ave.", y=w5916) -> (x != y?=w5915:bool)
        n1237 = Not Equal?(x=w5918, y=w5919) -> (x != y?=w5917:bool)
        n1238 = feedback #16(1.0) -> (w5902:dbl)
        n1239 = Compound Arithmetic op=OR("Reset FFT", w5917, w5915) -> (w5900:bool)
        n1240 = Select(t=1.0, s=w5900, f=w5902) -> (s? t:f=w5904:dbl)
        n1241 = Greater?(x=w5904, y="# Spectra to Ave.") -> (0:w5923:bool)
        n1242 = Increment(x=w5904) -> (x+1=w5903:dbl)
        n1243 = local read "DMA Update Period (s)"() -> (w5898:dbl)
        n1244 = Multiply(x="# Spectra to Ave.", y=w5898) -> (x*y=→"Ave. Time (s)":dbl)
        n1245 = Build Array(cluster{"f0":dbl, "df":dbl, "magnitude":dbl[]} {"f0"=0.0, "df"=0.0, "magnitude"=[]} ("PSD")) -> (w5907:cluster{"f0":dbl, "df":dbl, "magnitude":dbl[]}[])
        n1246 = Build Array(w5907, w5907, w5907, w5907) -> (w5909:T40)
        n1247 = feedback #17(w5909) -> (w5914:T40)
        n1248 = for {
          N: 4 -> [_]
          tunnel: w5918 -> [w5947] mode=indexing
          tunnel: w5925 -> [w5948]
          tunnel: w5924 -> [w5950]
          tunnel: w5900 -> [w5943]
          tunnel: w5923 -> [w5942]
          tunnel: "# Spectra to Ave." -> [w5941]
          tunnel: [w5940] -> w5913 mode=indexing
          tunnel: w5914 -> [w5945] mode=indexing
          tunnel: [w5944] -> w5901 mode=indexing
          tunnel: w5904 -> [w5939]
          n1249 = Less?(x=w5947, y=w5950) -> (x < y?=w5949:bool)
          n1250 = Index Array(array=w5948, index=w5947) -> (element=w5946:waveform(dbl))
          n1251 = case shown="True" w5949 {
            tunnel: w5946 -> [_ w5967]
            tunnel: w5945 -> [w5952 w5965]
            tunnel: [w5952 w5953] -> w5944
            tunnel: w5943 -> [_ w5964]
            tunnel: w5942 -> [_ w5957]
            tunnel: w5941 -> [_ w5956]
            tunnel: [cluster{"f0":dbl, "df":dbl, "magnitude":dbl[]} {"f0"=0.0, "df"=0.0, "magnitude"=[]} ("PSD") w5958] -> w5940
            tunnel: w5939 -> [_ w5955]
            frame #0 {
            }
            frame #1 {
              n1252 = call <vilib>:"Std Deviation and Variance.vi"("X"=w5967) -> ("mean"=w5968:dbl)  [unwired: 1 in, 2 out]
              n1253 = Subtract(x=w5967, y=w5968) -> (x-y=w5966:waveform(dbl))
              n1254 = xnode "Spectral Measurements"("Signals"=w5966) -> ("PSD"=w5960:cluster{"f0":dbl, "df":dbl, "magnitude":dbl[]})  [unwired: 1 in, 1 out]
              n1255 = case shown="False" w5964 {
                tunnel: w5965 -> [w5977 _]
                tunnel: [w5973 w5982] -> w5953
                tunnel: w5960 -> [w5976 w5983]
                tunnel: w5957 -> [w5975 _]
                frame #0 {
                  n1256 = Build Array (concatenate)(w5977, w5976) -> (w5974:cluster{"f0":dbl, "df":dbl, "magnitude":dbl[]}[])
                  n1257 = case shown="True" w5975 {
                    tunnel: w5974 -> [w5978 w5981]
                    tunnel: [w5978 w5979] -> w5973
                    frame #0 {
                    }
                    frame #1 {
                      n1258 = Delete From Array(array=w5981, index=0) -> (array with subset deleted=w5979:cluster{"f0":dbl, "df":dbl, "magnitude":dbl[]}[])  [unwired: 1 in, 1 out]
                    }
                  }
                }
                frame #1 {
                  n1259 = Build Array(w5983) -> (w5982:cluster{"f0":dbl, "df":dbl, "magnitude":dbl[]}[])
                }
              }
              n1260 = for {
                tunnel: w5953 -> [w5972] mode=indexing
                tunnel: [w5971] -> w5963 mode=indexing
                n1261 = Unbundle By Name(w5972) -> ("magnitude"=w5971:dbl[])
              }
              n1262 = Transpose 2D Array(2D array=w5963) -> (transposed array=w5962:dbl[][])
              n1263 = for {
                tunnel: w5962 -> [w5970] mode=indexing
                tunnel: [w5969] -> w5961 mode=indexing
                n1264 = Add Array Elements(numeric array=w5970) -> (sum=w5969:dbl)
              }
              n1265 = Select(t=w5956, s=w5957, f=w5955) -> (s? t:f=w5954:dbl)
              n1266 = Divide(x=w5961, y=w5954) -> (x/y=w5959:dbl[])
              n1267 = Bundle By Name(cluster=w5960, "magnitude"=w5959) -> (w5958:cluster{"f0":dbl, "df":dbl, "magnitude":dbl[]})
            }
          }
        }
        n1268 = case shown="True" w5900 {
          tunnel: w5901 -> [w5932 w5938]
          tunnel: [w5932 w5933] -> w5899
          frame #0 {
          }
          frame #1 {
            n1269 = Array Subset(array=w5938, index (row)=0 ("index"), length (row)=4 ("length"), index (col)=0 ("index"), length (col)=1 ("length")) -> (w5933:T40)
          }
        }
        n1270 = Split 1D Array(array=w5913, index=2) -> (first subarray=→"FFT 1":cluster{"f0":dbl, "df":dbl, "magnitude":dbl[]}[], second subarray=→"FFT 2":cluster{"f0":dbl, "df":dbl, "magnitude":dbl[]}[])
      }
    }
    n1271 = Bundle("APD 1", "APD 2") -> (w3951:cluster{string, string})  [unwired: 1 out]
    n1272 = Cluster To Array(cluster=w3951) -> (array=w3948:string[])
    n1273 = for {
      tunnel: w3919 -> [w4961] mode=indexing
      tunnel: w3954 -> [w4970]
      tunnel: w3846 -> [w4969]
      tunnel: [w4965] -> w3952 mode=indexing
      tunnel: "APD Disp. Scale" -> [w4966]
      tunnel: w3827 -> [w4964]
      tunnel: w3948 -> [w4963] mode=indexing
      tunnel: "APD Disp. Downsample" -> [w4959]
      tunnel: [w4962] -> w3947
      n1274 = call "integrate 1D array interval - double.vi"("Ave N"=w4959, "Array In"=w4961) -> ("Array Out"=w4960:dbl[])  [unwired: 1 out]
      n1275 = Multiply(x=w4969, y=w4959) -> (x*y=w4962:dbl)
      n1276 = Divide(x=w4960, y=w4966) -> (x/y=w4967:dbl[])
      n1277 = To Time Stamp(1:w4970) -> (0:w4971:timestamp)
      n1278 = Bundle By Name("t0"=w4971, "Y"=w4967, "dt"=w4962) -> (w4968:waveform(dbl))  [unwired: 1 out]
      n1279 = Set Waveform Attribute(5:w4963, 6:w4964, 7:w4968) -> (3:w4965:waveform(dbl))  [unwired: 1 in, 2 out]
    }
    "APD Display Period (s)" <- w3947
    n1280 = Reciprocal(x=w3947) -> (1/x=→"APD Display Freq. (Hz)":dbl)
    n1281 = feedback #18(w3820) -> (w3917:u32[])
    n1282 = Build Array (concatenate)(w3917, w3820) -> (w3914:u32[])
    n1283 = Array Size(array=w3914) -> (size(s)=w3911:i32)
    n1284 = Array Size(array=w3820) -> (size(s)=w3913:i32)
    n1285 = Build Array (concatenate)(w3952, w3953) -> (w3772:waveform(dbl)[])
    "All Signals" <- w3772
    n1286 = local read "APD Integration Time (s)"() -> (w3780:dbl)
    n1287 = Multiply(x=w3913, y="APD Ave N") -> (x*y=w3912:dbl)
    n1288 = Greater?(x=w3911, y=w3912) -> (0:w3915:bool)
    n1289 = Index Array(array=w3772, index=0) -> (element=w3904:waveform(dbl))
    n1290 = case shown="True" w3915 {
      tunnel: w3914 -> [w4471 w4476]
      tunnel: [w4471 w4472] -> w3852
      tunnel: w3912 -> [_ w4474]
      tunnel: w3911 -> [_ w4475]
      frame #0 {
      }
      frame #1 {
        n1291 = Subtract(x=w4475, y=w4474) -> (x-y=w4473:dbl)
        n1292 = Array Subset(array=w4476, index=w4473, length=w4474) -> (w4472:u32[])
      }
    }
    n1293 = Multiply(x="APD Disp. Scale", y=w3904) -> (x*y=w3782:waveform(dbl))
    n1294 = Multiply(x="APD Disp. Downsample", y=w3780) -> (x*y=w3778:dbl)
    n1295 = Divide(x=w3782, y=w3778) -> (x/y=w3771:waveform(dbl))
    "APD 1 Chart" <- w3771
    n1296 = Index Array(array=w3772, index=3) -> (element=w3863:waveform(dbl))
    n1297 = Index Array(array=w3772, index=6) -> (element=w3860:waveform(dbl))
    n1298 = Array Size(array=w3852) -> (size(s)=w3909:i32)
    n1299 = Add Array Elements(numeric array=w3852) -> (sum=w3920:u32)
    n1300 = call <vilib>:"Std Deviation and Variance.vi"("X"=w3852) -> ("standard deviation"=w3851:dbl)  [unwired: 1 in, 2 out]
    n1301 = Divide(x="T1 offset_x (mV)", y=1000.0) -> (x/y=w3864:dbl)
    n1302 = Multiply(x=w3846, y=w3909) -> (x*y=w3910:dbl)
    "Int. Time (s)" <- w3910
    n1303 = Divide(x=w3920, y=w3910) -> (x/y=w3849:dbl)
    "APD 1 Rate (Hz)" <- w3849
    n1304 = Divide(x=w3851, y=w3846) -> (x/y=w3850:dbl)
    "Rate sigma (Hz)" <- w3850
    n1305 = Divide(x=w3850, y=w3849) -> (x/y=→"sigma/mean":dbl)
    n1306 = Divide(x="T2 offset_x (mV)", y=1000.0) -> (x/y=w3862:dbl)
    n1307 = case shown="0, Default" "Calibration" {
      tunnel: "T1 alpha_x (nm/V)" -> [_ w4448 w4469]
      tunnel: "T1 kappa_x (pN/nm)" -> [_ _ w4459]
      tunnel: "T2 alpha_x (nm/V)" -> [_ w4447 w4467]
      tunnel: "T2 kappa_x (pN/nm)" -> [_ _ w4460]
      tunnel: w3863 -> [w4430 w4445 w4465]
      tunnel: w3860 -> [w4429 w4443 w4463]
      tunnel: [w4430 w4442 w4462] -> w3893
      tunnel: [w4429 w4441 w4461] -> w3892
      tunnel: ["T1 X (V)" ("Label.Text") "T1 X (nm)" ("Label.Text") "T1 X (pN)" ("Label.Text")] -> w3881
      tunnel: ["T2 X (V)" ("Label.Text") "T2 X (nm)" ("Label.Text") "T2 X (pN)" ("Label.Text")] -> w3880
      tunnel: ["Position (V)" ("Label.Text") "Position (nm)" ("Label.Text") "Force (pN)" ("Label.Text")] -> w3882
      tunnel: w3862 -> [_ w4433 w4452]
      tunnel: w3864 -> [_ w4436 w4454]
      tunnel: ["Mean (V)" ("Label.Text") "Mean (nm)" ("Label.Text") "Mean (pN)" ("Label.Text")] -> w3877
      tunnel: ["Difference (V)" ("Label.Text") "Difference (nm)" ("Label.Text") "Difference (pN)" ("Label.Text")] -> w3783
      frame #0 {
      }
      frame #1 {
        n1308 = Unbundle By Name(w4445) -> ("Y"=w4449:dbl[])
        n1309 = Unbundle By Name(w4443) -> ("Y"=w4434:dbl[])
        n1310 = Subtract(x=w4449, y=w4436) -> (x-y=w4437:dbl[])
        n1311 = Subtract(x=w4434, y=w4433) -> (x-y=w4435:dbl[])
        n1312 = Multiply(x=w4435, y=w4447) -> (x*y=w4444:dbl[])
        n1313 = Multiply(x=w4448, y=w4437) -> (x*y=w4446:dbl[])
        n1314 = Bundle By Name(cluster=w4443, "Y"=w4444) -> (w4441:waveform(dbl))
        n1315 = Bundle By Name(cluster=w4445, "Y"=w4446) -> (w4442:waveform(dbl))
      }
      frame #2 {
        n1316 = Unbundle By Name(w4465) -> ("Y"=w4470:dbl[])
        n1317 = Unbundle By Name(w4463) -> ("Y"=w4468:dbl[])
        n1318 = Subtract(x=w4468, y=w4452) -> (x-y=w4453:dbl[])
        n1319 = Subtract(x=w4470, y=w4454) -> (x-y=w4455:dbl[])
        n1320 = Compound Arithmetic op=MULTIPLY(w4453, w4467, w4460) -> (w4464:dbl[])
        n1321 = Compound Arithmetic op=MULTIPLY(w4459, w4469, w4455) -> (w4466:dbl[])
        n1322 = Bundle By Name(cluster=w4463, "Y"=w4464) -> (w4461:waveform(dbl))
        n1323 = Bundle By Name(cluster=w4465, "Y"=w4466) -> (w4462:waveform(dbl))
      }
    }
    n1324 = feedback #19(u16 1 ("Calibration")) -> (w3884:u16)
    n1325 = case shown="True" "Read Lateness and Rel Phase" {
      tunnel: w3824 -> [w4116 w4134]
      tunnel: w3823 -> [w4117 w4133]
      tunnel: [w4116 w4132] -> w3855
      tunnel: [w4117 w4131] -> w3854
      frame #0 {
      }
      frame #1 {
        n1326 = xnode "Read/Write Control"("FPGA VI Reference In"=w4134, "error in"=w4133) -> ("FPGA VI Reference Out"=w4132:T15, "error out"=w4131:errorcluster, "GI Relative phase"=→"GI relative phase":i16, "Relative phase"=→"Relative phase (AI1)":i16, "AI Late Counter"=→"Late Counter (AI1)":u32, "GI Late Counter"=→"GI Late Counter":u32, "MCL Late Counter"=→"MCL Late Counter":u32, "MCL Relative Phase"=→"Relative Phase (MCL)":i16, "APD Acq Relative Phase"=→"APD Acq Relative Phase":i16, "APD Gate Relative Phase"=→"APD Gate Relative Phase":i16, "APD Acq Late Counter"=→"APD Acq Late Counter":u32, "APD Gate Late Counter"=→"APD Gate Late Counter":u32, "Green FB Relative Phase"=→"Relative phase (Green FB)":i16, "GI Relative phase 2"=→"GI relative phase 2":i16, "GI Late Counter 2"=→"GI Late Counter 2":u32)
      }
    }
    n1327 = Not Equal?(x=w3884, y="Calibration") -> (x != y?=w3829:bool)
    n1328 = Unbundle By Name(w3863) -> ("Y"=w3866:dbl[])
    n1329 = Unbundle By Name(w3860) -> ("Y"=w3869:dbl[])
    n1330 = Subtract(x=w3866, y=w3864) -> (x-y=w3867:dbl[])
    n1331 = Subtract(x=w3869, y=w3862) -> (x-y=w3868:dbl[])
    n1332 = Multiply(x=w3868, y="T2 alpha_x (nm/V)") -> (x*y=w3859:dbl[])
    n1333 = Multiply(x="T1 alpha_x (nm/V)", y=w3867) -> (x*y=w3858:dbl[])
    n1334 = Multiply(x=w3892, y=-1.0) -> (x*y=w3871:waveform(dbl))
    n1335 = Subtract(x=w3859, y=w3858) -> (x-y=w3857:dbl[])
    n1336 = Unbundle By Name(w3892) -> ("Y"=w3811:dbl[])
    n1337 = Unbundle By Name(w3893) -> ("Y"=w3812:dbl[])
    n1338 = Build Array(w3893, w3871) -> (→"Force":waveform(dbl)[])
    n1339 = Subtract(x=w3857, y="Offset (nm)") -> (x-y=w3809:dbl[])
    n1340 = call <vilib>:"Mean.vi"("X"=w3811) -> ("mean"=w3787:dbl)  [unwired: 1 out]
    "T2 X" <- w3787
    n1341 = Absolute Value(x=w3812) -> (abs(x)=w3813:dbl[])
    n1342 = Absolute Value(x=w3811) -> (abs(x)=w3814:dbl[])
    n1343 = call <vilib>:"Mean.vi"("X"=w3812) -> ("mean"=w3788:dbl)  [unwired: 1 out]
    "T1 X" <- w3788
    n1344 = Add(x=w3813, y=w3814) -> (x+y=w3815:dbl[])
    n1345 = Bundle By Name(cluster=w3863, "Y"=w3809) -> (w3770:waveform(dbl))
    "Bead Separation" <- w3770
    n1346 = Divide(x=w3815, y=2.0) -> (x/y=→"Vec Mean of T1 T2":dbl[])
    n1347 = case shown="True" w3829 {
      tunnel: w3882 -> [_ w4423]
      tunnel: w3881 -> [_ w4422]
      tunnel: w3880 -> [_ w4421]
      tunnel: w3877 -> [_ w4420]
      tunnel: w3783 -> [_ w4419]
      frame #0 {
      }
      frame #1 {
        n1348 = property on="Force" class="WFChart (strict)"("YScale.NameLbl.Text"=w4423) -> ()  [unwired: 2 in, 2 out]
        n1349 = property on="T2 X" class="DigNum (strict)"("Caption.Text"=w4421) -> ()  [unwired: 2 in, 2 out]
        n1350 = property on="T1 X" class="DigNum (strict)"("Caption.Text"=w4422) -> ()  [unwired: 2 in, 2 out]
        n1351 = property on="Mean" class="DigNum (strict)"("Caption.Text"=w4420) -> ()  [unwired: 2 in, 2 out]
        n1352 = property on="Difference" class="DigNum (strict)"("Caption.Text"=w4419) -> ()  [unwired: 2 in, 2 out]
      }
    }
    n1353 = local read "Tether"() -> (w3818:bool)
    n1354 = Absolute Value(x=w3788) -> (abs(x)=w3785:dbl)
    n1355 = Absolute Value(x=w3787) -> (abs(x)=w3784:dbl)
    n1356 = local read "Display Period (s)"() -> (w3802:dbl)
    n1357 = Add(x=w3785, y=w3784) -> (x+y=w3879:dbl)
    n1358 = Subtract(x=w3785, y=w3784) -> (x-y=→"Difference":dbl)
    n1359 = feedback #20(w3809) -> (w3808:dbl[])
    n1360 = Divide(x=w3879, y=2.0) -> (x/y=w3817:dbl)
    "Mean" <- w3817
    n1361 = case shown="True" w3818 {
      tunnel: w3817 -> [_ w4072]
      frame #0 {
      }
      frame #1 {
        n1362 = Greater?(x="Lost Tether Alarm Threshold (pN)", y=w4072) -> (0:w4070:bool)
        n1363 = case shown="True" w4070 {
          frame #0 {
          }
          frame #1 {
            n1364 = local read "Time tether formed"() -> (w4078:timestamp)
            n1365 = Get Date/Time In Seconds() -> (seconds since 1Jan1904=w4079:timestamp)
            n1366 = Subtract(x=w4079, y=w4078) -> (x-y=w4077:dbl)
            n1367 = Number To Decimal String(number=w4077) -> (decimal integer string=w4074:string)  [unwired: 1 out]
            n1368 = local read "Messages"() -> (w4081:string)
            n1369 = call <vilib>:"Beep.vi"() -> ()  [unwired: 3 in, 9 out]
            n1370 = Concatenate Strings("Lost tether (" ("Message to add"), w4074, " s)." ("string")) -> (w4076:string)
            n1371 = local write "Tether"(FALSE ("Tether")) -> ()
            n1372 = call "Update messages.vi"("Message to add"=w4076, "Old message string"=w4081) -> ("New message string"=w4080:string)
            n1373 = local write "Messages"(w4080) -> ()
          }
        }
      }
    }
    n1374 = Build Array (concatenate)(w3809, w3808) -> (w3807:dbl[])
    n1375 = Divide(x="Bead Sep. Int. Time (s)", y=w3802) -> (x/y=w3801:dbl)
    n1376 = Split 1D Array(array=w3807, index=w3801) -> (first subarray=w3800:dbl[])  [unwired: 1 out]
    n1377 = xnode "Read/Write Control"("FPGA VI Reference In"=w3855, "error in"=w3854) -> ("FPGA VI Reference Out"=w3983:T15, "error out"=w3977:errorcluster, "AI2 Y Sum Set 1"=w3973:i16, "AI2 Y Sum Set 2"=w3972:i16, "Scanning"=→"AOD Scanning":bool, "Scan I"=→"AOD Scan I":u64, "Scanning MCL"=w3975:bool, "Scan I (MCL)"=→"MCL Scan I":u64, "Green FB Signals"=w3902:T35)  [unwired: 1 out]
    "MCL Scanning" <- w3975
    n1378 = call <vilib>:"Mean.vi"("X"=w3800) -> ("mean"=w3799:dbl)  [unwired: 1 out]
    "Bead Mean (nm)" <- w3799
    n1379 = Subtract(x=w3800, y=w3799) -> (x-y=w3798:dbl[])
    n1380 = Square(x=w3798) -> (x^2=w3797:dbl[])
    n1381 = call <vilib>:"Mean.vi"("X"=w3797) -> ("mean"=w3796:dbl)  [unwired: 1 out]
    n1382 = Square Root(x=w3796) -> (sqrt(x)=w3795:dbl)
    n1383 = Multiply(x=10.0, y=w3795) -> (x*y=→"RMS (Ang)":dbl)
    n1384 = flat-sequence "To save data" {
      tunnel: [w6366] -> w3996
      tunnel: [w6367] -> w3995
      tunnel: w3936 -> [w6360]
      tunnel: w3805 -> [w6364]
      tunnel: ["Save Calibration"] -> w3964
      tunnel: w3959 -> [w6363]
      tunnel: [w6356] -> w3958
      tunnel: [w6353] -> w3956
      tunnel: [w6350] -> w3955
      tunnel: w3935 -> [w6352]
      tunnel: w3826 -> [w6346]
      tunnel: [w6346] -> w3825
      tunnel: ["Start Saving"] -> w3773
      tunnel: w3996 -> [w6556]
      tunnel: w3995 -> [w6555]
      tunnel: w3994 -> [w6554]
      tunnel: w3964 -> [w6553]
      tunnel: w3958 -> [w6551]
      tunnel: w3956 -> [w6550]
      tunnel: w3955 -> [w6549]
      tunnel: w3789 -> [w6548]
      tunnel: w3847 -> [w6547]
      tunnel: w3825 -> [w6546]
      tunnel: w3773 -> [w6545]
      tunnel: w3771 -> [w6544]
      tunnel: w3770 -> [w6543]
      frame #0 {
        n1385 = Or(x="Save N Sets", y="Start Saving") -> (x .or. y?=w6347:bool)
        n1386 = To Double Precision Float(number=w6363) -> (double precision float=w6357:dbl)
        n1387 = Build Array(w6347, "Save Calibration", w6360, w6352) -> (w6362:bool[])
        n1388 = Compound Arithmetic op=OR("Save Calibration", w6360, w6347, w6352) -> (w6365:bool)
        n1389 = Boolean Array To Number(Boolean array=w6362) -> (number=w6359:u32)
        n1390 = feedback #21(refnum<k0> refnum) -> (w6368:refnum<file>)
        n1391 = feedback #22(FALSE ("Save APD Data\nwith Trap Data")) -> (w6351:bool)
        n1392 = feedback #23(refnum<k0> refnum) -> (w6354:refnum<file>)
        n1393 = feedback #24(0) -> (w6370:i32)
        n1394 = feedback #25() -> (w6358:u32)  [unwired: 1 out]
        n1395 = case shown="True" w6365 {
          tunnel: [w6375 1] -> w6366
          tunnel: w6370 -> [w6377 _]
          tunnel: [w6376 w6390] -> w6367
          tunnel: w6368 -> [w6376 _]
          tunnel: w6364 -> [_ w6410]
          tunnel: w6357 -> [_ w6408]
          tunnel: w6359 -> [_ w6411]
          tunnel: [w6374 w6389] -> w6356
          tunnel: w6358 -> [w6374 _]
          tunnel: [w6373 w6386] -> w6353
          tunnel: w6354 -> [w6373 _]
          tunnel: [w6372 w6385] -> w6350
          tunnel: w6351 -> [w6372 _]
          tunnel: "Start Saving" -> [_ w6383]
          tunnel: w6346 -> [_ w6382]
          frame #0 {
            n1396 = Increment(x=w6377) -> (x+1=w6375:i32)
          }
          frame #1 {
            w6378 = FALSE ("Start Saving")
            w6384 = 9.0  # File Version
            w6393 = FALSE ("prepend array or string size? (T)")
            w6391 = T24."big-endian, network order" ("byte order (0:big-endian, network order)")
            n1397 = Array Size(array=w6382) -> (size(s)=w6381:i32)
            n1398 = local read "BD 1 Frequency 1 (MHz)"() -> (w6407:dbl)
            n1399 = local read "BD 2 Frequency 1 (MHz)"() -> (w6406:dbl)
            n1400 = local read "BD 1 Frequency 2 (MHz)"() -> (w6405:dbl)
            n1401 = local read "BD 2 Frequency 2 (MHz)"() -> (w6404:dbl)
            n1402 = local read "BD 1 Frequency 3 (MHz)"() -> (w6403:dbl)
            n1403 = local read "BD 2 Frequency 3 (MHz)"() -> (w6402:dbl)
            n1404 = To Double Precision Float(number=w6381) -> (double precision float=w6380:dbl)
            n1405 = local write "Start Saving"(w6378) -> ()
            n1406 = local write "Save Calibration"(w6378) -> ()
            n1407 = Build Array(w6407, w6406, w6405, w6404, w6403, w6402) -> (w6401:dbl[])
            n1408 = case shown="1, Default" w6411 {
              tunnel: w6410 -> [w6455 w6469 w6484 w6521]
              tunnel: w6380 -> [w6460 w6476 w6504 w6540]
              tunnel: w6408 -> [w6459 w6475 w6503 w6539]
              tunnel: [w6456 w6471 w6495 w6531] -> w6399
              tunnel: [w6445 "Cal sets to save" w6485 w6522] -> w6389
              tunnel: w6401 -> [w6457 w6472 w6497 w6533]
              tunnel: "Save APD Data\nwith Trap Data" -> [w6454 _ w6480 w6518]
              tunnel: [w6454 w6465 w6480 w6518] -> w6385
              tunnel: w6384 -> [w6448 w6463 w6478 w6516]
              tunnel: w6383 -> [w6447 _ _ _]
              frame #0 {
                w6451 = 0.0 ("f")
                # "timeseries"
                n1409 = local read "Save ave N"() -> (w6462:dbl)
                n1410 = Multiply(x=w6462, y=w6455) -> (x*y=w6461:dbl)
                n1411 = Boolean To (0,1)(Boolean=w6454) -> (0, 1=w6453:i16)
                n1412 = To Double Precision Float(number=w6453) -> (double precision float=w6452:dbl)
                n1413 = Build Array(w6448, w6455, w6461, w6460, w6459, 0.0 ("f")) -> (w6458:dbl[])
                n1414 = Build Array(w6452, w6451, w6451, w6451, w6451) -> (w6449:dbl[])
                n1415 = Select(t=u32 4000000000, s=w6447, f="N sets to save") -> (s? t:f=w6445:u32)
                n1416 = Build Array (concatenate)(w6458, w6457, w6449) -> (w6456:dbl[])
              }
              frame #1 {
                w6466 = 0.0 ("f")
                w6465 = FALSE ("Save APD Data\nwith Trap Data")
                # "calibration"
                n1417 = Boolean To (0,1)(Boolean=w6465) -> (0, 1=w6468:i16)
                n1418 = To Double Precision Float(number=w6468) -> (double precision float=w6467:dbl)
                n1419 = Build Array(w6467, w6466, w6466, w6466, w6466) -> (w6464:dbl[])
                n1420 = Build Array(w6463, w6469, w6469, w6476, w6475, 1.0 ("t")) -> (w6473:dbl[])
                n1421 = Build Array (concatenate)(w6473, w6472, w6464) -> (w6471:dbl[])
                "Calibrating Trap..." <- TRUE ("Calibrating...")
              }
              frame #2 {
                w6481 = 0.0 ("f")
                # "scan dir (x/y = 0/1)"
                # "cycles/step"
                # "n scans (f/b)"
                # "steps"
                # "freq. range"
                # "AOD raster scan"
                n1422 = local read "Number of F/B Scans (AOD)"() -> (w6489:u16)
                n1423 = local read "Cycles/step (AOD)"() -> (w6491:u64)
                n1424 = local read "Scan Range (MHz)"() -> (w6494:dbl)
                n1425 = local read "Scan steps (AOD)"() -> (w6493:u64)
                n1426 = local read "Scan BD"() -> (w6501:bool)
                n1427 = local read "Save ave N"() -> (w6506:dbl)
                n1428 = Boolean To (0,1)(Boolean=w6501) -> (0, 1=w6500:i16)
                n1429 = To Double Precision Float(number=w6489) -> (double precision float=w6488:dbl)
                n1430 = To Double Precision Float(number=w6493) -> (double precision float=w6492:dbl)
                n1431 = To Double Precision Float(number=w6491) -> (double precision float=w6490:dbl)
                n1432 = To Double Precision Float(number=w6500) -> (double precision float=w6499:dbl)
                n1433 = Boolean To (0,1)(Boolean=w6480) -> (0, 1=w6483:i16)
                n1434 = Multiply(x=w6506, y=w6484) -> (x*y=w6505:dbl)
                n1435 = To Double Precision Float(number=w6483) -> (double precision float=w6482:dbl)
                n1436 = Build Array(w6482, w6481, w6481, w6481, w6481) -> (w6479:dbl[])
                n1437 = local read "N sets should be saved"() -> (w6486:dbl)
                n1438 = Build Array(w6499, w6494, w6492, w6490, w6488) -> (w6496:dbl[])
                n1439 = Build Array(w6478, w6484, w6505, w6504, w6503, 2.0 ("t")) -> (w6498:dbl[])
                n1440 = Round Toward +Infinity(x=w6486) -> (ceil(x): smallest int >= x=w6487:dbl)
                n1441 = Build Array (concatenate)(w6498, w6497, w6479, w6496) -> (w6495:dbl[])
                n1442 = To Unsigned Long Integer(number=w6487) -> (unsigned 32bit integer=w6485:u32)
              }
              frame #3 {
                w6513 = 0.0 ("f")
                # "MCL raster scan"
                n1443 = local read "Number of scans (MCL)"() -> (w6508:u64)
                n1444 = local read "Scan lines (y)"() -> (w6507:u64)
                n1445 = local read "2D or 1D Scan"() -> (w6510:bool)
                n1446 = local read "Scan Range (V)\n(of steps)"() -> (w6530:dbl)
                n1447 = local read "Fast Scan Dir"() -> (w6537:bool)
                n1448 = local read "Cycles/step (MCL)"() -> (w6527:u64)
                n1449 = Select(t=w6507, s=w6510, f=w6508) -> (s? t:f=w6509:u64)
                n1450 = local read "Scan steps (MCL)"() -> (w6529:u64)
                n1451 = Boolean To (0,1)(Boolean=w6510) -> (0, 1=w6512:i16)
                n1452 = local read "Save ave N"() -> (w6542:dbl)
                n1453 = local read "Initial X"() -> (w6515:dbl)
                n1454 = local read "Initial Y"() -> (w6514:dbl)
                n1455 = To Double Precision Float(number=w6512) -> (double precision float=w6511:dbl)
                n1456 = Boolean To (0,1)(Boolean=w6537) -> (0, 1=w6536:i16)
                n1457 = To Double Precision Float(number=w6509) -> (double precision float=w6525:dbl)
                n1458 = To Double Precision Float(number=w6529) -> (double precision float=w6528:dbl)
                n1459 = To Double Precision Float(number=w6527) -> (double precision float=w6526:dbl)
                n1460 = To Double Precision Float(number=w6536) -> (double precision float=w6535:dbl)
                n1461 = Boolean To (0,1)(Boolean=w6518) -> (0, 1=w6520:i16)
                n1462 = Multiply(x=w6542, y=w6521) -> (x*y=w6541:dbl)
                n1463 = To Double Precision Float(number=w6520) -> (double precision float=w6519:dbl)
                n1464 = local read "N sets should be saved (MCL)"() -> (w6523:dbl)
                n1465 = Build Array(w6519, w6511, w6513, w6513, w6513) -> (w6517:dbl[])
                n1466 = Build Array(w6535, w6530, w6528, w6526, w6525, w6515, w6514) -> (w6532:dbl[])
                n1467 = Build Array(w6516, w6521, w6541, w6540, w6539, 3.0 ("t")) -> (w6534:dbl[])
                n1468 = Round Toward +Infinity(x=w6523) -> (ceil(x): smallest int >= x=w6524:dbl)
                n1469 = Build Array (concatenate)(w6534, w6533, w6517, w6532) -> (w6531:dbl[])
                n1470 = To Unsigned Long Integer(number=w6524) -> (unsigned 32bit integer=w6522:u32)
              }
            }
            n1471 = local read "Index"() -> (w6416:dbl)
            n1472 = call "Create new save file.vi"("Insert"="", "Ext"=".dat", "Index In"=w6416) -> ("Path Out"=w6387:path, "Index Out"=w6388:dbl)
            n1473 = local write "Index"(w6388) -> ()
            n1474 = local write "Save file name"(w6387) -> ()
            n1475 = local write "Save index"(w6388) -> ()
            n1476 = Array Size(array=w6399) -> (size(s)=w6400:i32)
            n1477 = Open/Create/Replace File(file path (use dialog)=w6387, operation (0:open)=T25."create", access (0:read/write)=enum16{"read/write", "read-only", "write-only"}."write-only") -> (refnum out=w6413:refnum<file>)  [unwired: 1 in, 4 out]
            n1478 = local write "Saving..."(TRUE ("Saving...")) -> ()
            n1479 = To Double Precision Float(number=w6400) -> (double precision float=w6398:dbl)
            n1480 = String Length(string="Comment (data description)") -> (length=w6396:i32)
            n1481 = To Double Precision Float(number=w6396) -> (double precision float=w6395:dbl)
            n1482 = Deny Access(7:w6413) -> (3:w6412:refnum<file>)  [unwired: 1 in, 2 out]
            n1483 = Build Array (concatenate)(w6398, w6399, w6395) -> (w6397:dbl[])
            n1484 = case "If fluorescence data to be saved" shown="True" w6385 {
              tunnel: w6387 -> [_ w6443]
              tunnel: [refnum<k0> refnum w6423] -> w6386
              frame #0 {
              }
              frame #1 {
                w6422 = 0.0
                n1485 = local read "APD Integration Time (s)"() -> (w6428:dbl)
                n1486 = local read "N APD Samp/step"() -> (w6421:dbl)
                n1487 = Path To String(path=w6443) -> (string=w6442:string)
                n1488 = String Length(string=w6442) -> (length=w6441:i32)
                n1489 = Subtract(x=w6441, y=4) -> (x-y=w6439:i32)
                n1490 = String Subset(string=w6442, length (rest)=w6439) -> (substring=w6438:string)  [unwired: 1 out]
                n1491 = Build Array(w6428, w6421, w6422, w6422, w6422, w6422, w6422, w6422) -> (w6425:dbl[])
                n1492 = Concatenate Strings(w6438, "_fl.dat" ("string")) -> (w6436:string)
                n1493 = Array Size(array=w6425) -> (size(s)=w6427:i32)
                n1494 = String To Path(string=w6436) -> (path=w6432:path)
                n1495 = Open/Create/Replace File(file path (use dialog)=w6432, operation (0:open)=T25."create", access (0:read/write)=enum16{"read/write", "read-only", "write-only"}."write-only") -> (refnum out=w6433:refnum<file>)  [unwired: 1 in, 4 out]
                n1496 = Deny Access(7:w6433) -> (3:w6429:refnum<file>)  [unwired: 1 in, 2 out]
                n1497 = To Double Precision Float(number=w6427) -> (double precision float=w6426:dbl)
                n1498 = Build Array (concatenate)(w6426, w6425) -> (w6424:dbl[])
                n1499 = Write to Binary File(file (use dialog)=w6429, data=w6424, 5:FALSE ("prepend array or string size? (T)"), 9:T24."big-endian, network order" ("byte order (0:big-endian, network order)")) -> (refnum out=w6423:refnum<file>)  [unwired: 1 in, 3 out]
              }
            }
            n1500 = Write to Binary File(file (use dialog)=w6412, data=w6397, 5:w6393, 9:w6391) -> (refnum out=w6394:refnum<file>)  [unwired: 1 in, 3 out]
            n1501 = Write to Binary File(file (use dialog)=w6394, data="Comment (data description)", 5:w6393, 9:w6391) -> (refnum out=w6390:refnum<file>)  [unwired: 1 in, 3 out]
          }
        }
      }
      frame #1 {
        n1502 = local read "Saving..."() -> (w6552:bool)
        n1503 = case shown="True" w6552 {
          tunnel: w6556 -> [_ w6563]
          tunnel: w6555 -> [_ w6577]
          tunnel: w6554 -> [_ w6573]
          tunnel: w6553 -> [_ w6572]
          tunnel: w6551 -> [_ w6571]
          tunnel: w6550 -> [_ w6566]
          tunnel: w6549 -> [_ w6565]
          tunnel: w6548 -> [_ w6564]
          tunnel: w6547 -> [_ w6562]
          tunnel: w6546 -> [_ w6560]
          tunnel: w6545 -> [_ w6559]
          tunnel: w6544 -> [_ w6558]
          tunnel: w6543 -> [_ w6557]
          frame #0 {
          }
          frame #1 {
            n1504 = Multiply(x=w6563, y=w6562) -> (x*y=→"Time (s)":dbl)
            n1505 = Less Or Equal?(x=w6563, y=w6571) -> (x <= y?=w6575:bool)
            n1506 = Or(x="Stop Saving", y="Abort save 2") -> (x .or. y?=w6567:bool)
            n1507 = Not(x=w6567) -> (.not. x?=w6576:bool)
            n1508 = And(x=w6575, y=w6576) -> (x .and. y?=w6574:bool)
            n1509 = case shown="True" w6574 {
              tunnel: w6577 -> [w6582 w6609]
              tunnel: [0.0 w6612] -> w6570
              tunnel: w6563 -> [_ w6610]
              tunnel: w6571 -> [_ w6611]
              tunnel: w6573 -> [_ w6606]
              tunnel: w6572 -> [_ _]
              tunnel: w6566 -> [w6579 w6597]
              tunnel: w6565 -> [w6578 w6598]
              tunnel: w6564 -> [_ w6596]
              tunnel: w6560 -> [_ w6595]
              tunnel: w6559 -> [_ w6586]
              tunnel: w6558 -> [_ w6585]
              tunnel: w6557 -> [_ w6584]
              frame #0 {
                w6580 = FALSE
                n1510 = Close File(refnum=w6582) -> ()  [unwired: 1 in, 2 out]
                n1511 = case shown="True" w6578 {
                  tunnel: w6579 -> [_ w6583]
                  frame #0 {
                  }
                  frame #1 {
                    n1512 = Close File(refnum=w6583) -> ()  [unwired: 1 in, 2 out]
                  }
                }
                n1513 = local write "Raster Scanning..."(w6580) -> ()
                n1514 = local write "Calibrating Trap..."(w6580) -> ()
                n1515 = call <vilib>:"Beep.vi"() -> ()  [unwired: 3 in, 9 out]
                "Saving..." <- w6580
              }
              frame #1 {
                n1516 = local read "Calibrating Trap..."() -> (w6599:bool)
                n1517 = case shown="True" w6598 {
                  tunnel: w6597 -> [_ w6616]
                  tunnel: w6596 -> [_ w6615]
                  frame #0 {
                  }
                  frame #1 {
                    n1518 = Write to Binary File(file (use dialog)=w6616, data=w6615, 5:FALSE ("prepend array or string size? (T)"), 9:T24."big-endian, network order" ("byte order (0:big-endian, network order)")) -> ()  [unwired: 1 in, 4 out]
                  }
                }
                n1519 = Greater?(x="Save ave N", y=1.0) -> (0:w6602:bool)
                n1520 = Not(x=w6599) -> (.not. x?=w6601:bool)
                n1521 = And(x=w6601, y=w6602) -> (x .and. y?=w6603:bool)
                n1522 = case shown="False" w6603 {
                  tunnel: w6606 -> [w6619 w6631]
                  tunnel: [w6619 w6623] -> w6600
                  tunnel: "Save ave N" -> [_ w6624]
                  tunnel: w6595 -> [_ w6622]
                  frame #0 {
                  }
                  frame #1 {
                    n1523 = Array Size(array=w6631) -> (size(s)=w6625:i32)
                    n1524 = Array Size(array=w6622) -> (size(s)=w6621:i32)
                    n1525 = Divide(x=w6625, y=w6621) -> (x/y=w6629:dbl)
                    n1526 = Reshape Array(w6631, w6629, w6621) -> (w6630:i16[][])
                    n1527 = Transpose 2D Array(2D array=w6630) -> (transposed array=w6628:i16[][])
                    n1528 = for {
                      tunnel: w6628 -> [w6634] mode=indexing
                      tunnel: [w6633] -> w6620 mode=indexing
                      tunnel: w6624 -> [w6632]
                      n1529 = call "downsample 1D array - I16.vi"("Ave N"=w6632, "Array In"=w6634) -> ("Array Out"=w6633:i16[])  [unwired: 1 out]
                    }
                    n1530 = Transpose 2D Array(2D array=w6620) -> (transposed array=w6627:i16[][])
                    n1531 = Divide(x=w6625, y=w6624) -> (x/y=w6626:dbl)
                    n1532 = Reshape Array(w6627, w6626) -> (w6623:i16[])
                  }
                }
                n1533 = Unbundle By Name(w6584) -> ("Y"=w6590:dbl[])
                n1534 = Unbundle By Name(w6585) -> ("Y"=w6594:dbl[])
                n1535 = Write to Binary File(file (use dialog)=w6609, data=w6600, 5:FALSE ("prepend array or string size? (T)"), 9:T24."big-endian, network order" ("byte order (0:big-endian, network order)")) -> ()  [unwired: 1 in, 4 out]
                n1536 = feedback #26(w6590) -> (w6589:dbl[])
                n1537 = Build Array (concatenate)(w6589, w6590) -> (w6588:dbl[])
                n1538 = Select(t=w6590, s=w6586, f=w6588) -> (s? t:f=w6587:dbl[])
                "Trap Delta Graph" <- w6587
                n1539 = feedback #27(w6594) -> (w6593:dbl[])
                n1540 = Build Array (concatenate)(w6593, w6594) -> (w6592:dbl[])
                n1541 = Select(t=w6594, s=w6586, f=w6592) -> (s? t:f=w6591:dbl[])
                "APD 1 Graph" <- w6591
                n1542 = Divide(x=w6610, y=w6611) -> (x/y=w6613:dbl)
                n1543 = Multiply(x=w6613, y=100.0) -> (x*y=w6612:dbl)
              }
            }
            "Progress" <- w6570
            "Progress 2" <- w6570
          }
        }
      }
    }
    n1544 = local read "AI2 (V)"() -> (w3974:cluster{"Set 1":dbl, "Set 2":dbl})
    n1545 = Bundle By Name(cluster=w3974, "Set 1"=w3973, "Set 2"=w3972) -> (w3970:cluster{"Set 1":dbl, "Set 2":dbl})
    n1546 = Divide(x=w3970, y=3276.7) -> (x/y=w3969:cluster{"Set 1":dbl, "Set 2":dbl})
    n1547 = local write "AI2 (V)"(w3969) -> ()
    n1548 = Divide(x=w3902, y=3276.7) -> (x/y=w3898:T41)
    n1549 = Unbundle By Name(w3898) -> ("Green FB Ch 0"=w3901:dbl, "Green FB Ch 1"=w3900:dbl, "Green FB Ch 2"=w3899:dbl)
    n1550 = Divide(x=w3901, y=w3899) -> (x/y=w3897:dbl)
    n1551 = Divide(x=w3900, y=w3899) -> (x/y=w3896:dbl)
    n1552 = Bundle By Name(cluster=w3898, "Green FB Ch 0"=w3897, "Green FB Ch 1"=w3896) -> (w3876:T41)
    "Green FB Signals (V)" <- w3876
    n1553 = Unbundle By Name(w3876) -> ("Green FB Ch 2"=→"Green FB Plot":dbl)
    n1554 = local read "wait to reset values"() -> (w3978:bool)
    n1555 = Not(x=w3975) -> (.not. x?=w3979:bool)
    n1556 = And(x=w3979, y=w3978) -> (x .and. y?=w3980:bool)
    n1557 = case "Part of MCL raster scanning: returns to initial positions after scan done" shown="True" w3980 {
      tunnel: w3983 -> [w5312 w5319]
      tunnel: [w5312 w5318] -> w3982
      tunnel: w3977 -> [w5311 w5317]
      tunnel: [w5311 w5316] -> w3976
      frame #0 {
      }
      frame #1 {
        w5327 = 10.0 ("y")
        w5326 = 32767.0 ("y")
        # "to return scan values\nafter a synchronous \nAOM scan"
        n1558 = local read "AO2"() -> (w5320:dbl)
        n1559 = local read "AO1"() -> (w5321:dbl)
        n1560 = Multiply(x=w5321, y=w5326) -> (x*y=w5323:dbl)
        n1561 = Multiply(x=w5320, y=w5326) -> (x*y=w5325:dbl)
        n1562 = local write "wait to reset values"(FALSE ("wait to reset values")) -> ()
        n1563 = Divide(x=w5323, y=w5327) -> (x/y=w5322:dbl)
        n1564 = Divide(x=w5325, y=w5327) -> (x/y=w5324:dbl)
        n1565 = To Word Integer(number=w5322) -> (16bit integer=w5328:i16)
        n1566 = To Word Integer(number=w5324) -> (16bit integer=w5329:i16)
        n1567 = local read "Total Counts (ticks)"() -> (w5313:u32)
        n1568 = xnode "Read/Write Control"("FPGA VI Reference In"=w5319, "error in"=w5317, "AO1"=w5328, "AO2"=w5329, "MCL count"=w5313) -> ("FPGA VI Reference Out"=w5318:T15, "error out"=w5316:errorcluster)
        n1569 = local read "Scan Range (V)\n(of steps)"() -> (w5314:dbl)
        n1570 = property on="Scan Range (V)\n(of steps)" class="DigNum (strict)"("Val(Sgnl)"=w5314) -> ()  [unwired: 2 in, 2 out]
      }
    }
    n1571 = node-c288() -> ()  [unwired: 2 out]
  }
  n1572 = timed-loop "Rough control of MCL mirror stage (debugging)" {
    tunnel: w80 -> [w6709]
    tunnel: [w6708] -> w186
    timing: w11 -> [_]
    timing-out: [_] -> w10
    stop <- w6708 stop-if-true
    n1573 = node-c288() -> ()  [unwired: 2 out]
    n1574 = case shown="1" "MCL Mode" {
      tunnel: w6709 -> [_ w6712 w6814]
      frame #0 {
      }
      frame #1 {
        n1575 = node-c288() -> (w6714:T18)  [unwired: 4 out]
        n1576 = timed-loop "Oscillate MCL mirror" {
          timing: w6714 -> [_]
          timing-out: [_] -> w6713
          tunnel: w6712 -> [w6753]
          i -> [w6752]
          stop <- w6715 stop-if-true
          n1577 = node-c288() -> (w6751:i64)  [unwired: 1 out]
          n1578 = Multiply(x="AO1", y=32767.0) -> (x*y=w6747:dbl)
          n1579 = Multiply(x="AO2", y=32767.0) -> (x*y=w6742:dbl)
          n1580 = Divide(x=w6747, y=10.0) -> (x/y=w6748:dbl)
          n1581 = Divide(x=w6742, y=10.0) -> (x/y=w6743:dbl)
          n1582 = To Word Integer(number=w6748) -> (16bit integer=w6740:i16)
          n1583 = To Word Integer(number=w6743) -> (16bit integer=w6739:i16)
          n1584 = Divide(x=w6751, y=i64 1000) -> (x/y=w6722:dbl)
          n1585 = Multiply(x=w6722, y=w6752) -> (x*y=w6733:dbl)
          n1586 = Multiply(x="Osc. freq. (Hz) 2", y=6.283185307179586) -> (x*y=w6734:dbl)
          n1587 = Multiply(x=w6734, y=w6733) -> (x*y=w6732:dbl)
          n1588 = Sine(x=w6732) -> (sin(x)=w6731:dbl)
          n1589 = Multiply(x=w6731, y="Osc. amp. (V)") -> (x*y=w6729:dbl)
          n1590 = Add(x=w6729, y="Osc. center (V)") -> (x+y=w6727:dbl)
          n1591 = Divide(x=w6727, y=10.0) -> (x/y=w6725:dbl)
          n1592 = Multiply(x=w6725, y=32767.0) -> (x*y=w6720:dbl)
          n1593 = Select(t=w6720, s="Scan axis", f=w6740) -> (s? t:f=w6738:dbl)
          n1594 = Select(t=w6739, s="Scan axis", f=w6720) -> (s? t:f=w6737:dbl)
          n1595 = local read "MCL Mode"() -> (w6719:u16)
          n1596 = Not Equal?(x=w6719, y=u16 1) -> (x != y?=w6716:bool)
          n1597 = local read "Stop All"() -> (w6717:bool)
          n1598 = xnode "Read/Write Control"("FPGA VI Reference In"=w6753, "AO1"=w6738, "AO2"=w6737) -> ()  [unwired: 1 in, 2 out]
          n1599 = Compound Arithmetic op=OR(w6717, w6716) -> (w6715:bool)
          n1600 = node-c288() -> ()  [unwired: 2 out]
        }
        n1601 = node-c288(w6713) -> ()  [unwired: 1 out]
      }
      frame #2 {
        n1602 = case shown="True" "Start Scan" {
          tunnel: w6814 -> [_ w6826]
          frame #0 {
          }
          frame #1 {
            n1603 = Subtract(x="End (V)", y="Begin (V)") -> (x-y=w6822:dbl)
            n1604 = Decrement(x="N Points") -> (x-1=w6821:dbl)
            n1605 = Divide(x=w6822, y=w6821) -> (x/y=w6819:dbl)
            n1606 = for {
              N: "N Points" -> [_]
              tunnel: "Begin (V)" -> [w6839]
              tunnel: w6826 -> [w6831]
              tunnel: [w6830] -> w6825 mode=indexing
              tunnel: w6819 -> [w6829]
              tunnel: [w6827] -> w6818 mode=indexing
              i -> [w6838]
              n1607 = Multiply(x=w6829, y=w6838) -> (x*y=w6837:dbl)
              n1608 = Add(x=w6839, y=w6837) -> (x+y=w6834:dbl)
              n1609 = local read "Scan axis"() -> (w6828:bool)
              n1610 = local read "AO1"() -> (w6836:dbl)
              n1611 = local read "AO2"() -> (w6835:dbl)
              n1612 = Select(t=w6834, s=w6828, f=w6836) -> (s? t:f=w6833:dbl)
              n1613 = Select(t=w6835, s=w6828, f=w6834) -> (s? t:f=w6832:dbl)
              n1614 = flat-sequence {
                tunnel: w6833 -> [w6843]
                tunnel: w6832 -> [w6842]
                tunnel: w6831 -> [w6840]
                tunnel: [w6908] -> w6830
                tunnel: [w6907] -> w6827
                frame #0 {
                  w6846 = 10.0 ("y")
                  w6841 = 32767.0 ("y")
                  n1615 = Multiply(x=w6843, y=w6841) -> (x*y=w6849:dbl)
                  n1616 = Multiply(x=w6842, y=w6841) -> (x*y=w6847:dbl)
                  n1617 = Divide(x=w6849, y=w6846) -> (x/y=w6850:dbl)
                  n1618 = Divide(x=w6847, y=w6846) -> (x/y=w6848:dbl)
                  n1619 = To Word Integer(number=w6850) -> (16bit integer=w6844:i16)
                  n1620 = To Word Integer(number=w6848) -> (16bit integer=w6845:i16)
                  n1621 = xnode "Read/Write Control"("FPGA VI Reference In"=w6840, "AO1"=w6844, "AO2"=w6845) -> ()  [unwired: 1 in, 2 out]
                }
                frame #1 {
                  n1622 = Wait (ms)(milliseconds to wait="DAQ Delay (ms)") -> ()  [unwired: 1 out]
                }
                frame #2 {
                  n1623 = local read "Slow mean"() -> (w6908:dbl)
                  n1624 = local read "Sigma"() -> (w6907:dbl)
                }
              }
            }
            n1625 = Bundle("Begin (V)"="Begin (V)", w6819, w6825) -> (→"MCL Scan":cluster{"Begin (V)":dbl, dbl, dbl[]})  [unwired: 1 out]
            n1626 = Bundle("Begin (V)"="Begin (V)", w6819, w6818) -> (→"MCL Scan 2":cluster{"Begin (V)":dbl, dbl, dbl[]})  [unwired: 1 out]
          }
        }
      }
    }
    n1627 = local read "Stop All"() -> (w6708:bool)
    n1628 = node-c288() -> ()  [unwired: 2 out]
  }
  n1629 = timed-loop "Mouse control: trap position (AOM deflection), set confocal spot from image" {
    tunnel: [w6910] -> w137
    tunnel: w80 -> [w6909]
    timing: w19 -> [_]
    timing-out: [_] -> w18
    stop <- w6910 stop-if-true
    n1630 = node-c288() -> ()  [unwired: 2 out]
    n1631 = event shown="[0] \"Pane\": Mouse Down" {
      selector: _ -> [_ _]
      dyn-events: _ -> [_ _]
      timeout: _ -> [_ _]
      tunnel: w6909 -> [w6913 _]
      event #0 {
        n1632 = event-data() -> ("Time"=w6915:u32, "Coords"=w6914:T7, "Button"=w6916:u16)  [unwired: 6 out]
        n1633 = case shown="1" w6916 {
          tunnel: w6915 -> [_ _ w7012]
          tunnel: w6914 -> [_ w6946 w7010]
          tunnel: w6913 -> [_ _ w7008]
          frame #0 {
          }
          frame #1 {
            n1634 = property on="APD 1" class="ImageControl"() -> ("Displayed Image Position"=w6945:cluster{"Left":i32, "Top":i32})  [unwired: 2 in, 2 out]
            n1635 = property on="APD 1" class="ImageControl"() -> ("Displayed Image Size"=w6943:cluster{"Width":u32, "Height":u32})  [unwired: 2 in, 2 out]
            n1636 = property on="Detection Laser X" class="ImageControl"() -> ("Displayed Image Position"=w6942:cluster{"Left":i32, "Top":i32})  [unwired: 2 in, 2 out]
            n1637 = property on="Detection Laser X" class="ImageControl"() -> ("Displayed Image Size"=w6944:cluster{"Width":u32, "Height":u32})  [unwired: 2 in, 2 out]
            n1638 = property on="Detection Laser Y" class="ImageControl"() -> ("Displayed Image Position"=w6941:cluster{"Left":i32, "Top":i32})  [unwired: 2 in, 2 out]
            n1639 = property on="Detection Laser Y" class="ImageControl"() -> ("Displayed Image Size"=w6940:cluster{"Width":u32, "Height":u32})  [unwired: 2 in, 2 out]
            n1640 = Unbundle By Name(w6945) -> ("Left"=w6939:i32, "Top"=w6938:i32)
            n1641 = Unbundle By Name(w6943) -> ("Width"=w6937:u32, "Height"=w6936:u32)
            n1642 = Unbundle By Name(w6942) -> ("Left"=w6935:i32, "Top"=w6934:i32)
            n1643 = Unbundle By Name(w6944) -> ("Width"=w6933:u32, "Height"=w6932:u32)
            n1644 = Unbundle By Name(w6941) -> ("Left"=w6931:i32, "Top"=w6930:i32)
            n1645 = Unbundle By Name(w6940) -> ("Width"=w6929:u32, "Height"=w6928:u32)
            n1646 = Bundle("Left"=w6939, "Top"=w6938, "Width"=w6937, "Height"=w6936) -> (w6927:T42)  [unwired: 1 in]
            n1647 = Bundle("Left"=w6935, "Top"=w6934, "Width"=w6933, "Height"=w6932) -> (w6926:T42)  [unwired: 1 in]
            n1648 = Bundle("Left"=w6931, "Top"=w6930, "Width"=w6929, "Height"=w6928) -> (w6925:T42)  [unwired: 1 in]
            n1649 = Build Cluster Array(w6927, w6926, w6925) -> (w6924:T43)
            n1650 = for {
              tunnel: w6946 -> [w6957]
              tunnel: w6924 -> [w6958] mode=indexing
              shift-right: [w6955] -> w6922
              shift-left: TRUE -> [w6956]
              shift-right: [w6954] -> w6920
              shift-left: _ -> [w6950]
              shift-right: [w6953] -> w6919
              shift-left: _ -> [w6949]
              shift-right: [w6952] -> w6918
              shift-left: _ -> [w6948]
              shift-right: [w6951] -> w6917
              shift-left: _ -> [w6947]
              n1651 = case shown="True" w6956 {
                selector: w6956 -> [w6963 _]
                tunnel: w6958 -> [_ w6972]
                tunnel: w6957 -> [_ w6970]
                tunnel: [w6963 w6968] -> w6955
                tunnel: [w6962 w6967] -> w6954
                tunnel: [w6961 w6966] -> w6953
                tunnel: [w6960 w6965] -> w6952
                tunnel: [w6959 w6964] -> w6951
                tunnel: w6950 -> [w6962 _]
                tunnel: w6949 -> [w6961 _]
                tunnel: w6948 -> [w6960 _]
                tunnel: w6947 -> [w6959 _]
                frame #0 {
                }
                frame #1 {
                  n1652 = Unbundle(w6972) -> (w6971:T42)
                  n1653 = call "isclickinwindow.vi"("Image Param"=w6971, "Point32"=w6970) -> ("4 Y"=w6964:i32, "3 Height"=w6965:i32, "2 X"=w6966:i32, "1 Width"=w6967:i32, "In image?"=w6969:bool)  [unwired: 1 in]
                  n1654 = Not(x=w6969) -> (.not. x?=w6968:bool)
                }
              }
            }
            n1655 = Not(x=w6922) -> (.not. x?=w6921:bool)
            n1656 = case shown="True" w6921 {
              tunnel: w6919 -> [_ w6985]
              tunnel: w6917 -> [_ w6984]
              tunnel: w6920 -> [_ w6983]
              tunnel: w6918 -> [_ w6982]
              frame #0 {
              }
              frame #1 {
                w6978 = FALSE ("Get Point")
                n1657 = local read "Scan lines (y)"() -> (w6987:u64)
                n1658 = local read "Actual MCL Inc (V)"() -> (w6979:dbl)
                n1659 = local read "Scan steps (MCL)"() -> (w6986:u64)
                n1660 = Divide "Y Pix/step"(x=w6982, y=w6987) -> (x/y=w6994:dbl)
                n1661 = Divide "Y V/pix"(x=w6979, y=w6994) -> (x/y=w6993:dbl)
                n1662 = Divide "Y half step offset"(x=w6979, y=2.0) -> (x/y=w6995:dbl)
                n1663 = Divide "X pix/step"(x=w6983, y=w6986) -> (x/y=w6992:dbl)
                n1664 = Negate(x=w6995) -> (-x=w6996:dbl)
                n1665 = local read "Initial Y"() -> (w7002:dbl)
                n1666 = Multiply(x=w6984, y=w6993) -> (x*y=w7003:dbl)
                n1667 = Divide "X half step offset"(x=w6979, y=2.0) -> (x/y=w6989:dbl)
                n1668 = Divide "X V/pix"(x=w6979, y=w6992) -> (x/y=w6991:dbl)
                n1669 = Multiply(x=w6979, y=w6986) -> (x*y=w6998:dbl)
                n1670 = Compound Arithmetic op=ADD(w6996, w7003, w7002) -> (w6980:dbl)
                "Pointer Y (V)" <- w6980
                n1671 = Multiply(x=w6991, y=w6985) -> (x*y=w7000:dbl)
                n1672 = Negate(x=w6989) -> (-x=w6988:dbl)
                n1673 = local read "Initial X"() -> (w7001:dbl)
                n1674 = Negate(x=w7000) -> (-x=w6999:dbl)
                n1675 = Compound Arithmetic op=ADD(w6988, w6998, w7001, w6999) -> (w6981:dbl)
                "Pointer X (V)" <- w6981
                n1676 = Or(x="Set X Only", y="Set Confocal Spot (X-Y)") -> (x .or. y?=w6974:bool)
                n1677 = Or(x="Set Confocal Spot (X-Y)", y="Set Y Only") -> (x .or. y?=w6973:bool)
                n1678 = case shown="True" w6974 {
                  tunnel: w6981 -> [_ w7004]
                  frame #0 {
                  }
                  frame #1 {
                    n1679 = property on="AO2" class="Slide (strict)"("Val(Sgnl)"=w7004) -> ()  [unwired: 2 in, 2 out]
                  }
                }
                n1680 = case shown="True" w6973 {
                  tunnel: w6980 -> [_ w7005]
                  frame #0 {
                  }
                  frame #1 {
                    n1681 = property on="AO1" class="Slide (strict)"("Val(Sgnl)"=w7005) -> ()  [unwired: 2 in, 2 out]
                  }
                }
                n1682 = local write "Set Confocal Spot (X-Y)"(w6978) -> ()
                n1683 = local write "Set X Only"(w6978) -> ()
                n1684 = local write "Set Y Only"(w6978) -> ()
              }
            }
          }
          frame #2 {
            n1685 = local read "BD 2 Frequency 1 (MHz)"() -> (w7006:dbl)
            n1686 = local read "BD 1 Frequency 1 (MHz)"() -> (w7007:dbl)
            n1687 = local write "Manipulating Trap"(TRUE ("Manipulating Trap")) -> ()
            n1688 = local write "Coords"(T7 {"Horizontal"=0, "Vertical"=0} ("Coords")) -> ()
            n1689 = while {
              tunnel: w7012 -> [w7017]
              tunnel: w7010 -> [w7016]
              tunnel: w7008 -> [w7015]
              tunnel: w7007 -> [w7014]
              tunnel: w7006 -> [w7013]
              stop <- w7018 stop-if-true
              n1690 = event shown="[0] \"Pane\": Mouse Move" {
                selector: _ -> [_ _]
                dyn-events: _ -> [_ _]
                timeout: _ -> [_ _]
                tunnel: ["Force Manip Abort" w7082] -> w7018
                tunnel: w7017 -> [w7025 _]
                tunnel: w7016 -> [w7023 _]
                tunnel: w7015 -> [w7022 _]
                tunnel: w7014 -> [w7021 _]
                tunnel: w7013 -> [w7020 _]
                event #0 {
                  n1691 = event-data() -> ("Time"=w7026:u32, "Coords"=w7027:T7)  [unwired: 3 out]
                  n1692 = Less?(x=w7026, y=w7025) -> (x < y?=w7024:bool)
                  n1693 = case "Makes sure old motion events prior to mouse click aren't used" shown="False" w7024 {
                    tunnel: w7027 -> [w7069 _]
                    tunnel: w7023 -> [w7070 _]
                    tunnel: w7022 -> [w7047 _]
                    tunnel: w7021 -> [w7043 _]
                    tunnel: w7020 -> [w7042 _]
                    frame #0 {
                      n1694 = Subtract(x=w7069, y=w7070) -> (x-y=w7068:T7)
                      "Coords" <- w7068
                      n1695 = local read "Y RF Frequency Limits (MHz)"() -> (w7028:T12)
                      n1696 = To Double Precision Float(number=w7068) -> (double precision float=w7067:cluster{"Horizontal":dbl, "Vertical":dbl})
                      n1697 = Multiply(x=cluster{"Horizontal":dbl, "Vertical":dbl} {"Horizontal"=-1.0, "Vertical"=1.0}, y="Manipulation Scaling") -> (x*y=w7063:cluster{"Horizontal":dbl, "Vertical":dbl})
                      n1698 = Multiply(x=w7067, y=w7063) -> (x*y=w7065:cluster{"Horizontal":dbl, "Vertical":dbl})
                      n1699 = local read "X RF Frequency Limits (MHz)"() -> (w7029:T12)
                      n1700 = Unbundle By Name(w7065) -> ("Horizontal"=w7060:dbl, "Vertical"=w7064:dbl)
                      n1701 = Boolean To (0,1)(Boolean="Manip. X?") -> (0, 1=w7058:i16)
                      n1702 = Unbundle By Name(w7028) -> ("Maximum"=w7031:dbl, "Minimum"=w7030:dbl)
                      n1703 = Boolean To (0,1)(Boolean="Manip. Y?") -> (0, 1=w7055:i16)
                      n1704 = Multiply(x=w7064, y=w7055) -> (x*y=w7057:dbl)
                      n1705 = Multiply(x=w7058, y=w7060) -> (x*y=w7061:dbl)
                      n1706 = local read "BD 1 Frequency 2 (MHz)"() -> (w7045:dbl)
                      n1707 = Unbundle By Name(w7029) -> ("Maximum"=w7033:dbl, "Minimum"=w7032:dbl)
                      n1708 = local read "BD 2 Frequency 2 (MHz)"() -> (w7044:dbl)
                      n1709 = Add(x=w7042, y=w7057) -> (x+y=w7035:dbl)
                      n1710 = Add(x=w7043, y=w7061) -> (x+y=w7037:dbl)
                      n1711 = In Range and Coerce(upper limit=w7033, x=w7037, lower limit=w7032) -> (coerced(x)=w7036:dbl)  [unwired: 1 out]
                      n1712 = In Range and Coerce(upper limit=w7031, x=w7035, lower limit=w7030) -> (coerced(x)=w7034:dbl)  [unwired: 1 out]
                      n1713 = Subtract(x=w7036, y=w7045) -> (x-y=w7054:dbl)
                      n1714 = Subtract(x=w7034, y=w7044) -> (x-y=w7053:dbl)
                      n1715 = Square(x=w7054) -> (x^2=w7052:dbl)
                      n1716 = Square(x=w7053) -> (x^2=w7051:dbl)
                      n1717 = Add(x=w7052, y=w7051) -> (x+y=w7050:dbl)
                      n1718 = Square Root(x=w7050) -> (sqrt(x)=w7046:dbl)
                      n1719 = In Range and Coerce(upper limit="Limit Max (MHz)", x=w7046, lower limit="Limit Min (MHz)") -> (In Range?=w7039:bool)  [unwired: 1 out]
                      n1720 = Not(x="Limits Enable") -> (.not. x?=w7038:bool)
                      n1721 = Or(x=w7039, y=w7038) -> (x .or. y?=w7040:bool)
                      n1722 = case shown="True" w7040 {
                        tunnel: w7047 -> [_ w7080]
                        tunnel: w7046 -> [_ w7071]
                        tunnel: w7036 -> [_ w7078]
                        tunnel: w7045 -> [_ w7077]
                        tunnel: w7034 -> [_ w7076]
                        tunnel: w7044 -> [_ w7075]
                        tunnel: w7029 -> [_ w7073]
                        tunnel: w7028 -> [_ w7072]
                        frame #0 {
                        }
                        frame #1 {
                          n1723 = local read "BD 1 Frequency 3 (MHz)"() -> (w7079:dbl)
                          n1724 = local read "BD 2 Frequency 3 (MHz)"() -> (w7074:dbl)
                          n1725 = local write "Trap Delta (MHz)"(w7071) -> ()
                          n1726 = property on="Initial delta (MHz)" class="DigNum (strict)"("Val(Sgnl)"=w7071) -> ()  [unwired: 2 in, 2 out]
                          n1727 = call "set RF board frequency - interlace.vi"("Board 2 Frequency Limits"=w7072, "Board 1 Frequency Limits"=w7073, "FPGA VI Reference In"=w7080, "Board 2 Frequency 3 (MHz)"=w7074, "Board 1 Frequency 3 (MHz)"=w7079, "Board 2 Frequency 2 (MHz)"=w7075, "Board 2 Frequency 1 (MHz)"=w7076, "Board 1 Frequency 2 (MHz)"=w7077, "Board 1 Frequency 1  (MHz)"=w7078) -> ()  [unwired: 1 in, 2 out]
                          n1728 = local write "BD 2 Frequency 1 (MHz)"(w7076) -> ()
                          n1729 = local write "BD 1 Frequency 1 (MHz)"(w7078) -> ()
                        }
                      }
                    }
                    frame #1 {
                    }
                  }
                }
                event #1 {
                  n1730 = event-data() -> ("Button"=w7081:u16)  [unwired: 8 out]
                  n1731 = case shown="3" w7081 {
                    tunnel: [FALSE TRUE] -> w7082
                    frame #0 {
                    }
                    frame #1 {
                      n1732 = local write "Manipulating Trap"(FALSE ("Manipulating Trap")) -> ()
                    }
                  }
                }
              }
            }
          }
        }
      }
      event #1 {
        n1733 = event-data() -> ()  [unwired: 6 out]
      }
    }
    n1734 = local read "Stop All"() -> (w6910:bool)
    n1735 = node-c288() -> ()  [unwired: 2 out]
  }
  n1736 = timed-loop "Stage Control and Stage + Action Control" {
    shift-right: [w7097] -> w61
    shift-left: w63 -> [w7114]
    shift-right: [w7096] -> w60
    shift-left: w62 -> [w7113]
    tunnel: w59 -> [w7098]
    timing: w17 -> [_]
    timing-out: [_] -> w16
    shift-right: ["Dump Beads"] -> _
    shift-left: FALSE ("Dump Beads") -> [w7089]
    stop <- w7115 stop-if-true
    (unwired) T12 {"Minimum"=0.0, "Maximum"=0.0, "Increment"=0.0}  # Y Limits
    (unwired) T12 {"Minimum"=0.0, "Maximum"=0.0, "Increment"=0.0}  # X Limits
    n1737 = node-c288() -> ()  [unwired: 2 out]
    n1738 = local read "Stop All"() -> (w7115:bool)
    n1739 = call "Read Stage Position.vi"("error in"=w7113, "VISA resource name in"=w7114) -> ("Current Position"=w7099:cluster{dbl, dbl, dbl}, "error out"=w7106:errorcluster, "VISA resource name out"=w7107:refnum<visa-resource-name>)  [unwired: 1 out]
    "Current Stage  Position" <- w7099
    n1740 = Or(x="Move to Position 3", y="Data Acq. Spot") -> (x .or. y?=w7092:bool)
    n1741 = Or(x="Lower Cap.", y=w7089) -> (x .or. y?=w7088:bool)
    n1742 = Or(x="Move to Position 1", y="Upper Cap.") -> (x .or. y?=w7095:bool)
    n1743 = Compound Arithmetic op=OR(w7088, "Move to Position 2") -> (w7094:bool)
    n1744 = Or(x="Dump Beads", y="Move to Position 4") -> (x .or. y?=w7091:bool)
    n1745 = Build Array(w7095, w7094, w7092, w7091) -> (w7105:bool[])
    n1746 = Or Array Elements(Boolean array=w7105) -> (logical OR=w7108:bool)
    n1747 = case shown="True" w7108 {
      tunnel: w7107 -> [w7160 w7168]
      tunnel: w7106 -> [w7159 w7167]
      tunnel: [w7160 w7171] -> w7104
      tunnel: [w7159 w7170] -> w7103
      tunnel: w7105 -> [_ w7169]
      tunnel: "Dump Beads" -> [_ w7164]
      tunnel: w7088 -> [_ w7163]
      tunnel: "Upper Cap." -> [_ w7162]
      tunnel: "Data Acq. Spot" -> [_ w7161]
      frame #0 {
      }
      frame #1 {
        n1748 = flat-sequence {
          tunnel: w7169 -> [w7179]
          tunnel: w7168 -> [w7174]
          tunnel: w7167 -> [w7173]
          tunnel: [w7182] -> w7166
          tunnel: [w7181] -> w7165
          tunnel: [w7188] -> w7170
          tunnel: [w7189] -> w7171
          tunnel: w7166 -> [w7189]
          tunnel: w7165 -> [w7188]
          tunnel: w7164 -> [w7186]
          tunnel: w7163 -> [w7185]
          tunnel: w7162 -> [w7184]
          tunnel: w7161 -> [w7183]
          frame #0 {
            n1749 = Boolean Array To Number(Boolean array=w7179) -> (number=w7180:u32)
            n1750 = local read "Saved Stage Positions"() -> (w7178:T4)
            n1751 = Logarithm Base 2(1:w7180) -> (0:w7176:dbl)
            n1752 = Cluster To Array(cluster=w7178) -> (array=w7177:cluster{dbl, dbl, dbl}[])
            n1753 = Index Array(array=w7177, index=w7176) -> (element=w7175:cluster{dbl, dbl, dbl})
            n1754 = call "Set Stage Position.vi"("Position"=w7175, "error in"=w7173, "VISA resource name in"=w7174) -> ("error out"=w7181:errorcluster, "VISA resource name out"=w7182:refnum<visa-resource-name>)  [unwired: 1 out]
            "Stage Moving" <- TRUE ("Stage Moving")
          }
          frame #1 {
            n1755 = local write "Stage Moving"(FALSE ("Stage Moving")) -> ()
            n1756 = case shown="True" w7186 {
              frame #0 {
              }
              frame #1 {
                w7204 = FALSE ("Value (Signaling)")
                n1757 = property on="Green Laser ON/Interlacing" class="Bool (strict)"("Val(Sgnl)"=w7204) -> ()  [unwired: 2 in, 2 out]
                n1758 = property on="Trap 1 (ON/OFF)" class="Bool (strict)"("Val(Sgnl)"=w7204) -> ()  [unwired: 2 in, 2 out]
                n1759 = property on="Trap 2 (ON/OFF)" class="Bool (strict)"("Val(Sgnl)"=w7204) -> ()  [unwired: 2 in, 2 out]
              }
            }
            n1760 = call <vilib>:"Beep.vi"() -> ()  [unwired: 3 in, 9 out]
            n1761 = case shown="True" w7184 {
              selector: w7184 -> [_ w7202]
              frame #0 {
              }
              frame #1 {
                n1762 = property on="Trap 2 (ON/OFF)" class="Bool (strict)"("Val(Sgnl)"=w7202) -> ()  [unwired: 2 in, 2 out]
              }
            }
            n1763 = case shown="True" w7183 {
              selector: w7183 -> [_ w7190]
              frame #0 {
              }
              frame #1 {
                n1764 = flat-sequence {
                  tunnel: w7190 -> [w7191]
                  frame #0 {
                    n1765 = property on="Save Calibration" class="Bool (strict)"("Val(Sgnl)"=w7191) -> ()  [unwired: 2 in, 2 out]
                  }
                  frame #1 {
                    n1766 = Wait (ms)(milliseconds to wait=u32 2000) -> ()  [unwired: 1 out]
                  }
                  frame #2 {
                    n1767 = while {
                      stop <- w7193 stop-if-true
                      n1768 = local read "Saving..."() -> (w7194:bool)
                      n1769 = Wait (ms)(milliseconds to wait=u32 1000) -> ()  [unwired: 1 out]
                      n1770 = Not(x=w7194) -> (.not. x?=w7193:bool)
                    }
                  }
                  frame #3 {
                    n1771 = Multiply(x="Cal read wait (s)", y=u32 1000 ("milliseconds to wait")) -> (x*y=w7197:u32)
                    n1772 = Wait (ms)(milliseconds to wait=w7197) -> ()  [unwired: 1 out]
                  }
                  frame #4 {
                    n1773 = property on="Read Cal" class="Bool (strict)"("Val(Sgnl)"=TRUE ("Value (Signaling)")) -> ()  [unwired: 2 in, 2 out]
                  }
                  frame #5 {
                    n1774 = Wait (ms)(milliseconds to wait=u32 2000) -> ()  [unwired: 1 out]
                  }
                  frame #6 {
                    n1775 = property on="Fish for Tether" class="Bool (strict)"("Val(Sgnl)"=TRUE ("Value (Signaling)")) -> ()  [unwired: 2 in, 2 out]
                  }
                }
              }
            }
            n1776 = case shown="True" w7185 {
              selector: w7185 -> [_ w7203]
              frame #0 {
              }
              frame #1 {
                n1777 = property on="Trap 1 (ON/OFF)" class="Bool (strict)"("Val(Sgnl)"=w7203) -> ()  [unwired: 2 in, 2 out]
              }
            }
          }
        }
      }
    }
    n1778 = Or(x="+z", y="-z") -> (x .or. y?=w7102:bool)
    n1779 = case shown="True" w7102 {
      tunnel: w7104 -> [w7119 w7123]
      tunnel: w7103 -> [w7118 w7122]
      tunnel: [w7119 w7126] -> w7097
      tunnel: [w7118 w7125] -> w7096
      tunnel: "+z" -> [_ w7129]
      tunnel: "-z" -> [_ w7128]
      tunnel: w7099 -> [_ w7127]
      tunnel: w7098 -> [_ w7124]
      frame #0 {
      }
      frame #1 {
        n1780 = flat-sequence {
          tunnel: w7129 -> [w7155]
          tunnel: w7128 -> [w7154]
          tunnel: w7127 -> [w7150]
          tunnel: w7124 -> [w7135]
          tunnel: w7123 -> [w7132]
          tunnel: w7122 -> [w7131]
          tunnel: [w7142] -> w7121
          tunnel: [w7141] -> w7120
          tunnel: [w7157] -> w7125
          tunnel: [w7158] -> w7126
          tunnel: w7121 -> [w7158]
          tunnel: w7120 -> [w7157]
          frame #0 {
            n1781 = Boolean To (0,1)(Boolean=w7155) -> (0, 1=w7153:i16)
            n1782 = Boolean To (0,1)(Boolean=w7154) -> (0, 1=w7152:i16)
            n1783 = Unbundle(w7150) -> (w7149:dbl, w7148:dbl, w7144:dbl)
            n1784 = Divide(x="z nudge increment (um)", y=1000.0) -> (x/y=w7138:dbl)
            n1785 = Multiply(x=w7153, y=w7138) -> (x*y=w7146:dbl)
            n1786 = Multiply(x=w7152, y=w7138) -> (x*y=w7151:dbl)
            n1787 = Negate(x=w7151) -> (-x=w7147:dbl)
            n1788 = Add(x=w7146, y=w7147) -> (x+y=w7145:dbl)
            n1789 = local write "Stage Moving"(TRUE ("Stage Moving")) -> ()
            n1790 = Add(x=w7145, y=w7144) -> (x+y=w7137:dbl)
            n1791 = Unbundle(w7135) -> ("Minimum"=w7134:dbl, "Maximum"=w7133:dbl)  [unwired: 1 out]
            n1792 = In Range and Coerce(upper limit=w7133, x=w7137, lower limit=w7134) -> (coerced(x)=w7136:dbl)  [unwired: 1 out]
            n1793 = Bundle(cluster=w7150, w7149, w7148, w7136) -> (w7143:cluster{dbl, dbl, dbl})
            n1794 = call "Set Stage Position.vi"("Position"=w7143, "error in"=w7131, "VISA resource name in"=w7132) -> ("error out"=w7141:errorcluster, "VISA resource name out"=w7142:refnum<visa-resource-name>)  [unwired: 1 out]
          }
          frame #1 {
            n1795 = local write "Stage Moving"(FALSE ("Stage Moving")) -> ()
          }
        }
      }
    }
    n1796 = node-c288() -> ()  [unwired: 2 out]
  }
  n1797 = for "Create Greyscale map" {
    N: 256 -> [_]
    tunnel: [w7206] -> w190 mode=indexing
    i -> [w7209]
    n1798 = To Unsigned Byte Integer(number=w7209) -> (unsigned 8bit integer=w7205:u8)
    n1799 = Join Numbers(hi=w7205, lo=w7205) -> ((hi.lo)=w7208:u16)
    n1800 = Join Numbers(hi=w7205, lo=w7205) -> ((hi.lo)=w7207:u16)
    n1801 = Join Numbers(hi=w7208, lo=w7207) -> ((hi.lo)=w7206:u32)
  }
  n1802 = node-c288(w10) -> ()  [unwired: 1 out]
  n1803 = node-c288(w14) -> ()  [unwired: 1 out]
  n1804 = node-c288(w18) -> ()  [unwired: 1 out]
  n1805 = node-c288(w16) -> ()  [unwired: 1 out]
  n1806 = node-c288(w12) -> ()  [unwired: 1 out]
  n1807 = VISA Close(VISA resource name=w61, error in (no error)=w60) -> (error out=w65:errorcluster)
  n1808 = call <vilib>:"Simple Error Handler.vi"("error in (no error)"=w65) -> ()  [unwired: 1 in, 8 out]
  n1809 = node-c288(w129) -> ()  [unwired: 1 out]
  n1810 = flat-sequence {
    tunnel: w231 -> [w7213]
    tunnel: w233 -> [w7214]
    tunnel: [w7212] -> w211
    tunnel: [w7211] -> w210
    tunnel: w186 -> [_]
    tunnel: w184 -> [_]
    tunnel: w137 -> [_]
    tunnel: w20 -> [_]
    tunnel: w211 -> [w7272]
    tunnel: w210 -> [w7273]
    frame #0 {
      w7210 = FALSE ("AI to FIFO")
      n1811 = xnode "Read/Write Control"("FPGA VI Reference In"=w7214, "error in"=w7213, "AI to FIFO"=w7210, "APD to FIFO"=w7210) -> ("FPGA VI Reference Out"=w7212:T15, "error out"=w7211:errorcluster)
    }
    frame #1 {
      n1812 = xnode "Close FPGA VI Reference"("FPGA VI Reference In"=w7272, "error in"=w7273) -> ("error out"=→"error out":errorcluster)
    }
  }
